vi "Beampointing_Multi_Pico2.vi"() -> ()   [LabVIEW 2013]
uses:
  GUI_Template/GUI_master/tcp_new_data_event.ctl
  GUI_Template/GUI_master/tcp new data cluster.ctl
  Ctrs/beam detection.ctl
  GUI_Beampointing_single_TRA/Ctrs/move.ctl
  <vilib>/Utility/file.llb/Read From Spreadsheet File (string).vi
  <userlib>/_OpenG.lib/array/array.llb/Filter 1D Array with Scalar (String)__ogtk.vi
  <userlib>/_OpenG.lib/array/array.llb/Filter 1D Array (String)__ogtk.vi
  <vilib>/Utility/file.llb/Write To Spreadsheet File (string).vi
  <vilib>/Analysis/NI_AALBase.lvlib
panel:
  out "x-y*floor(x/y)":dbl
  out "error out":errorcluster
  out "config path":string
  out "Array 3":bool[](array[boolean])
  out "Array 2":u16[](array[numeric])
  out "Array":u16[](array[numeric])
  out "Moving Y":string
  out "Moving X":string
  out "particles":T1(array[cluster])
  out "millisecond timer value":u32
  out "appended path":path
  out "millisecond timer 2":u32
  in  "GUIdevice 98":string="PicoPad4"
  in  "Position.Axis 111::98":dbl=77.0 caption="Motor Axis 1" min=-30000.0 max=30000.0 format="%#_6f"
  in  "Position.Axis 112::98":dbl=77.0 caption="Motor Axis 1" min=-20000.0 max=20000.0 format="%#_6f"
  in  "Position.Axis 113::98":dbl=77.0 caption="Motor Axis 1" min=-20000.0 max=20000.0 format="%#_6f"
  in  "Position.Axis 121::98":dbl=77.0 caption="Motor Axis 1" min=-999999.0 max=999999.0 format="%#_6f"
  in  "Position.Axis 122::98":dbl=77.0 caption="Motor Axis 1" min=-999999.0 max=999999.0 format="%#_6f"
  in  "Position.Axis 123::98":dbl=77.0 caption="Motor Axis 1" min=-999999.0 max=999999.0 format="%#_6f"
  in  "Position.Axis 131::98":dbl=77.0 caption="Motor Axis 1" min=-999999.0 max=999999.0 format="%#_6f"
  in  "Position.Axis 132::98":dbl=77.0 caption="Motor Axis 1" min=-999999.0 max=999999.0 format="%#_6f"
  in  "Position.Axis 133::98":dbl=77.0 caption="Motor Axis 1" min=-999999.0 max=999999.0 format="%#_6f"
  in  "Position.Axis 141::98":dbl=77.0 caption="Motor Axis 1" min=-999999.0 max=999999.0 format="%#_6f"
  in  "Position.Axis 142::98":dbl=77.0 caption="Motor Axis 1" min=-999999.0 max=999999.0 format="%#_6f"
  in  "Position.Axis 143::98":dbl=77.0 caption="Motor Axis 1" min=-999999.0 max=999999.0 format="%#_6f"
  in  "Position.Axis 211::98":dbl=77.0 caption="Motor Axis 1" min=-999999.0 max=999999.0 format="%#_6f"
  in  "Position.Axis 212::98":dbl=77.0 caption="Motor Axis 1" min=-999999.0 max=999999.0 format="%#_6f"
  in  "Position.Axis 213::98":dbl=77.0 caption="Motor Axis 1" min=-999999.0 max=999999.0 format="%#_6f"
  in  "Position.Axis 221::98":dbl=77.0 caption="Motor Axis 1" min=-999999.0 max=999999.0 format="%#_6f"
  in  "Position.Axis 222::98":dbl=77.0 caption="Motor Axis 1" min=-999999.0 max=999999.0 format="%#_6f"
  in  "Position.Axis 223::98":dbl=77.0 caption="Motor Axis 1" min=-999999.0 max=999999.0 format="%#_6f"
  in  "Position.Axis 231::98":dbl=77.0 caption="Motor Axis 1" min=-999999.0 max=999999.0 format="%#_6f"
  in  "Position.Axis 232::98":dbl=77.0 caption="Motor Axis 1" min=-999999.0 max=999999.0 format="%#_6f"
  in  "Position.Axis 233::98":dbl=77.0 caption="Motor Axis 1" min=-999999.0 max=999999.0 format="%#_6f"
  in  "Position.Axis 241::98":dbl=77.0 caption="Motor Axis 1" min=-999999.0 max=999999.0 format="%#_6f"
  in  "Position.Axis 242::98":dbl=77.0 caption="Motor Axis 1" min=-999999.0 max=999999.0 format="%#_6f"
  in  "Position.Axis 243::98":dbl=77.0 caption="Motor Axis 1" min=-999999.0 max=999999.0 format="%#_6f"
  in  "Position.Axis 311::98":dbl=77.0 caption="Motor Axis 1" min=-999999.0 max=999999.0 format="%#_6f"
  in  "Position.Axis 312::98":dbl=77.0 caption="Motor Axis 1" min=-999999.0 max=999999.0 format="%#_6f"
  in  "Position.Axis 313::98":dbl=77.0 caption="Motor Axis 1" min=-999999.0 max=999999.0 format="%#_6f"
  in  "Position.Axis 321::98":dbl=77.0 caption="Motor Axis 1" min=-999999.0 max=999999.0 format="%#_6f"
  in  "Position.Axis 322::98":dbl=77.0 caption="Motor Axis 1" min=-999999.0 max=999999.0 format="%#_6f"
  in  "Position.Axis 323::98":dbl=77.0 caption="Motor Axis 1" min=-999999.0 max=999999.0 format="%#_6f"
  in  "Position.Axis 331::98":dbl=77.0 caption="Motor Axis 1" min=-999999.0 max=999999.0 format="%#_6f"
  in  "Position.Axis 332::98":dbl=77.0 caption="Motor Axis 1" min=-999999.0 max=999999.0 format="%#_6f"
  in  "Position.Axis 333::98":dbl=77.0 caption="Motor Axis 1" min=-999999.0 max=999999.0 format="%#_6f"
  in  "Position.Axis 341::98":dbl=77.0 caption="Motor Axis 1" min=-999999.0 max=999999.0 format="%#_6f"
  in  "Position.Axis 342::98":dbl=77.0 caption="Motor Axis 1" min=-999999.0 max=999999.0 format="%#_6f"
  in  "Position.Axis 343::98":dbl=77.0 caption="Motor Axis 1" min=-999999.0 max=999999.0 format="%#_6f"
  in  "Position.Axis 411::98":dbl=77.0 caption="Motor Axis 1" min=-999999.0 max=999999.0 format="%#_6f"
  in  "Position.Axis 412::98":dbl=77.0 caption="Motor Axis 1" min=-999999.0 max=999999.0 format="%#_6f"
  in  "Position.Axis 413::98":dbl=77.0 caption="Motor Axis 1" min=-999999.0 max=999999.0 format="%#_6f"
  in  "Position.Axis 421::98":dbl=77.0 caption="Motor Axis 1" min=-999999.0 max=999999.0 format="%#_6f"
  in  "Position.Axis 422::98":dbl=77.0 caption="Motor Axis 1" min=-999999.0 max=999999.0 format="%#_6f"
  in  "Position.Axis 423::98":dbl=77.0 caption="Motor Axis 1" min=-999999.0 max=999999.0 format="%#_6f"
  in  "Position.Axis 431::98":dbl=77.0 caption="Motor Axis 1" min=-999999.0 max=999999.0 format="%#_6f"
  in  "Position.Axis 432::98":dbl=77.0 caption="Motor Axis 1" min=-999999.0 max=999999.0 format="%#_6f"
  in  "Position.Axis 433::98":dbl=77.0 caption="Motor Axis 1" min=-999999.0 max=999999.0 format="%#_6f"
  in  "Position.Axis 441::98":dbl=77.0 caption="Motor Axis 1" min=-999999.0 max=999999.0 format="%#_6f"
  in  "Position.Axis 442::98":dbl=77.0 caption="Motor Axis 1" min=-999999.0 max=999999.0 format="%#_6f"
  in  "Position.Axis 443::98":dbl=77.0 caption="Motor Axis 1" min=-999999.0 max=999999.0 format="%#_6f"
  in  "Position.Axis 511::98":dbl=77.0 caption="Motor Axis 1" min=-999999.0 max=999999.0 format="%#_6f"
  in  "Position.Axis 512::98":dbl=77.0 caption="Motor Axis 1" min=-999999.0 max=999999.0 format="%#_6f"
  in  "Position.Axis 513::98":dbl=77.0 caption="Motor Axis 1" min=-999999.0 max=999999.0 format="%#_6f"
  in  "Position.Axis 521::98":dbl=77.0 caption="Motor Axis 1" min=-999999.0 max=999999.0 format="%#_6f"
  in  "Position.Axis 522::98":dbl=77.0 caption="Motor Axis 1" min=-999999.0 max=999999.0 format="%#_6f"
  in  "Position.Axis 523::98":dbl=77.0 caption="Motor Axis 1" min=-999999.0 max=999999.0 format="%#_6f"
  in  "Position.Axis 531::98":dbl=77.0 caption="Motor Axis 1" min=-999999.0 max=999999.0 format="%#_6f"
  in  "Position.Axis 532::98":dbl=77.0 caption="Motor Axis 1" min=-999999.0 max=999999.0 format="%#_6f"
  in  "Position.Axis 533::98":dbl=77.0 caption="Motor Axis 1" min=-999999.0 max=999999.0 format="%#_6f"
  in  "Position.Axis 541::98":dbl=77.0 caption="Motor Axis 1" min=-999999.0 max=999999.0 format="%#_6f"
  in  "Position.Axis 542::98":dbl=77.0 caption="Motor Axis 1" min=-999999.0 max=999999.0 format="%#_6f"
  in  "Position.Axis 543::98":dbl=77.0 caption="Motor Axis 1" min=-999999.0 max=999999.0 format="%#_6f"
  in  "Numeric":dbl
  out "Current State":string
  in  "output cluster 2":T5 {"detection para"."smal para"."Measurement Parameter" items=["Center of Mass X", "Center of Mass Y", "First Pixel X", "First Pixel Y", "Bounding Rect Left", "Bounding Rect Top", "Bounding Rect Right", "Bounding Rect Bottom", "Max Feret Diameter Start X", "Max Feret Diameter Start Y", "Max Feret Diameter End X", "Max Feret Diameter End Y", "Max Horiz. Segment Length Left", "Max Horiz. Segment Length Right", "Max Horiz. Segment Length Row", "-", "Bounding Rect Width", "Bounding Rect Height", "Bounding Rect Diagonal", "Perimeter", "Convex Hull Perimeter", "Holes' Perimeter", "Max Feret Diameter", "Equivalent Ellipse Major Axis", "Equivalent Ellipse Minor Axis", "Equivalent Ellipse Minor Axis (Feret)", "Equivalent Rect Long Side", "Equivalent Rect Short Side", "Equivalent Rect Diagonal", "Equivalent Rect Short Side (Feret)", "Average Horiz. Segment Length", "Average Vert. Segment Length", "Hydraulic Radius", "Waddel Disk Diameter", "-", "Area", "Holes' Area", "Particle & Holes' Area", "Convex Hull Area", "Image Area", "-", "Number of Holes", "Number of Horiz. Segments", "Number of Vert. Segments", "-", "Orientation", "Max Feret Diameter Orientation", "-", "% Area/Image Area", "% Area/(Particle & Holes' Area)", "Ratio of Equivalent Ellipse Axes", "Ratio of Equivalent Rect Sides", "-", "Elongation Factor", "Compactness Factor", "Heywood Circularity Factor", "Type Factor", "-", "Sum X", "Sum Y", "Sum XX", "Sum XY", "Sum YY", "Sum XXX", "Sum XXY", "Sum XYY", "Sum YYY", "-", "Moment of Inertia XX", "Moment of Inertia XY", "Moment of Inertia YY", "Moment of Inertia XXX", "Moment of Inertia XXY", "Moment of Inertia XYY", "Moment of Inertia YYY", "Norm. Moment of Inertia XX", "Norm. Moment of Inertia XY", "Norm. Moment of Inertia YY", "Norm. Moment of Inertia XXX", "Norm. Moment of Inertia XXY", "Norm. Moment of Inertia XYY", "Norm. Moment of Inertia YYY", "Hu Moment 1", "Hu Moment 2", "Hu Moment 3", "Hu Moment 4", "Hu Moment 5", "Hu Moment 6", "Hu Moment 7"]; "detection para"."smal para"."Range Lower Value" format="%.2f"; "detection para"."smal para"."Range Upper Value" format="%.2f"; "detection para"."detection method" items=["clustering", "entropy", "metric", "moments", "inter-class variance"]; "detection para"."Filter" items=["No Filter", "Median Filter", "Low Pass Filter"]}
  out "CCDs":string[](array[string])
  in  "GUIdevice 12":string
  in  "GUIdevice 11":string
  in  "GUIdevice 10":string
  in  "GUIdevice 9":string
  out "error out 2":errorcluster
  in  "active cams":string[](array[string])
  in  "Motor Y":dbl[][](array[numeric])
  in  "Motor X":dbl[][](array[numeric])
  out "Names":string[](array[string])
  in  "Offset X stats":dbl[][](array[numeric])
  in  "Offset Y stats":dbl[][](array[numeric])
  out "Box":T6(array[cluster])
  in  "Tab Control 2":enum32{"Config ", "Main", "History"}(tab)=enum."Main"
  out "Waveform Chart":u32(graph)
  in  "associated motors":T7
  out "Cameras":T8
  out "Status":cluster{i32, i32, "Centroid X":dbl[][]}(graph)
  out "image::9":T9(plugin-control) caption="L8_M10Leak"
  out "image::6":T9(plugin-control) caption="L5_TREXPass2"
  in  "Exposure:12":dbl=0.095 min=0.0001 max=1.0 format="%#_6f"
  in  "Triggerdelay::12":dbl=0.003 min=0.0 max=0.09 format="%#_6f"
  in  "Exposure::11":dbl=0.095 min=0.0001 max=1.0 format="%#_6f"
  in  "Triggerdelay::11":dbl=0.003 min=0.0 max=0.09 format="%#_6f"
  in  "Exposure::10":dbl=0.095 min=0.0001 max=1.0 format="%#_6f"
  in  "Triggerdelay::10":dbl=0.003 min=0.0 max=0.09 format="%#_6f"
  in  "Exposure::9":dbl=0.095 min=0.0001 max=1.0 format="%#_6f"
  in  "Triggerdelay::9":dbl=0.003 min=0.0 max=0.09 format="%#_6f"
  in  "Trigger::9":bool
  in  "Trigger::10":bool caption="Trigger:10"
  in  "Trigger::11":bool
  in  "Trigger::12":bool
  in  "Target.Y::9":dbl=45.0 caption="T9y" min=0.0 max=2000.0 format="%#_6f"
  in  "Target.X::9":dbl=47.0 caption="Tx9" min=0.0 max=2000.0 format="%#_6f"
  in  "Target.Y::10":dbl=45.0 caption="T10y" min=0.0 max=2000.0 format="%#_6f"
  in  "Target.X::10":dbl=47.0 caption="T10x" min=0.0 max=2000.0 format="%#_6f"
  in  "Target.Y::11":dbl=45.0 caption="T11y" min=0.0 max=2000.0 format="%#_6f"
  in  "Target.X::11":dbl=47.0 caption="T11x" min=0.0 max=2000.0 format="%#_6f"
  in  "Target.Y::12":dbl=45.0 caption="T12y" min=0.0 max=2000.0 format="%#_6f"
  in  "Target.X::12":dbl=47.0 caption="T12x" min=0.0 max=2000.0 format="%#_6f"
  in  "Exposure::8":dbl=0.095 min=0.01 max=1.0 format="%#_6f"
  in  "Triggerdelay::8":dbl=0.003 min=0.0 max=0.09 format="%#_6f"
  in  "Trigger::8":bool
  in  "Target.Y::8":dbl=45.0 caption="T8y" min=0.0 max=2000.0 format="%#_6f"
  in  "Target.X::8":dbl=47.0 caption="T8x" min=0.0 max=2000.0 format="%#_6f"
  in  "Target.Y::7":dbl=45.0 caption="T7x" min=0.0 max=2000.0 format="%#_6f"
  in  "Target.X::7":dbl=47.0 caption="T7y" min=0.0 max=2000.0 format="%#_6f"
  in  "Target.Y::6":dbl=45.0 caption="T6y" min=0.0 max=2000.0 format="%#_6f"
  in  "Target.X::6":dbl=47.0 caption="T6x" min=0.0 max=2000.0 format="%#_6f"
  in  "Target.Y::5":dbl=45.0 caption="T5y" min=0.0 max=2000.0 format="%#_6f"
  in  "Target.X::5":dbl=47.0 caption="T5x" min=0.0 max=2000.0 format="%#_6f"
  in  "Target.Y::4":dbl=45.0 caption="T4y" min=0.0 max=2000.0 format="%#_6f"
  in  "Target.X::4":dbl=47.0 caption="T4x" min=0.0 max=2000.0 format="%#_6f"
  in  "Target.Y::3":dbl=163.0 caption="T3y" min=0.0 max=2000.0 format="%#_6f"
  in  "Target.X::3":dbl=152.0 caption="T3x" min=0.0 max=2000.0 format="%#_6f"
  in  "Target.Y::2":dbl=74.0 caption="T2y" min=1.0 max=600.0 format="%#_6f"
  in  "Target.X::2":dbl=75.0 caption="T2x" min=1.0 max=800.0 format="%#_6f"
  in  "Target.Y::1":dbl=61.0 caption="T1y" min=1.0 max=600.0 format="%#_6f"
  in  "Target.X::1":dbl=77.0 caption="T1x" min=1.0 max=800.0 format="%#_6f"
  in  "Exposure::7":dbl=0.095 min=0.0001 max=1.0 format="%#_6f"
  in  "Triggerdelay::7":dbl=0.003 min=0.0 max=0.09 format="%#_6f"
  in  "Trigger::7":bool
  in  "Exposure::6":dbl=0.095 min=0.0001 max=1.0 format="%#_6f"
  in  "Triggerdelay::6":dbl=0.003 min=0.0 max=0.09 format="%#_6f"
  in  "Trigger::6":bool
  in  "Exposure::5":dbl=0.095 min=0.0001 max=1.0 format="%#_6f"
  in  "Triggerdelay::5":dbl=0.003 min=0.0 max=0.09 format="%#_6f"
  in  "Trigger::5":bool
  in  "Exposure::4":dbl=0.095 min=0.0001 max=1.0 format="%#_6f"
  in  "Triggerdelay::4":dbl=0.003 min=0.0 max=0.09 format="%#_6f"
  in  "Trigger::4":bool
  in  "Exposure::3":dbl=0.095 min=0.0001 max=1.0 format="%#_6f"
  in  "Triggerdelay::3":dbl=0.003 min=0.0 max=0.09 format="%#_6f"
  in  "Trigger::3":bool
  in  "Exposure::2":dbl=0.095 min=0.0001 max=1.0 format="%#_6f"
  in  "Triggerdelay::2":dbl=0.003 min=0.0 max=0.09 format="%#_6f"
  in  "Trigger::2":bool
  out "image::1":T9(plugin-control) caption="PA2_Input1"
  out "image::2":T9(plugin-control) caption="PA2_Input2"
  out "image::3":T9(plugin-control) caption="L1_TelInpNear"
  out "image::4":T9(plugin-control) caption="L2_TelInpFar"
  out "image::5":T9(plugin-control) caption="L4_TREXpass1"
  out "image::7":T9(plugin-control) caption="L6_TREXpass3"
  out "image::8":T9(plugin-control) caption="L7_TREXPass4"
  in  "Exposure::1":dbl=0.095 min=0.0001 max=1.0 format="%#_6f"
  in  "Triggerdelay::1":dbl=0.003 min=0.0 max=0.09 format="%#_6f"
  in  "Trigger::1":bool
  in  "UDP error message":string
  out "required Y":bool[](array[boolean])
  out "required X":bool[](array[boolean])
  out "detected":bool[](array[boolean])
  out "name array":string[](array[string])
  out "image::10":T9(plugin-control) caption="B1_TelInput"
  out "image::11":T9(plugin-control) caption="B2_TelLens1"
  out "image::12":T9(plugin-control) caption="B3_TelLens2"
  out "speedmode X":bool[](array[boolean])
  out "speedmode Y":bool[](array[boolean])
  out "CCD 9":cluster{timestamp[], dbl[]}[](graph)
  out "CCD 10":cluster{timestamp[], dbl[]}[](graph)
  out "CCD 11":cluster{timestamp[], dbl[]}[](graph)
  out "CCD 12":cluster{timestamp[], dbl[]}[](graph)
  out "CCD 5":cluster{timestamp[], dbl[]}[](graph)
  out "CCD 6":cluster{timestamp[], dbl[]}[](graph)
  out "CCD 7":cluster{timestamp[], dbl[]}[](graph)
  out "CCD 8":cluster{timestamp[], dbl[]}[](graph)
  out "CCD 2":cluster{timestamp[], dbl[]}[](graph)
  out "CCD 1":cluster{timestamp[], dbl[]}[](graph)
  out "CCD 3":cluster{timestamp[], dbl[]}[](graph)
  out "CCD 4":cluster{timestamp[], dbl[]}[](graph)
  out "History index":i32
  in  "History Size":i32=500
  out "Particle Reports (Pixels)":T10(array[cluster])
  in  "Feedback Global":bool
  in  "detection para":T3[](array[typedef])=[{"Filter"=1, "Filter Para"={"X Size"=5, "Y Size"=5, "% Tolerance"=1}, "detection method"=4, "smal para"=[{"Measurement Parameter"=35, "Range Lower Value"=0.0, "Range Upper Value"=0.0, "Range"=TRUE, "Measurement Type"=FALSE}], "Remove small Objects"=TRUE, "Restrict to round Objects"=FALSE}, {"Filter"=1, "Filter Para"={"X Size"=5, "Y Size"=5, "% Tolerance"=1}, "detection method"=4, "smal para"=[{"Measurement Parameter"=35, "Range Lower Value"=0.0, "Range Upper Value"=500.0, "Range"=FALSE, "Measurement Type"=FALSE}], "Remove small Objects"=TRUE, "Restrict to round Objects"=FALSE}, {"Filter"=1, "Filter Para"={"X Size"=5, "Y Size"=5, "% Tolerance"=1}, "detection method"=4, "smal para"=[{"Measurement Parameter"=35, "Range Lower Value"=0.0, "Range Upper Value"=500.0, "Range"=TRUE, "Measurement Type"=FALSE}], "Remove small Objects"=TRUE, "Restrict to round Objects"=FALSE}, {"Filter"=1, "Filter Para"={"X Size"=5, "Y Size"=5, "% Tolerance"=1}, "detection method"=4, "smal para"=[{"Measurement Parameter"=35, "Range Lower Value"=0.0, "Range Upper Value"=500.0, "Range"=TRUE, "Measurement Type"=FALSE}], "Remove small Objects"=TRUE, "Restrict to round Objects"=FALSE}, {"Filter"=1, "Filter Para"={"X Size"=5, "Y Size"=5, "% Tolerance"=1}, "detection method"=4, "smal para"=[{"Measurement Parameter"=35, "Range Lower Value"=0.0, "Range Upper Value"=500.0, "Range"=TRUE, "Measurement Type"=FALSE}], "Remove small Objects"=TRUE, "Restrict to round Objects"=FALSE}, {"Filter"=1, "Filter Para"={"X Size"=5, "Y Size"=5, "% Tolerance"=1}, "detection method"=4, "smal para"=[{"Measurement Parameter"=35, "Range Lower Value"=0.0, "Range Upper Value"=500.0, "Range"=TRUE, "Measurement Type"=FALSE}], "Remove small Objects"=TRUE, "Restrict to round Objects"=FALSE}, {"Filter"=1, "Filter Para"={"X Size"=5, "Y Size"=5, "% Tolerance"=1}, "detection method"=4, "smal para"=[{"Measurement Parameter"=35, "Range Lower Value"=0.0, "Range Upper Value"=500.0, "Range"=TRUE, "Measurement Type"=FALSE}], "Remove small Objects"=TRUE, "Restrict to round Objects"=FALSE}, {"Filter"=1, "Filter Para"={"X Size"=5, "Y Size"=5, "% Tolerance"=1}, "detection method"=3, "smal para"=[{"Measurement Parameter"=35, "Range Lower Value"=0.0, "Range Upper Value"=0.0, "Range"=FALSE, "Measurement Type"=FALSE}], "Remove small Objects"=TRUE, "Restrict to round Objects"=FALSE}, {"Filter"=1, "Filter Para"={"X Size"=5, "Y Size"=5, "% Tolerance"=1}, "detection method"=4, "smal para"=[{"Measurement Parameter"=35, "Range Lower Value"=0.0, "Range Upper Value"=0.0, "Range"=FALSE, "Measurement Type"=FALSE}], "Remove small Objects"=TRUE, "Restrict to round Objects"=FALSE}, {"Filter"=1, "Filter Para"={"X Size"=5, "Y Size"=5, "% Tolerance"=1}, "detection method"=4, "smal para"=[{"Measurement Parameter"=35, "Range Lower Value"=0.0, "Range Upper Value"=500.0, "Range"=TRUE, "Measurement Type"=FALSE}], "Remove small Objects"=TRUE, "Restrict to round Objects"=FALSE}, {"Filter"=1, "Filter Para"={"X Size"=5, "Y Size"=5, "% Tolerance"=1}, "detection method"=4, "smal para"=[{"Measurement Parameter"=35, "Range Lower Value"=0.0, "Range Upper Value"=500.0, "Range"=TRUE, "Measurement Type"=FALSE}], "Remove small Objects"=TRUE, "Restrict to round Objects"=FALSE}, {"Filter"=1, "Filter Para"={"X Size"=5, "Y Size"=5, "% Tolerance"=1}, "detection method"=4, "smal para"=[{"Measurement Parameter"=35, "Range Lower Value"=0.0, "Range Upper Value"=500.0, "Range"=TRUE, "Measurement Type"=FALSE}], "Remove small Objects"=TRUE, "Restrict to round Objects"=FALSE}] {"smal para"."Measurement Parameter" items=["Center of Mass X", "Center of Mass Y", "First Pixel X", "First Pixel Y", "Bounding Rect Left", "Bounding Rect Top", "Bounding Rect Right", "Bounding Rect Bottom", "Max Feret Diameter Start X", "Max Feret Diameter Start Y", "Max Feret Diameter End X", "Max Feret Diameter End Y", "Max Horiz. Segment Length Left", "Max Horiz. Segment Length Right", "Max Horiz. Segment Length Row", "-", "Bounding Rect Width", "Bounding Rect Height", "Bounding Rect Diagonal", "Perimeter", "Convex Hull Perimeter", "Holes' Perimeter", "Max Feret Diameter", "Equivalent Ellipse Major Axis", "Equivalent Ellipse Minor Axis", "Equivalent Ellipse Minor Axis (Feret)", "Equivalent Rect Long Side", "Equivalent Rect Short Side", "Equivalent Rect Diagonal", "Equivalent Rect Short Side (Feret)", "Average Horiz. Segment Length", "Average Vert. Segment Length", "Hydraulic Radius", "Waddel Disk Diameter", "-", "Area", "Holes' Area", "Particle & Holes' Area", "Convex Hull Area", "Image Area", "-", "Number of Holes", "Number of Horiz. Segments", "Number of Vert. Segments", "-", "Orientation", "Max Feret Diameter Orientation", "-", "% Area/Image Area", "% Area/(Particle & Holes' Area)", "Ratio of Equivalent Ellipse Axes", "Ratio of Equivalent Rect Sides", "-", "Elongation Factor", "Compactness Factor", "Heywood Circularity Factor", "Type Factor", "-", "Sum X", "Sum Y", "Sum XX", "Sum XY", "Sum YY", "Sum XXX", "Sum XXY", "Sum XYY", "Sum YYY", "-", "Moment of Inertia XX", "Moment of Inertia XY", "Moment of Inertia YY", "Moment of Inertia XXX", "Moment of Inertia XXY", "Moment of Inertia XYY", "Moment of Inertia YYY", "Norm. Moment of Inertia XX", "Norm. Moment of Inertia XY", "Norm. Moment of Inertia YY", "Norm. Moment of Inertia XXX", "Norm. Moment of Inertia XXY", "Norm. Moment of Inertia XYY", "Norm. Moment of Inertia YYY", "Hu Moment 1", "Hu Moment 2", "Hu Moment 3", "Hu Moment 4", "Hu Moment 5", "Hu Moment 6", "Hu Moment 7"]; "smal para"."Range Lower Value" format="%.2f"; "smal para"."Range Upper Value" format="%.2f"; "detection method" items=["clustering", "entropy", "metric", "moments", "inter-class variance"]; "Filter" items=["No Filter", "Median Filter", "Low Pass Filter"]}
  in  "GUIdevice 8":string="B5_CompressorOut"
  in  "Tab Control":T11(tab)
  in  "Center":bool
  in  "Save Stats":bool
  in  "Save Config":bool
  in  "Load Config":bool
  in  "update speed [ms]":i32=200
  in  "Img to avg":i32=20 min=3 max=200 step=1
  in  "Reset History":bool
  in  "save path":path=path "W:/BP_DATA"
  in  "autodetect":bool
  in  "Detection Rate":dbl=0.8 min=0.001 max=1.0
  in  "new tdms":bool
  in  "Speedmode @":dbl=3.0 min=1.0 max=20.0
  in  "Align":bool
  in  "deivice ini":bool
  in  "beam detection para":T3={"Filter"=1, "Filter Para"={"X Size"=5, "Y Size"=5, "% Tolerance"=1}, "detection method"=4, "smal para"=[{"Measurement Parameter"=35, "Range Lower Value"=0.0, "Range Upper Value"=500.0, "Range"=FALSE, "Measurement Type"=FALSE}], "Remove small Objects"=TRUE, "Restrict to round Objects"=FALSE} {"smal para"."Measurement Parameter" items=["Center of Mass X", "Center of Mass Y", "First Pixel X", "First Pixel Y", "Bounding Rect Left", "Bounding Rect Top", "Bounding Rect Right", "Bounding Rect Bottom", "Max Feret Diameter Start X", "Max Feret Diameter Start Y", "Max Feret Diameter End X", "Max Feret Diameter End Y", "Max Horiz. Segment Length Left", "Max Horiz. Segment Length Right", "Max Horiz. Segment Length Row", "-", "Bounding Rect Width", "Bounding Rect Height", "Bounding Rect Diagonal", "Perimeter", "Convex Hull Perimeter", "Holes' Perimeter", "Max Feret Diameter", "Equivalent Ellipse Major Axis", "Equivalent Ellipse Minor Axis", "Equivalent Ellipse Minor Axis (Feret)", "Equivalent Rect Long Side", "Equivalent Rect Short Side", "Equivalent Rect Diagonal", "Equivalent Rect Short Side (Feret)", "Average Horiz. Segment Length", "Average Vert. Segment Length", "Hydraulic Radius", "Waddel Disk Diameter", "-", "Area", "Holes' Area", "Particle & Holes' Area", "Convex Hull Area", "Image Area", "-", "Number of Holes", "Number of Horiz. Segments", "Number of Vert. Segments", "-", "Orientation", "Max Feret Diameter Orientation", "-", "% Area/Image Area", "% Area/(Particle & Holes' Area)", "Ratio of Equivalent Ellipse Axes", "Ratio of Equivalent Rect Sides", "-", "Elongation Factor", "Compactness Factor", "Heywood Circularity Factor", "Type Factor", "-", "Sum X", "Sum Y", "Sum XX", "Sum XY", "Sum YY", "Sum XXX", "Sum XXY", "Sum XYY", "Sum YYY", "-", "Moment of Inertia XX", "Moment of Inertia XY", "Moment of Inertia YY", "Moment of Inertia XXX", "Moment of Inertia XXY", "Moment of Inertia XYY", "Moment of Inertia YYY", "Norm. Moment of Inertia XX", "Norm. Moment of Inertia XY", "Norm. Moment of Inertia YY", "Norm. Moment of Inertia XXX", "Norm. Moment of Inertia XXY", "Norm. Moment of Inertia XYY", "Norm. Moment of Inertia YYY", "Hu Moment 1", "Hu Moment 2", "Hu Moment 3", "Hu Moment 4", "Hu Moment 5", "Hu Moment 6", "Hu Moment 7"]; "smal para"."Range Lower Value" format="%.2f"; "smal para"."Range Upper Value" format="%.2f"; "detection method" items=["clustering", "entropy", "metric", "moments", "inter-class variance"]; "Filter" items=["No Filter", "Median Filter", "Low Pass Filter"]}
  in  "move config":T2={"Tolerance [%]"=0.1, "Stepsize"=0.0001, "Invert Axis"=TRUE, "Invert Direction X"=FALSE, "Invert Direction Y"=TRUE, "enable feedback"=FALSE, "Set Centriod Target"=FALSE}
  in  "ActiveMotor":u16(ring)=7 items=["PA2_Input1", "PA2_Input2", "L2_TelInpFar", "L1_TelInpNear", "L4_TREXPASS1", "L5_TREXPass2", "L6_TREXPass3", "L7_TREXPass4", "L8_M10Leak", "B1_TelInput", "B2_TelLens1", "NoName", "NoName", "NoName", "MBeamSplitterL", "Mdiode", "NoName", "NoName", "NoName", "NoName"]
  in  "ActiveMotorName::99":string
  in  "RelativeMove.Axis 1.CCW::99":bool caption="RelativeMove.Axis 1.CCW::1"
  in  "RelativeMove.Axis 1.CW::99":bool caption="RelativeMove.Axis 1.CW::1"
  in  "RelativeMove.Axis 2.CCW::99":bool caption="RelativeMove.Axis. 2.CCW::1"
  in  "RelativeMove.Axis 2.CW::99":bool caption="RelativeMove.Axis 2.CW::1"
  in  "RelativeSettings.Axis 1.Position::99":dbl caption="Axis 1 Position" min=-999999.0 max=999999.0 format="%_4p"
  in  "RelativeSettings.Axis 2.Position::99":dbl caption="Axis 2 Position" min=-999999.0 max=999999.0 format="%_4p"
  in  "RelativeSettings.Axis 2.StepSize::99":dbl=50.0 caption="Axis 2 StepSize" min=0.0 max=999999.0 format="%_4p"
  in  "RelativeSettings.Axis 1.StepSize::99":dbl=50.0 caption="Axis 1 Stepsize" min=0.0 max=999999.0 format="%_4p"
  out "Arguments Y":string
  in  "active axis refs 2":T12(array[cluster])
  in  "active Axis ref":cluster{"Ref X":refnum<vi>, "Ref Y":refnum<vi>}
  in  "CCDs":u16(ring) items=["PA2_Input1", "PA2_Input2", "L1_TelInpNear", "L2_TelInpFar", "L4_TREXpass1", "L5_TREXPass2", "L6_TREXpass3", "L7_TREXPass4", "L8_M10Leak", "B1_TelInput", "B2_TelLens1", "B3_TelLens2"]
  out "motor refs":refnum<vi>[](array[refnum])
  in  "Position.Axis 511::99":dbl=77.0 caption="Motor Axis 1" min=-20000.0 max=20000.0 format="%#_6f"
  in  "Position.Axis 512::99":dbl=77.0 caption="Motor Axis 1" min=-20000.0 max=20000.0 format="%#_6f"
  in  "Position.Axis 513::99":dbl=77.0 caption="Motor Axis 1" min=-20000.0 max=20000.0 format="%#_6f"
  in  "Position.Axis 521::99":dbl=77.0 caption="Motor Axis 1" min=-20000.0 max=20000.0 format="%#_6f"
  in  "Position.Axis 522::99":dbl=77.0 caption="Motor Axis 1" min=-20000.0 max=20000.0 format="%#_6f"
  in  "Position.Axis 523::99":dbl=77.0 caption="Motor Axis 1" min=-20000.0 max=20000.0 format="%#_6f"
  in  "Position.Axis 531::99":dbl=77.0 caption="Motor Axis 1" min=-20000.0 max=20000.0 format="%#_6f"
  in  "Position.Axis 532::99":dbl=77.0 caption="Motor Axis 1" min=-20000.0 max=20000.0 format="%#_6f"
  in  "Position.Axis 533::99":dbl=77.0 caption="Motor Axis 1" min=-20000.0 max=20000.0 format="%#_6f"
  in  "Position.Axis 541::99":dbl=77.0 caption="Motor Axis 1" min=-20000.0 max=20000.0 format="%#_6f"
  in  "Position.Axis 542::99":dbl=77.0 caption="Motor Axis 1" min=-20000.0 max=20000.0 format="%#_6f"
  in  "Position.Axis 543::99":dbl=77.0 caption="Motor Axis 1" min=-20000.0 max=20000.0 format="%#_6f"
  in  "Position.Axis 411::99":dbl=77.0 caption="Motor Axis 1" min=-20000.0 max=20000.0 format="%#_6f"
  in  "Position.Axis 412::99":dbl=77.0 caption="Motor Axis 1" min=-20000.0 max=20000.0 format="%#_6f"
  in  "Position.Axis 413::99":dbl=77.0 caption="Motor Axis 1" min=-20000.0 max=20000.0 format="%#_6f"
  in  "Position.Axis 421::99":dbl=77.0 caption="Motor Axis 1" min=-20000.0 max=20000.0 format="%#_6f"
  in  "Position.Axis 422::99":dbl=77.0 caption="Motor Axis 1" min=-20000.0 max=20000.0 format="%#_6f"
  in  "Position.Axis 423::99":dbl=77.0 caption="Motor Axis 1" min=-20000.0 max=20000.0 format="%#_6f"
  in  "Position.Axis 431::99":dbl=77.0 caption="Motor Axis 1" min=-20000.0 max=20000.0 format="%#_6f"
  in  "Position.Axis 432::99":dbl=77.0 caption="Motor Axis 1" min=-20000.0 max=20000.0 format="%#_6f"
  in  "Position.Axis 433::99":dbl=77.0 caption="Motor Axis 1" min=-20000.0 max=20000.0 format="%#_6f"
  in  "Position.Axis 441::99":dbl=77.0 caption="Motor Axis 1" min=-20000.0 max=20000.0 format="%#_6f"
  in  "Position.Axis 442::99":dbl=77.0 caption="Motor Axis 1" min=-20000.0 max=20000.0 format="%#_6f"
  in  "Position.Axis 443::99":dbl=77.0 caption="Motor Axis 1" min=-20000.0 max=20000.0 format="%#_6f"
  in  "Position.Axis 311::99":dbl=77.0 caption="Motor Axis 1" min=-50000.0 max=50000.0 format="%#_6f"
  in  "Position.Axis 312::99":dbl=77.0 caption="Motor Axis 1" min=-50000.0 max=50000.0 format="%#_6f"
  in  "Position.Axis 313::99":dbl=77.0 caption="Motor Axis 1" min=-999999.0 max=999999.0 format="%#_6f"
  in  "Position.Axis 321::99":dbl=77.0 caption="Motor Axis 1" min=-20000.0 max=20000.0 format="%#_6f"
  in  "Position.Axis 322::99":dbl=77.0 caption="Motor Axis 1" min=-20000.0 max=20000.0 format="%#_6f"
  in  "Position.Axis 323::99":dbl=77.0 caption="Motor Axis 1" min=-20000.0 max=20000.0 format="%#_6f"
  in  "Position.Axis 331::99":dbl=77.0 caption="Motor Axis 1" min=-20000.0 max=20000.0 format="%#_6f"
  in  "Position.Axis 332::99":dbl=77.0 caption="Motor Axis 1" min=-20000.0 max=20000.0 format="%#_6f"
  in  "Position.Axis 333::99":dbl=77.0 caption="Motor Axis 1" min=-20000.0 max=20000.0 format="%#_6f"
  in  "Position.Axis 341::99":dbl=77.0 caption="Motor Axis 1" min=-20000.0 max=20000.0 format="%#_6f"
  in  "Position.Axis 342::99":dbl=77.0 caption="Motor Axis 1" min=-20000.0 max=20000.0 format="%#_6f"
  in  "Position.Axis 343::99":dbl=77.0 caption="Motor Axis 1" min=-20000.0 max=20000.0 format="%#_6f"
  in  "Position.Axis 241::99":dbl=77.0 caption="Motor Axis 1" min=-20000.0 max=20000.0 format="%#_6f"
  in  "Position.Axis 242::99":dbl=77.0 caption="Motor Axis 1" min=-20000.0 max=20000.0 format="%#_6f"
  in  "Position.Axis 243::99":dbl=77.0 caption="Motor Axis 1" min=-20000.0 max=20000.0 format="%#_6f"
  in  "Position.Axis 231::99":dbl=77.0 caption="Motor Axis 1" min=-20000.0 max=20000.0 format="%#_6f"
  in  "Position.Axis 232::99":dbl=77.0 caption="Motor Axis 1" min=-20000.0 max=20000.0 format="%#_6f"
  in  "Position.Axis 233::99":dbl=77.0 caption="Motor Axis 1" min=-20000.0 max=20000.0 format="%#_6f"
  in  "Position.Axis 221::99":dbl=77.0 caption="Motor Axis 1" min=-20000.0 max=20000.0 format="%#_6f"
  in  "Position.Axis 222::99":dbl=77.0 caption="Motor Axis 1" min=-20000.0 max=200000.0 format="%#_6f"
  in  "Position.Axis 223::99":dbl=77.0 caption="Motor Axis 1" min=-20000.0 max=20000.0 format="%#_6f"
  in  "Position.Axis 211::99":dbl=77.0 caption="Motor Axis 1" min=-20000.0 max=200000.0 format="%#_6f"
  in  "Position.Axis 212::99":dbl=77.0 caption="Motor Axis 1" min=-20000.0 max=20000.0 format="%#_6f"
  in  "Position.Axis 213::99":dbl=77.0 caption="Motor Axis 1" min=-20000.0 max=20000.0 format="%#_6f"
  in  "Position.Axis 141::99":dbl=77.0 caption="Motor Axis 1" min=-20000.0 max=20000.0 format="%#_6f"
  in  "Position.Axis 142::99":dbl=77.0 caption="Motor Axis 1" min=-20000.0 max=20000.0 format="%#_6f"
  in  "Position.Axis 143::99":dbl=77.0 caption="Motor Axis 1" min=-20000.0 max=20000.0 format="%#_6f"
  in  "Position.Axis 131::99":dbl=77.0 caption="Motor Axis 1" min=-20000.0 max=20000.0 format="%#_6f"
  in  "Position.Axis 132::99":dbl=77.0 caption="Motor Axis 1" min=-20000.0 max=20000.0 format="%#_6f"
  in  "Position.Axis 133::99":dbl=77.0 caption="Motor Axis 1" min=-20000.0 max=20000.0 format="%#_6f"
  in  "Position.Axis 121::99":dbl=77.0 caption="Motor Axis 1" min=-20000.0 max=20000.0 format="%#_6f"
  in  "Position.Axis 122::99":dbl=77.0 caption="Motor Axis 1" min=-20000.0 max=20000.0 format="%#_6f"
  in  "Position.Axis 123::99":dbl=77.0 caption="Motor Axis 1" min=-20000.0 max=20000.0 format="%#_6f"
  in  "Position.Axis 113::99":dbl=77.0 caption="Motor Axis 1" min=-20000.0 max=20000.0 format="%#_6f"
  in  "Position.Axis 112::99":dbl=77.0 caption="Motor Axis 1" min=-20000.0 max=20000.0 format="%#_6f"
  in  "Position.Axis 111::99":dbl=77.0 caption="Motor Axis 1" min=-20000.0 max=20000.0 format="%#_6f"
  out "Arguments X":string
  in  "GUIdevice 99":string="PicoPad3"
  in  "move properties":T2[](array[typedef])=[{"Tolerance [%]"=0.1, "Stepsize"=0.0001, "Invert Axis"=TRUE, "Invert Direction X"=FALSE, "Invert Direction Y"=TRUE, "enable feedback"=FALSE, "Set Centriod Target"=FALSE}, {"Tolerance [%]"=0.1, "Stepsize"=0.0001, "Invert Axis"=TRUE, "Invert Direction X"=FALSE, "Invert Direction Y"=TRUE, "enable feedback"=FALSE, "Set Centriod Target"=FALSE}, {"Tolerance [%]"=0.1, "Stepsize"=0.0001, "Invert Axis"=TRUE, "Invert Direction X"=FALSE, "Invert Direction Y"=TRUE, "enable feedback"=FALSE, "Set Centriod Target"=FALSE}, {"Tolerance [%]"=0.1, "Stepsize"=0.0001, "Invert Axis"=TRUE, "Invert Direction X"=FALSE, "Invert Direction Y"=TRUE, "enable feedback"=FALSE, "Set Centriod Target"=FALSE}, {"Tolerance [%]"=0.1, "Stepsize"=0.0001, "Invert Axis"=TRUE, "Invert Direction X"=FALSE, "Invert Direction Y"=TRUE, "enable feedback"=FALSE, "Set Centriod Target"=FALSE}, {"Tolerance [%]"=0.1, "Stepsize"=0.0001, "Invert Axis"=TRUE, "Invert Direction X"=FALSE, "Invert Direction Y"=TRUE, "enable feedback"=FALSE, "Set Centriod Target"=FALSE}, {"Tolerance [%]"=0.1, "Stepsize"=0.0001, "Invert Axis"=TRUE, "Invert Direction X"=FALSE, "Invert Direction Y"=TRUE, "enable feedback"=FALSE, "Set Centriod Target"=FALSE}, {"Tolerance [%]"=0.1, "Stepsize"=0.0001, "Invert Axis"=TRUE, "Invert Direction X"=FALSE, "Invert Direction Y"=TRUE, "enable feedback"=FALSE, "Set Centriod Target"=FALSE}, {"Tolerance [%]"=0.1, "Stepsize"=0.0001, "Invert Axis"=TRUE, "Invert Direction X"=FALSE, "Invert Direction Y"=TRUE, "enable feedback"=FALSE, "Set Centriod Target"=FALSE}, {"Tolerance [%]"=0.1, "Stepsize"=0.0001, "Invert Axis"=TRUE, "Invert Direction X"=FALSE, "Invert Direction Y"=TRUE, "enable feedback"=FALSE, "Set Centriod Target"=FALSE}, {"Tolerance [%]"=0.1, "Stepsize"=0.0001, "Invert Axis"=TRUE, "Invert Direction X"=FALSE, "Invert Direction Y"=TRUE, "enable feedback"=FALSE, "Set Centriod Target"=FALSE}, {"Tolerance [%]"=0.1, "Stepsize"=0.0001, "Invert Axis"=TRUE, "Invert Direction X"=FALSE, "Invert Direction Y"=TRUE, "enable feedback"=FALSE, "Set Centriod Target"=FALSE}, {"Tolerance [%]"=0.1, "Stepsize"=0.0001, "Invert Axis"=TRUE, "Invert Direction X"=FALSE, "Invert Direction Y"=TRUE, "enable feedback"=FALSE, "Set Centriod Target"=FALSE}]
  in  "Time":timestamp[][](array[timestamp])
  in  "Mean Size":dbl[][](array[numeric])
  in  "Size":dbl[][](array[numeric])
  in  "active CCDs":i32(listbox)=1
  in  "Offset Y":dbl[][](array[numeric])
  in  "Offset X":dbl[][](array[numeric])
  in  "Mean Centroid X":dbl[][](array[numeric])
  in  "Mean Centroid Y":dbl[][](array[numeric])
  in  "Centroid Y":dbl[][](array[numeric])
  in  "Centroid X":dbl[][](array[numeric])
  in  "GUIdevice 7":string="B2_TelLens1"
  in  "GUIdevice 6":string="B1_TelInput"
  in  "GUIdevice 5":string="L8_M10Leak"
  in  "GUIdevice 4":string="L7_TREXPass4"
  in  "GUIdevice 3":string="L6_TREXpass3"
  in  "GUIdevice 2":string="L5_TREXPass2"
  in  "insert tag":bool=TRUE
  in  "stop":bool
  in  "GUIdevice 1":string="L4_TREXpass1"
  out "tcp data event":T13
  out "error IO 2":errorcluster
  # "x [Tolerance]"
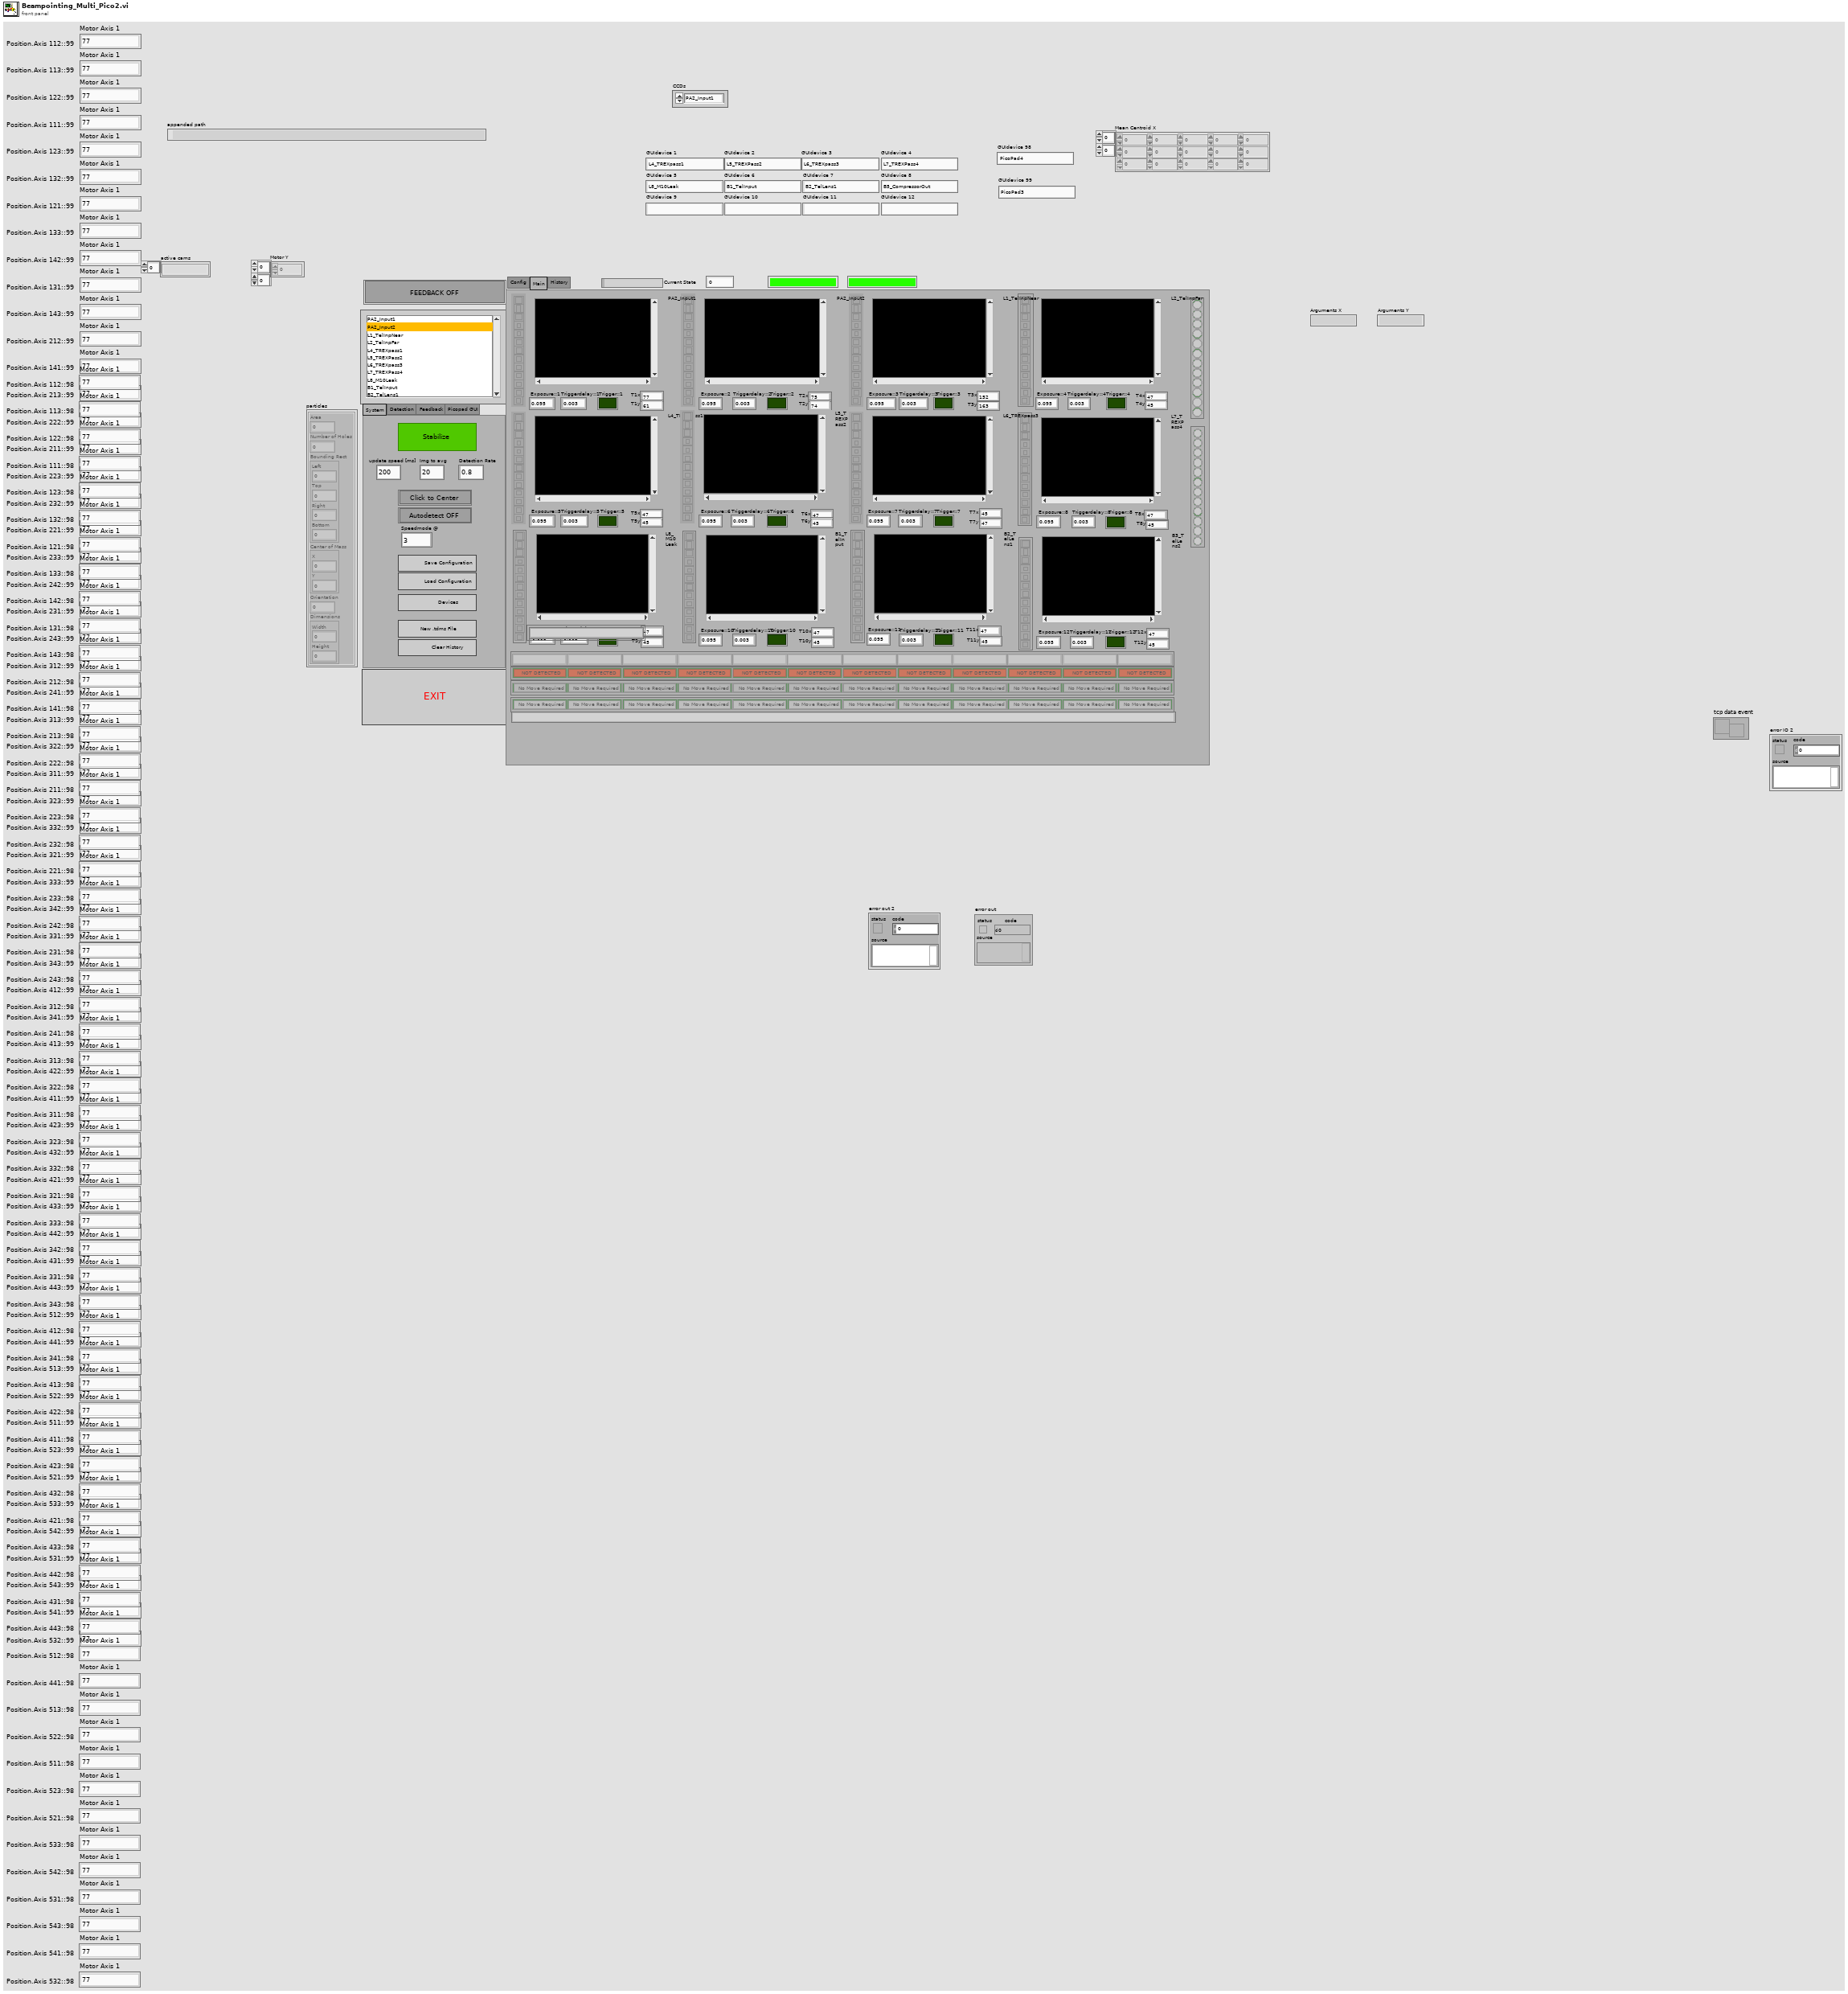
[diagram p1: front panel]
types:
  T1 = cluster{"Area":dbl, "Number of Holes":dbl, "Bounding Rect":cluster{"Left":dbl, "Top":dbl, "Right":dbl, "Bottom":dbl}, "Center of Mass":cluster{"X":dbl, "Y":dbl}, "Orientation":dbl, "Dimensions":cluster{"Width":dbl, "Height":dbl}}[]
  T2 = typedef "move.ctl" = cluster{"Tolerance [%]":dbl, "Stepsize":dbl, "Invert Axis":bool, "Invert Direction X":bool, "Invert Direction Y":bool, "enable feedback":bool, "Set Centriod Target":bool}
  T3 = typedef "beam detection.ctl" = cluster{"Filter":u16, "Filter Para":cluster{"X Size":i32, "Y Size":i32, "% Tolerance":i32}, "detection method":i32, "smal para":cluster{"Measurement Parameter":T4, "Range Lower Value":dbl, "Range Upper Value":dbl, "Range":bool, "Measurement Type":bool}[], "Remove small Objects":bool, "Restrict to round Objects":bool}
  T4 = typedef "Particle Parameters" = i32
  T5 = cluster{"CCDs":string[], "move properties":T2[], "detection para":T3[], "thresholds":cluster{"Lower value":sgl, "Upper value":sgl}[], "Value":cluster{"Motor CCD 1":u16, "Motor CCD 2":u16, "Motor CCD 3":u16, "Motor CCD 4":u16, "Motor CCD 5":u16, "Motor CCD 6":u16, "Motor CCD 7":u16, "Motor CCD 8":u16, "Motor CCD 9":u16, "Motor CCD 10":u16, "Motor CCD 11":u16, "Motor CCD 12":u16}}
  T6 = cluster{"Left":dbl, "Top":dbl, "Right":dbl, "Bottom":dbl}[]
  T7 = cluster{"Motor CCD 1":u16, "Motor CCD 2":u16, "Motor CCD 3":u16, "Motor CCD 4":u16, "Motor CCD 5":u16, "Motor CCD 6":u16, "Motor CCD 7":u16, "Motor CCD 8":u16, "Motor CCD 9":u16, "Motor CCD 10":u16, "Motor CCD 11":u16, "Motor CCD 12":u16}
  T8 = cluster{"[0]":string, "[1]":string, "[2]":string, "[3]":string, "[4]":string, "[5]":string, "[6]":string, "[7]":string, "[8]":string, "[8] 2":string, "[8] 3":string, "[8] 4":string}
  T9 = typedef "IMAQ Image.ctl" = refnum<image>
  T10 = cluster{"Area":dbl, "Number of Holes":dbl, "Bounding Rect":cluster{"Left":dbl, "Top":dbl, "Right":dbl, "Bottom":dbl}, "Center of Mass":cluster{"X":dbl, "Y":dbl}, "Orientation":dbl, "Dimensions":cluster{"Width":dbl, "Height":dbl}}[][]
  T11 = enum32{"System", "Detection", "Feedback", "Picopad GUI"}
  T12 = cluster{"Ref X":refnum<vi>, "Ref Y":refnum<vi>}[]
  T13 = typedef "tcp_new_data_event.ctl" = refnum<user-event>
  T14 = typedef "tcp new data cluster.ctl" = cluster{"EventEnum":enum16{"new data", "connection status update"}, "Device name":string}
  T15 = cluster{"Left":i32, "Top":i32, "Right":i32, "Bottom":i32}
  T16 = enum32{"invalid app kind", "Development System", "Run Time System", "Student Edition", "Embedded LabVIEW", "Evaluation", "Custom"}
  T17 = enum16{"open", "open or create", "create or replace", "create", "open (read-only)"}
  T18 = enum32{"Invalid", "Standard", "Closed", "Hidden", "Minimized", "Maximized"}
  T19 = enum16{"open", "replace", "create", "open or create", "replace or create", "replace or create with confirmation"}
  T20 = typedef "Image Type" = u32
  T21 = cluster{"[0]":string, "[1]":string, "[2]":string, "[3]":string, "[4]":string, "[5]":string, "[6]":string, "[7]":string, "[8]":string, "[9]":string, "[10]":string, "[11]":string}
  T22 = cluster{"Target.X::1":refnum<vi>, "Target.Y::1":refnum<vi>}
  T23 = cluster{"Target.X::2":refnum<vi>, "Target.Y::2":refnum<vi>}
  T24 = cluster{"Target.X::3":refnum<vi>, "Target.Y::3":refnum<vi>}
  T25 = cluster{"Target.X::4":refnum<vi>, "Target.Y::4":refnum<vi>}
  T26 = cluster{"Target.X::5":refnum<vi>, "Target.Y::5":refnum<vi>}
  T27 = cluster{"Target.X::6":refnum<vi>, "Target.Y::6":refnum<vi>}
  T28 = cluster{"Target.X::7":refnum<vi>, "Target.Y::7":refnum<vi>}
  T29 = cluster{"Target.X::8":refnum<vi>, "Target.Y::8":refnum<vi>}
  T30 = cluster{"Target.X::12":refnum<vi>, "Target.Y::12":refnum<vi>}
  T31 = cluster{"Target.X::9":refnum<vi>, "Target.Y::9":refnum<vi>}
  T32 = cluster{"Target.X::10":refnum<vi>, "Target.Y::10":refnum<vi>}
  T33 = cluster{"Target.X::11":refnum<vi>, "Target.Y::11":refnum<vi>}
  T34 = cluster{"Target.X::12":refnum<vi>, "Target.Y::12":refnum<vi>}[]
  T35 = cluster{"Left":dbl, "Top":dbl, "Right":dbl, "Bottom":dbl}
  T36 = cluster{"Core":cluster{"Current VI Reference":refnum<vi>, "Close Panel on Exit?":bool}, "detection para":T3[], "thresholds":cluster{"Lower value":sgl, "Upper value":sgl}[], "Centroid X":dbl[][], "Centroid Y":dbl[][], "img to avg":i32, "Mean Centroid X":dbl[][], "Mean Centroid Y":dbl[][], "Offset X":dbl[][], "Offset Y":dbl[][], "Offset X stats ":dbl[][], "Offset Y stats ":dbl[][], "Size":dbl[][], "Mean Size":dbl[][], "Time":timestamp[][], "move properties":T2[], "active axis refs 2":cluster{"Ref X":refnum<vi>, "Ref Y":refnum<vi>}[], "active ccd":i32, "Feedback global":bool, "Motor X":dbl[][], "Motor Y":dbl[][], "active cams":string[], "Data Value Reference out":refnum<k34>, "detected":bool[], "speedmode X":bool[], "speedmode Y":bool[]}
  T37 = cluster{"Current VI Reference":refnum<vi>, "Close Panel on Exit?":bool}
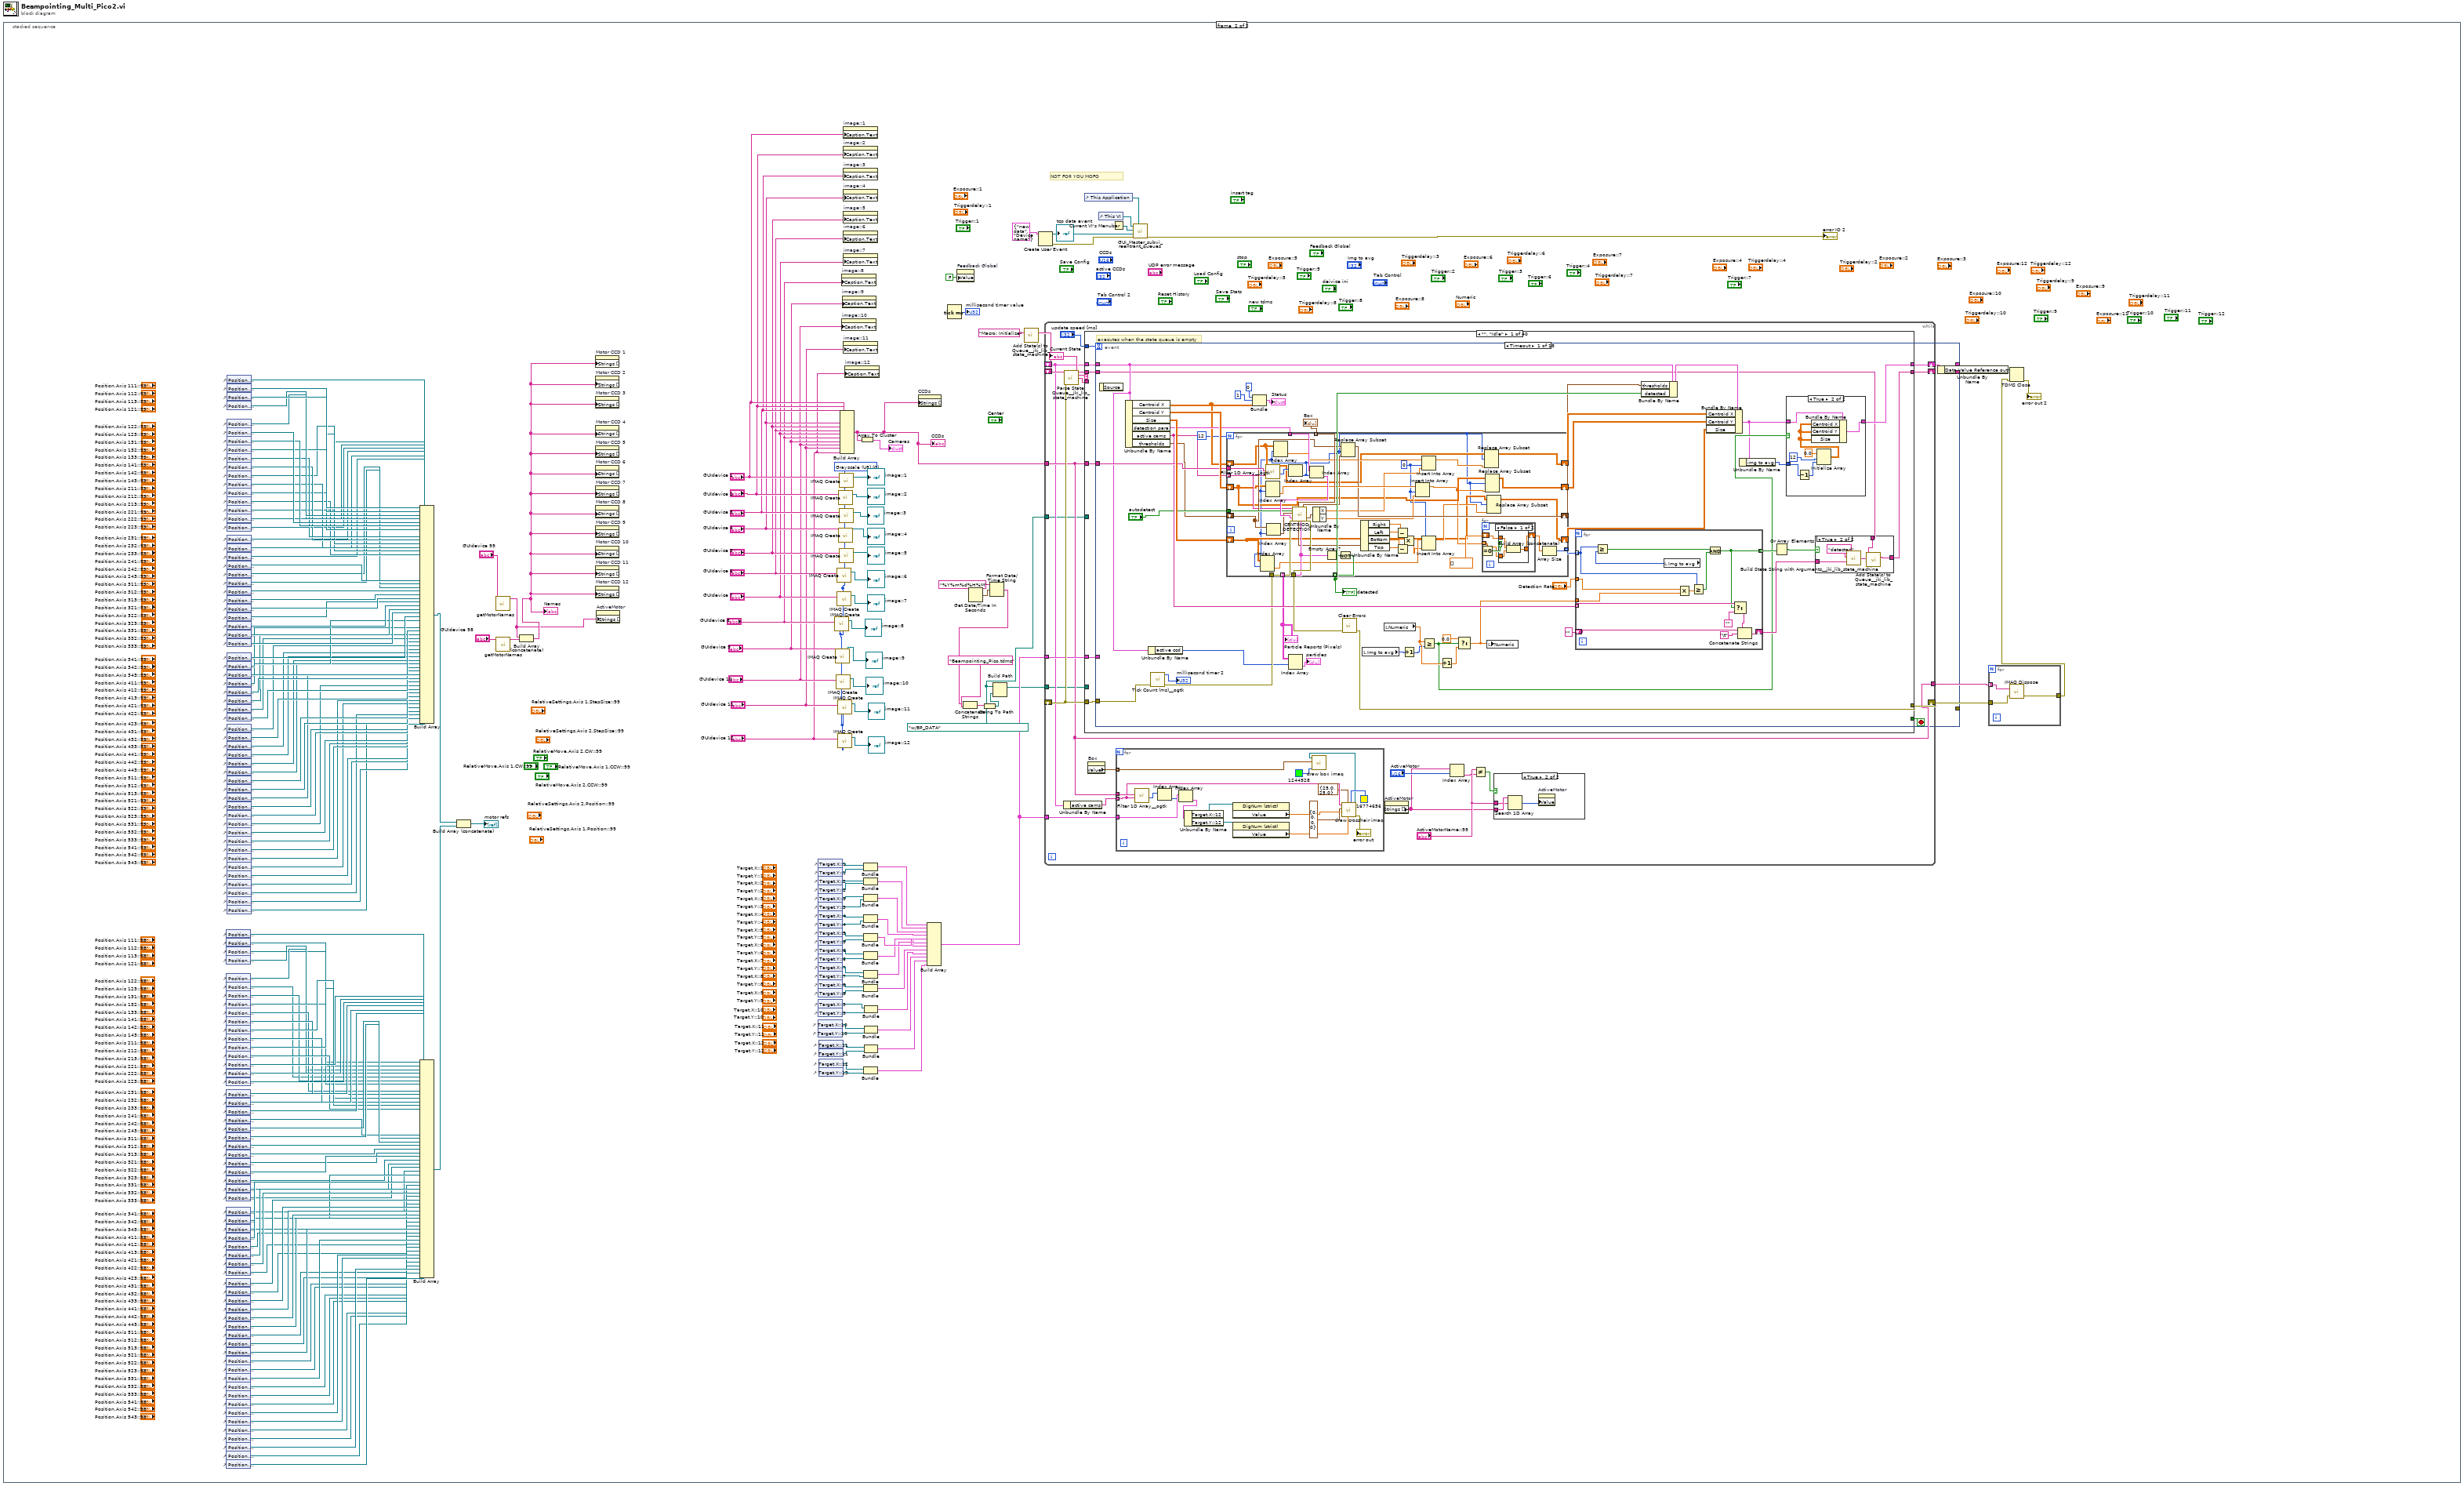
[diagram p0: block diagram]
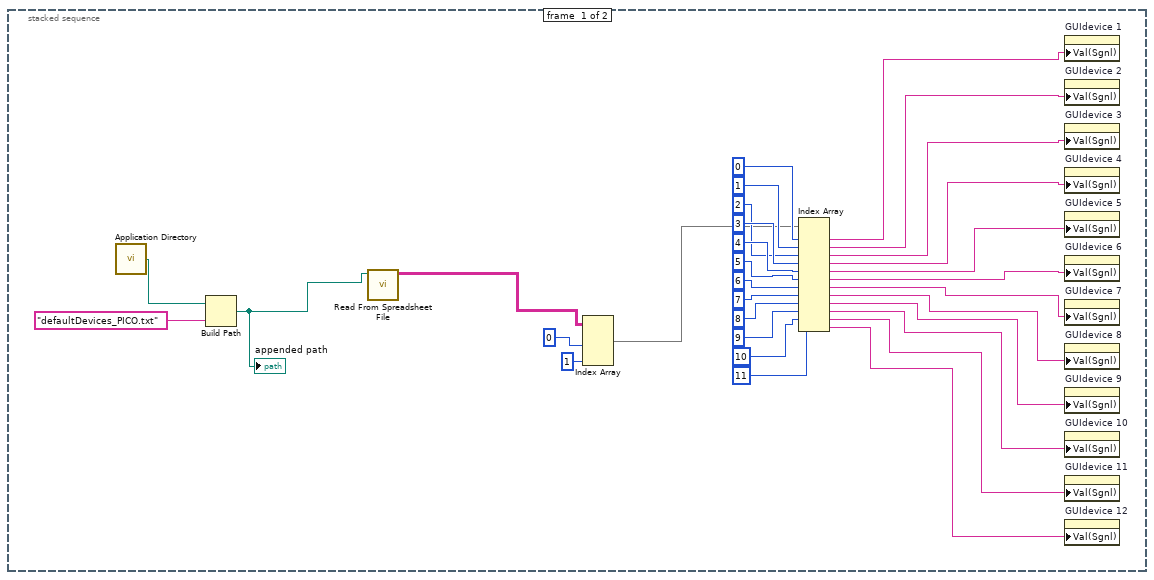
[diagram p2: hidden frame]
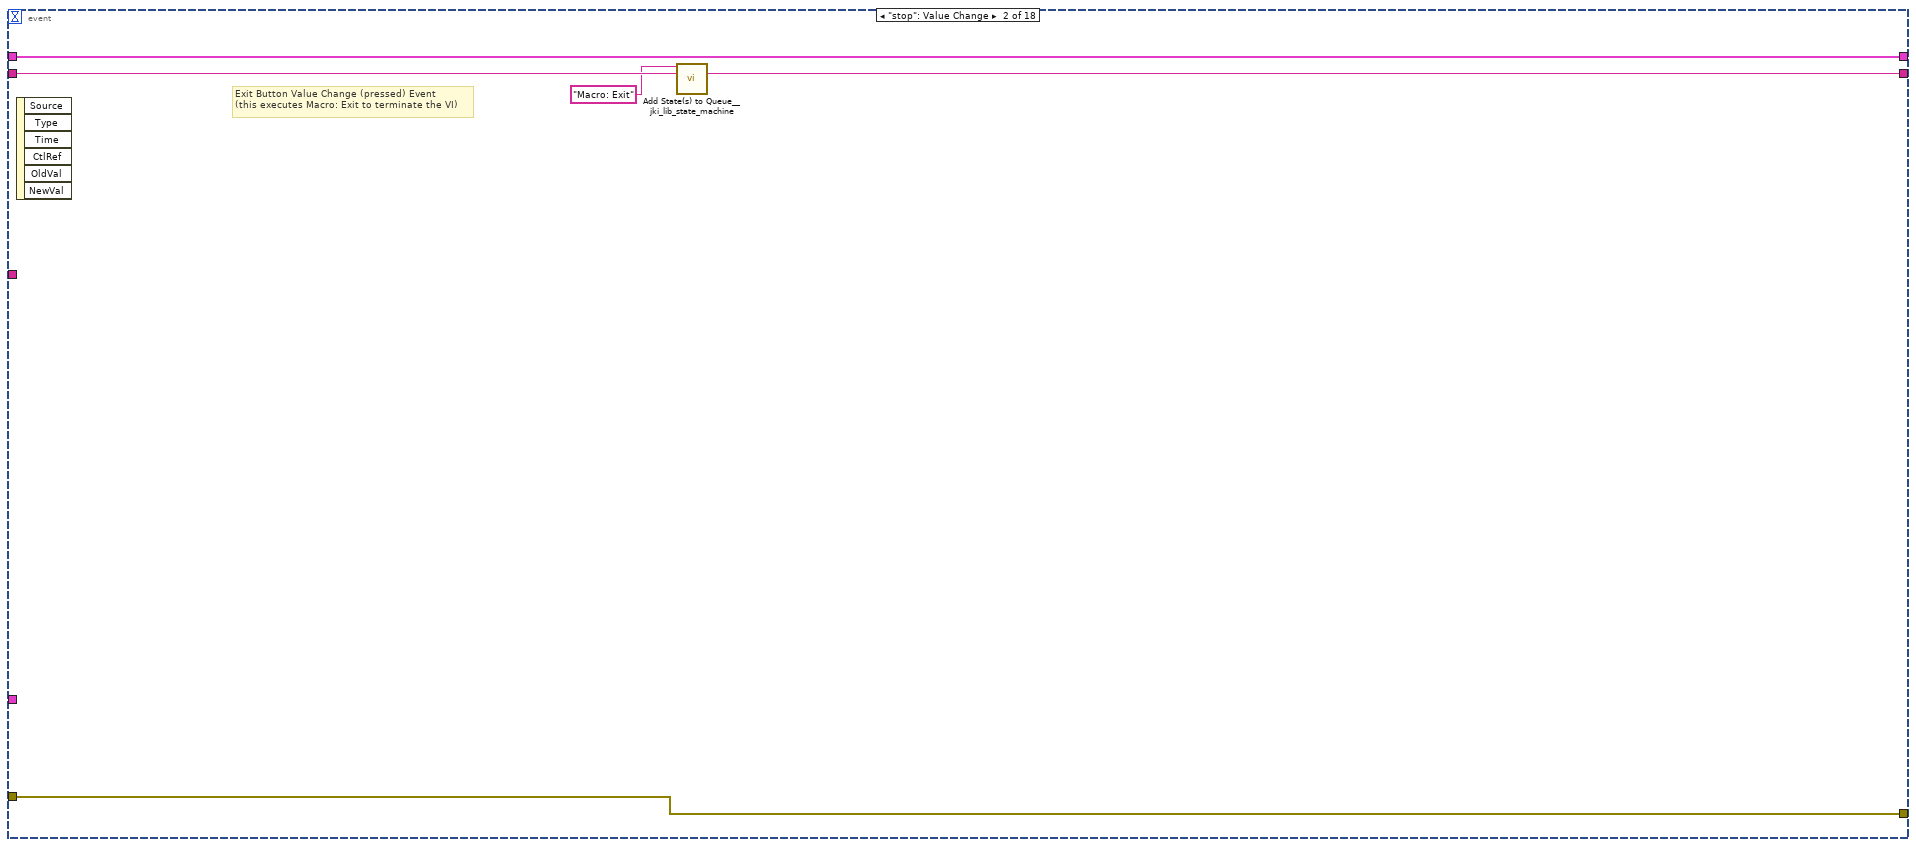
[diagram p7: hidden frame]
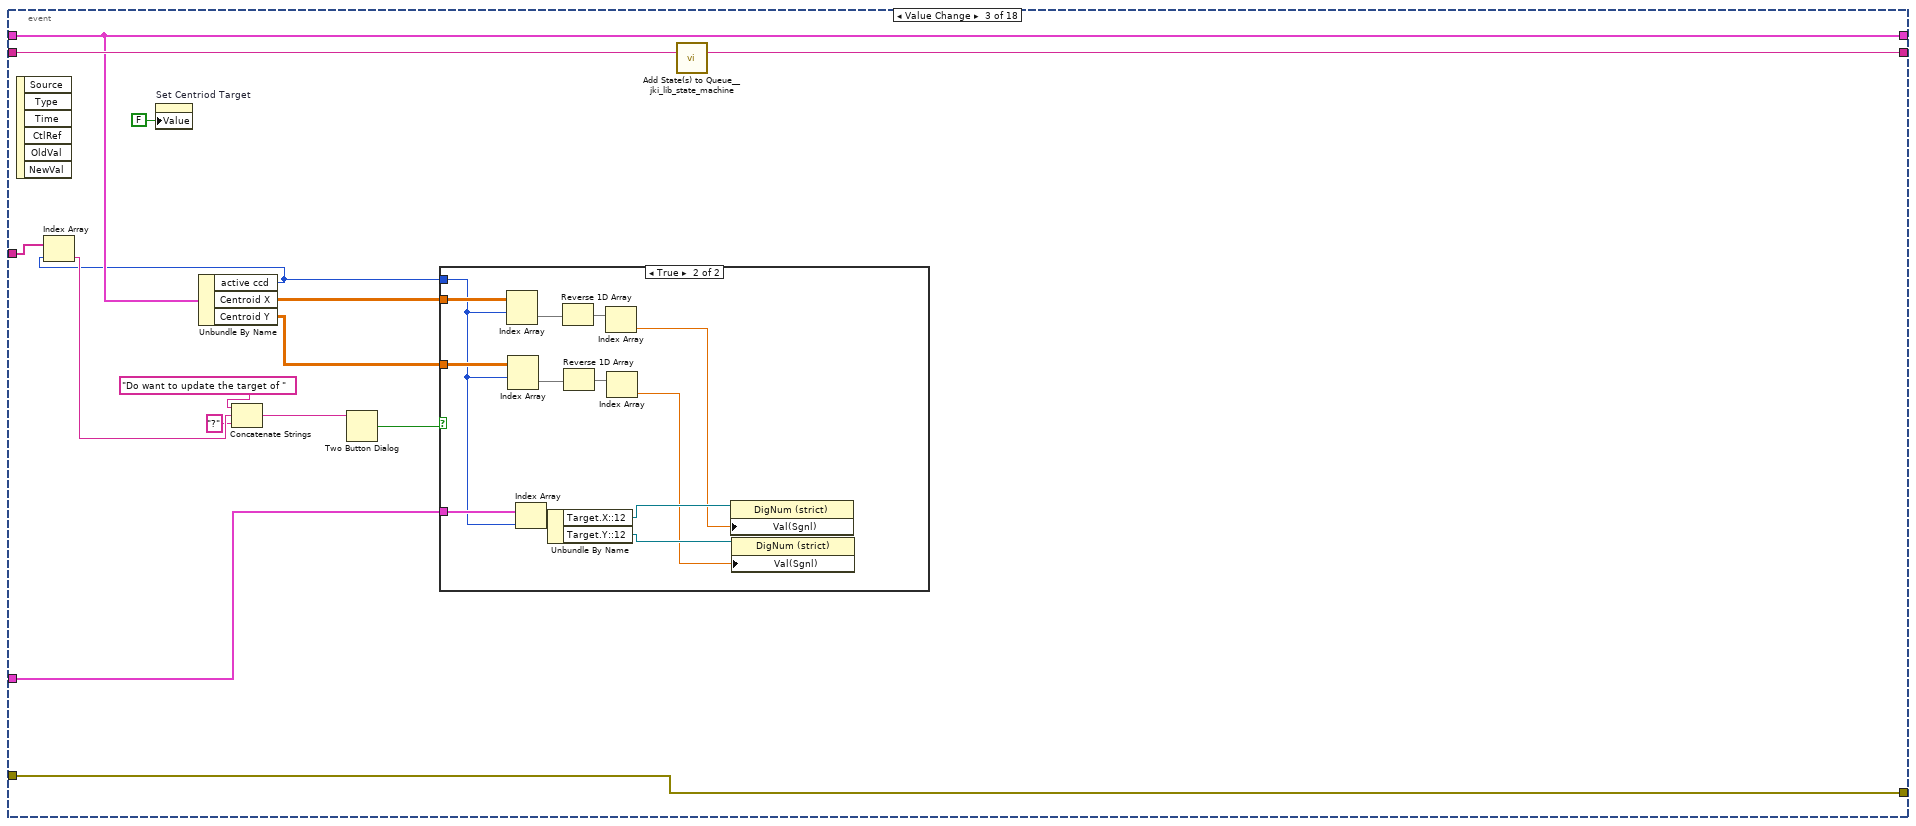
[diagram p8: hidden frame]
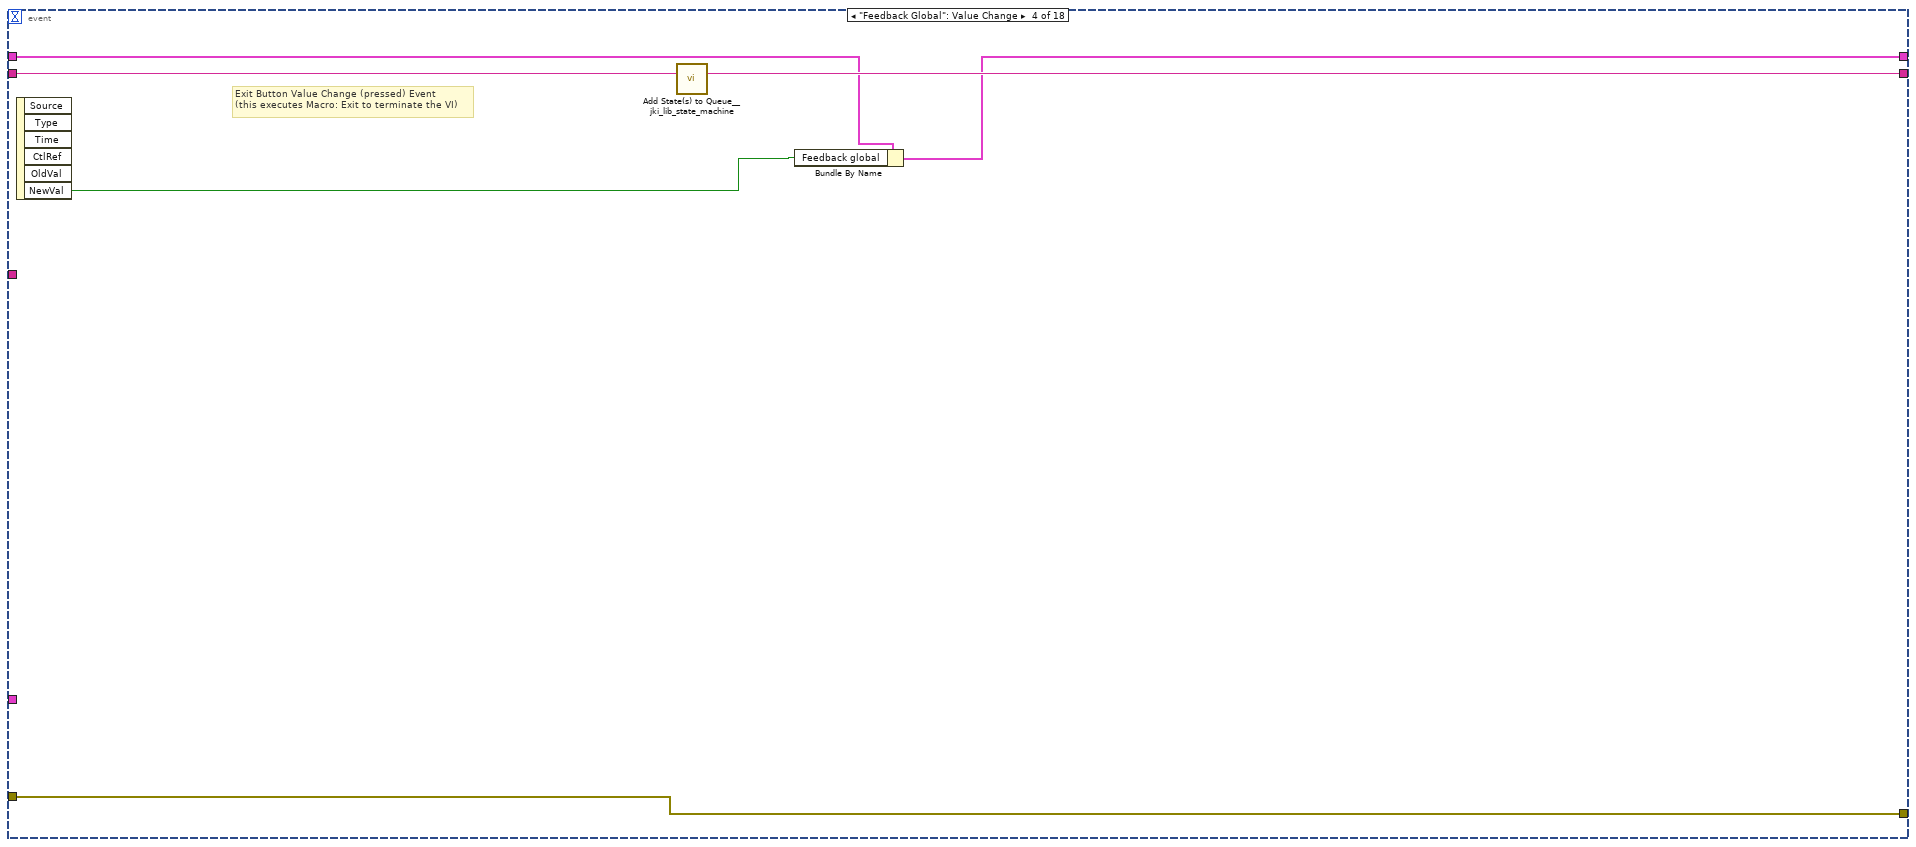
[diagram p10: hidden frame]
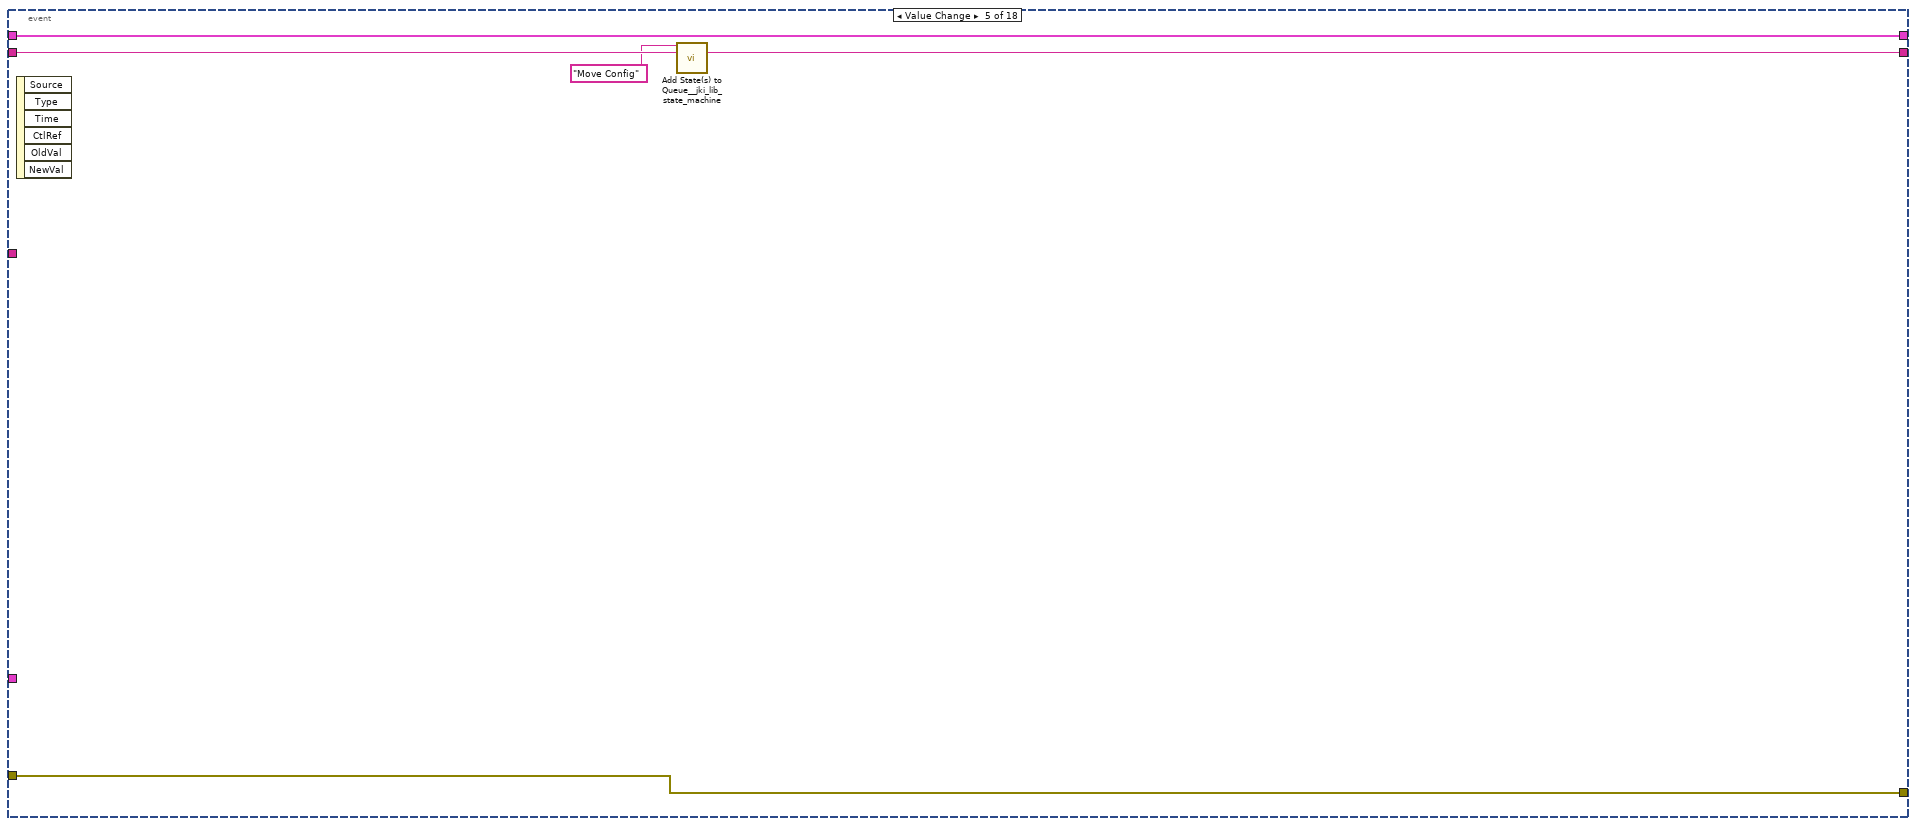
[diagram p11: hidden frame]
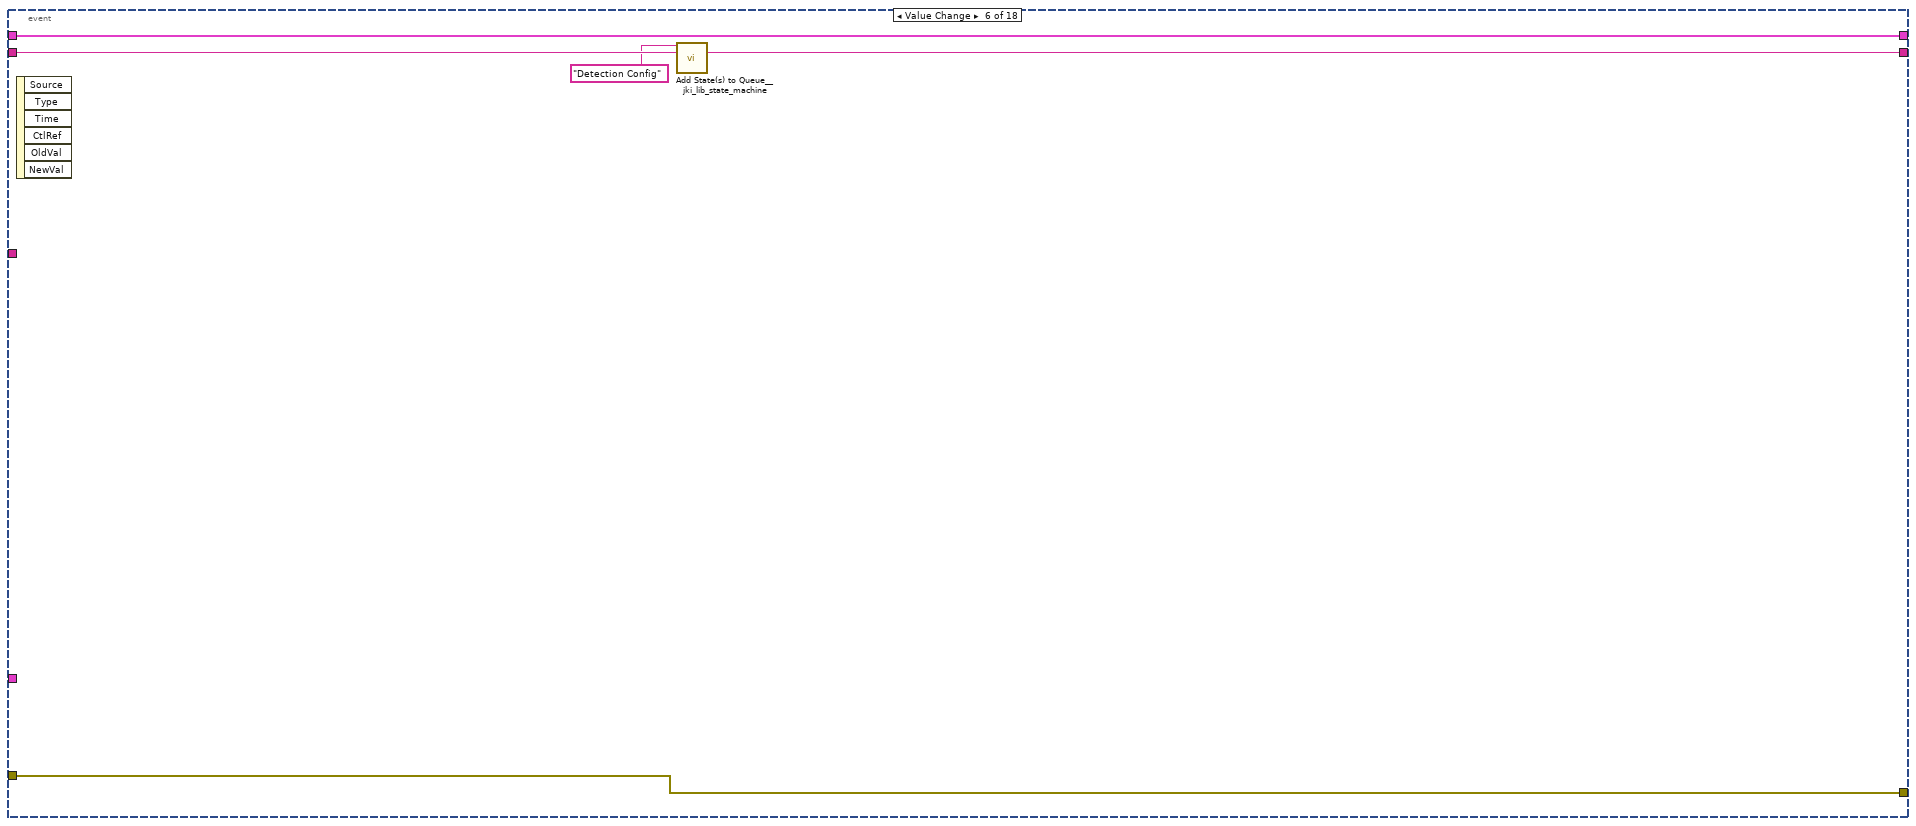
[diagram p12: hidden frame]
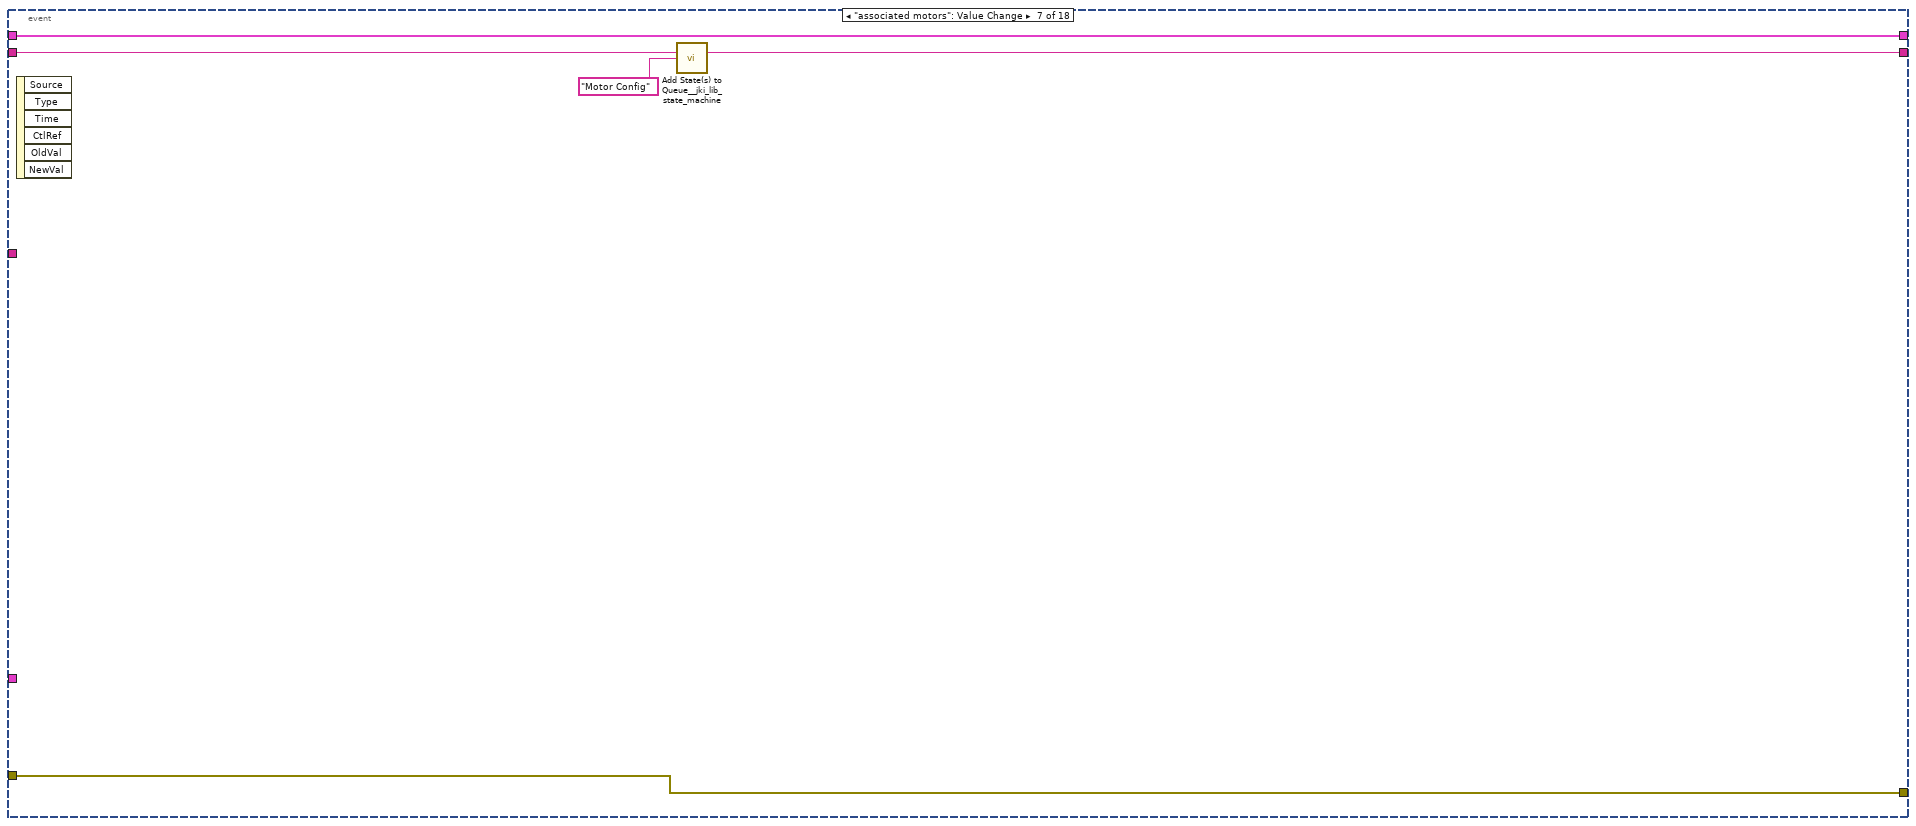
[diagram p13: hidden frame]
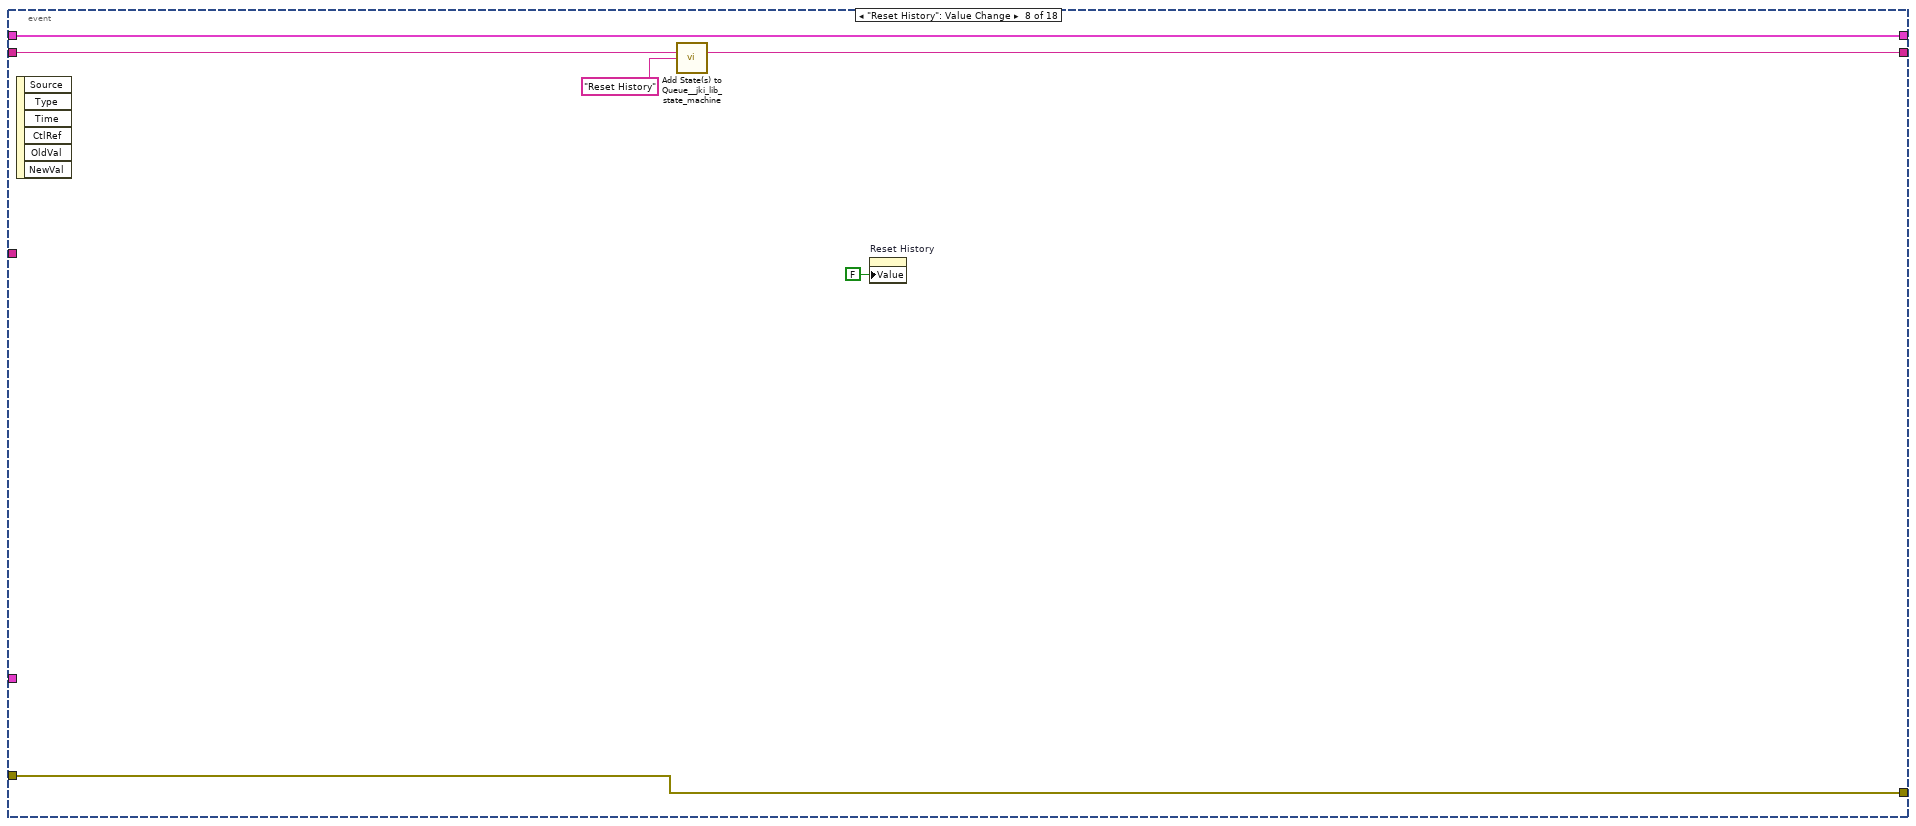
[diagram p14: hidden frame]
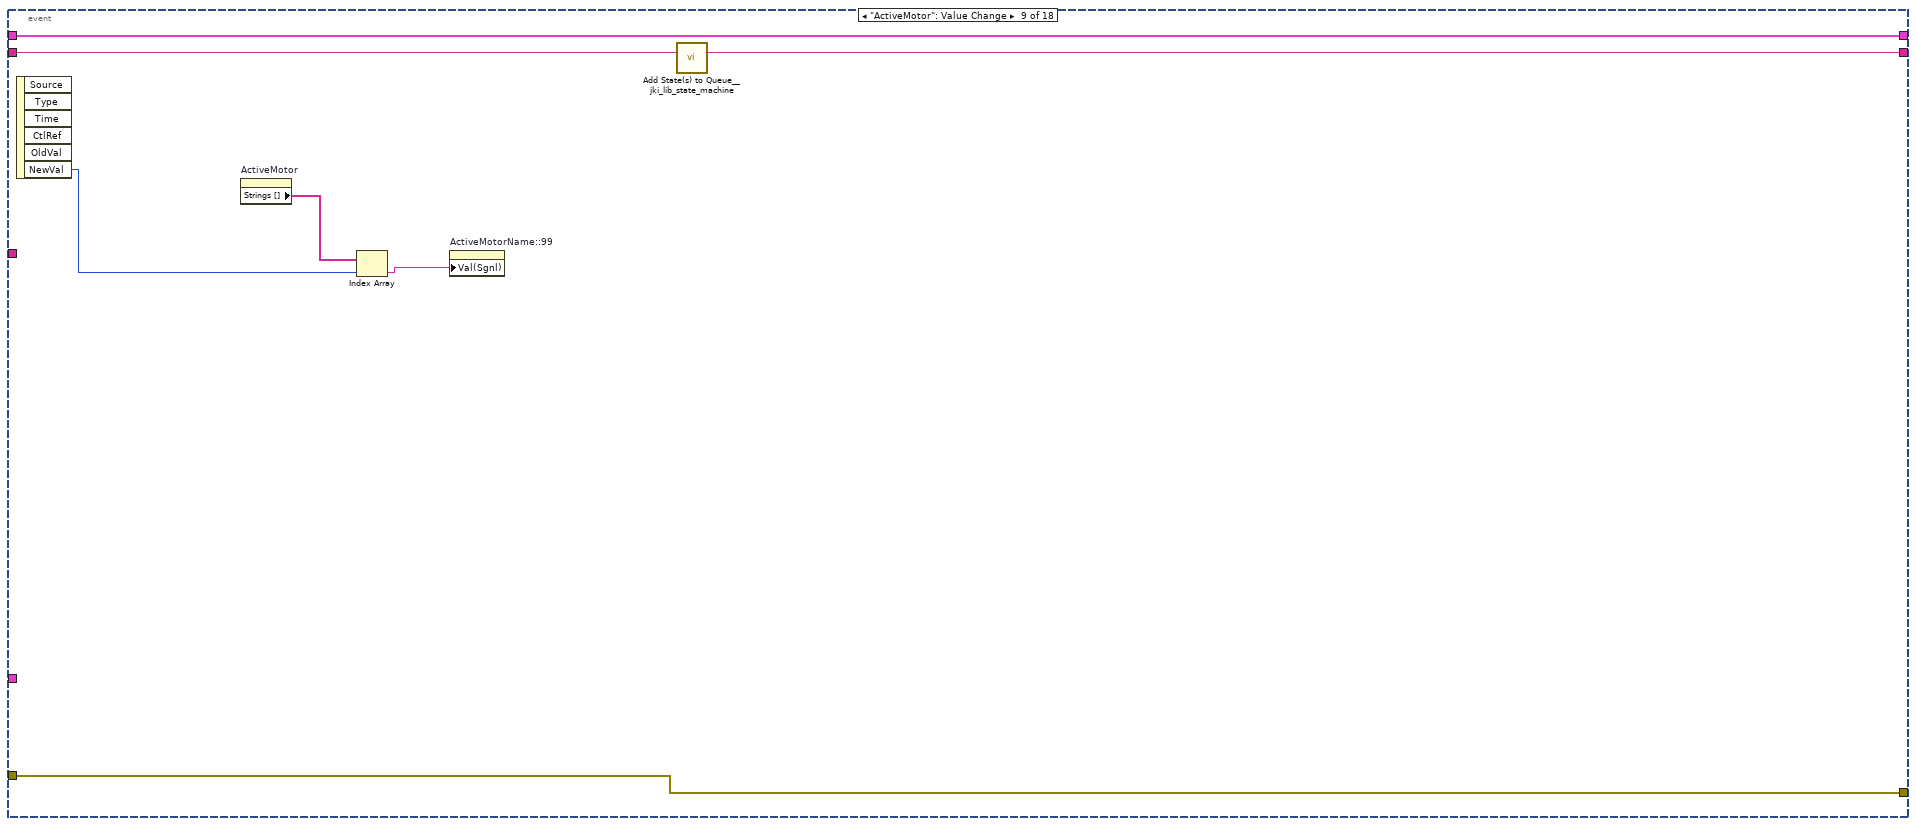
[diagram p15: hidden frame]
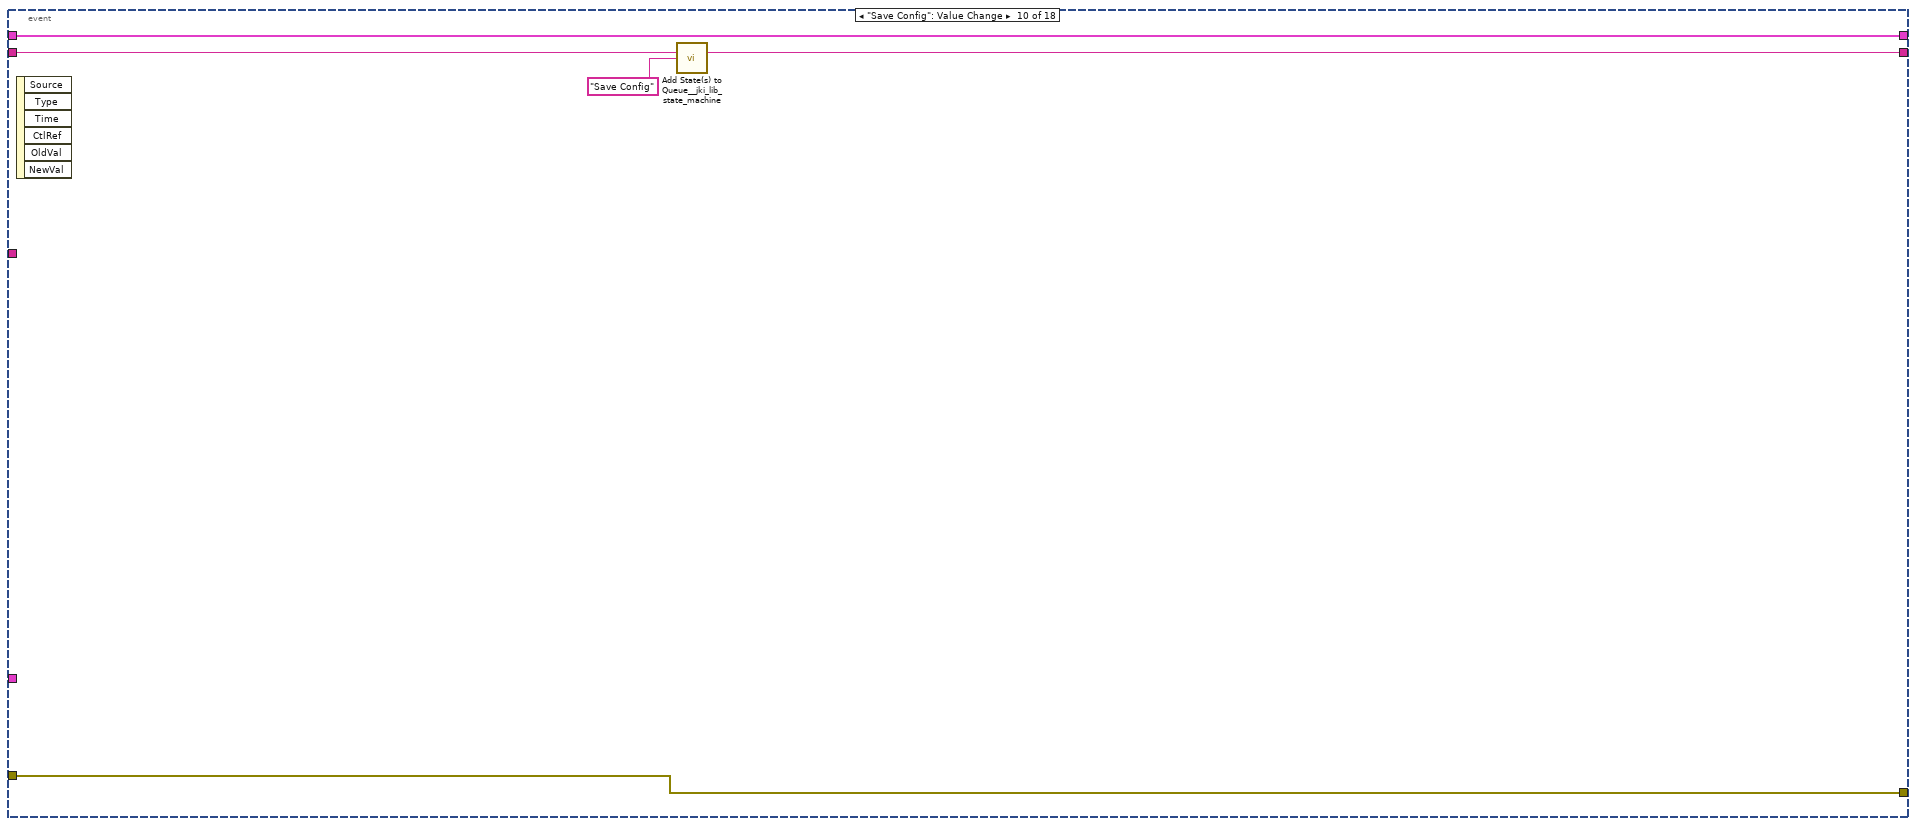
[diagram p16: hidden frame]
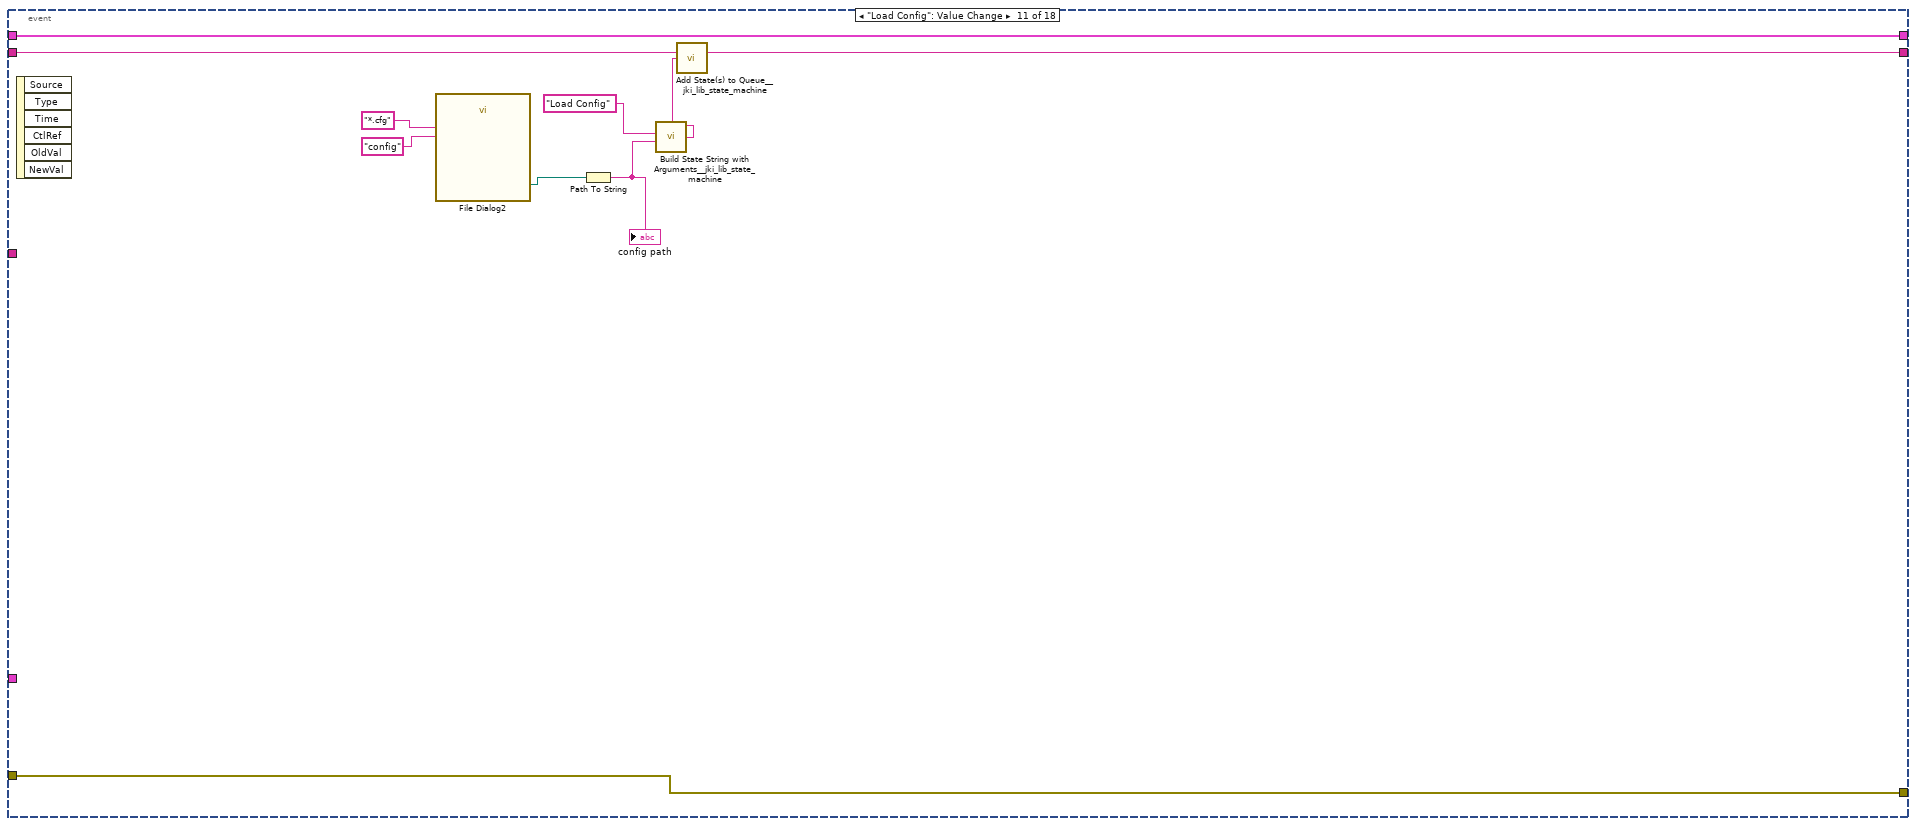
[diagram p17: hidden frame]
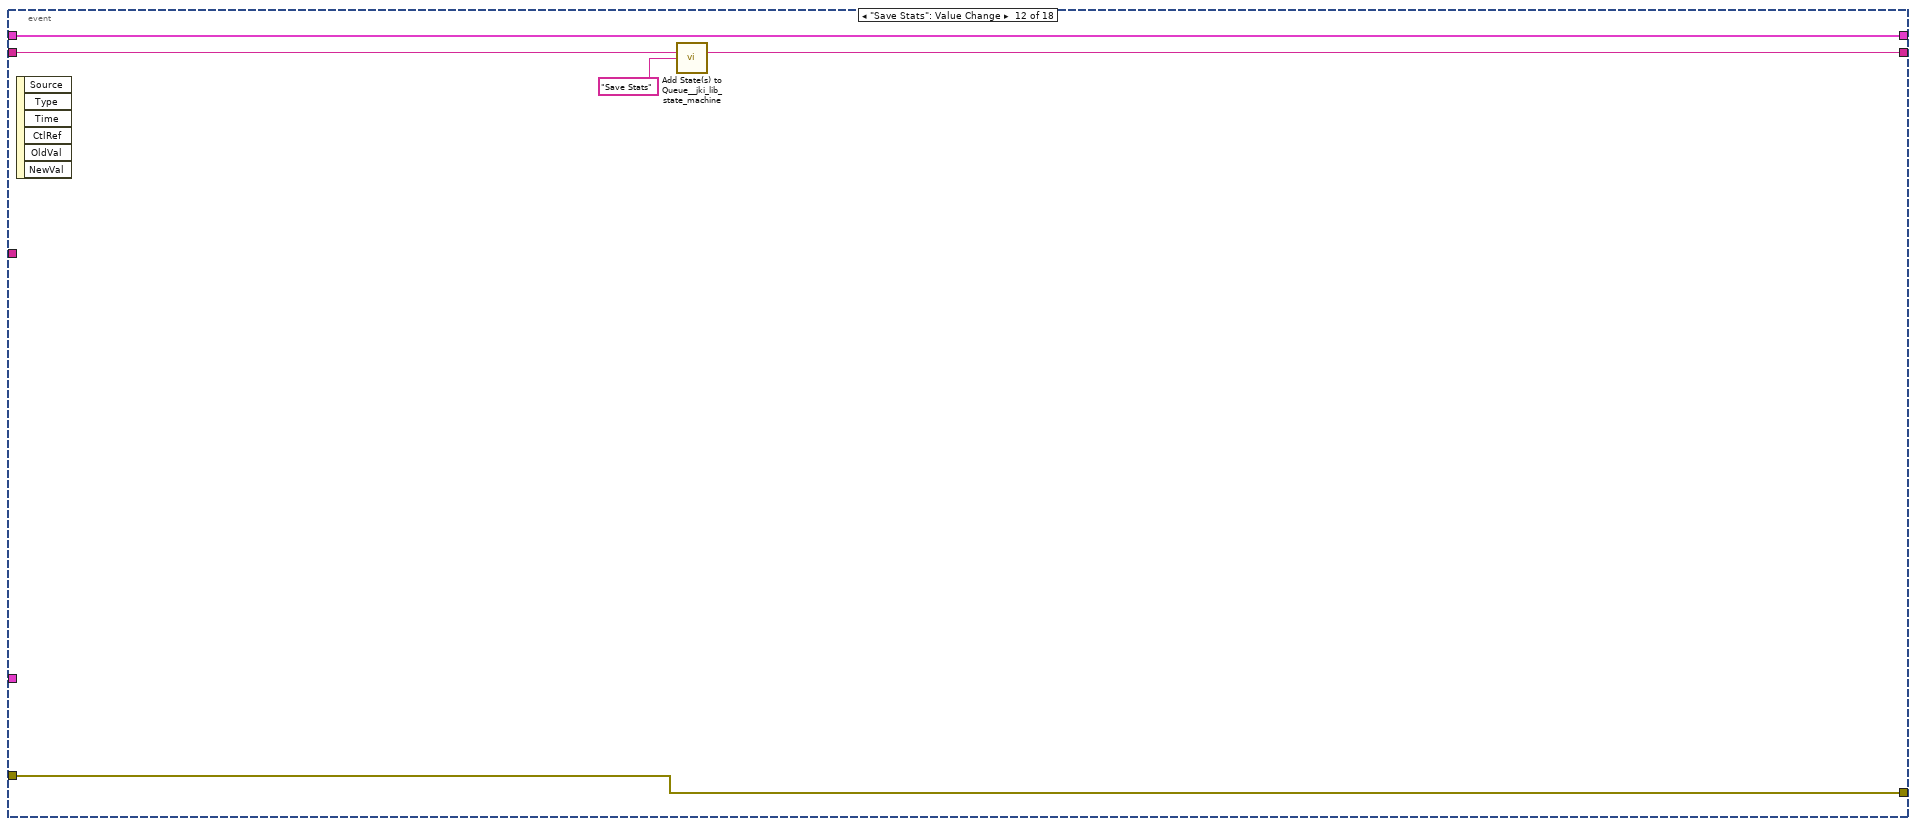
[diagram p18: hidden frame]
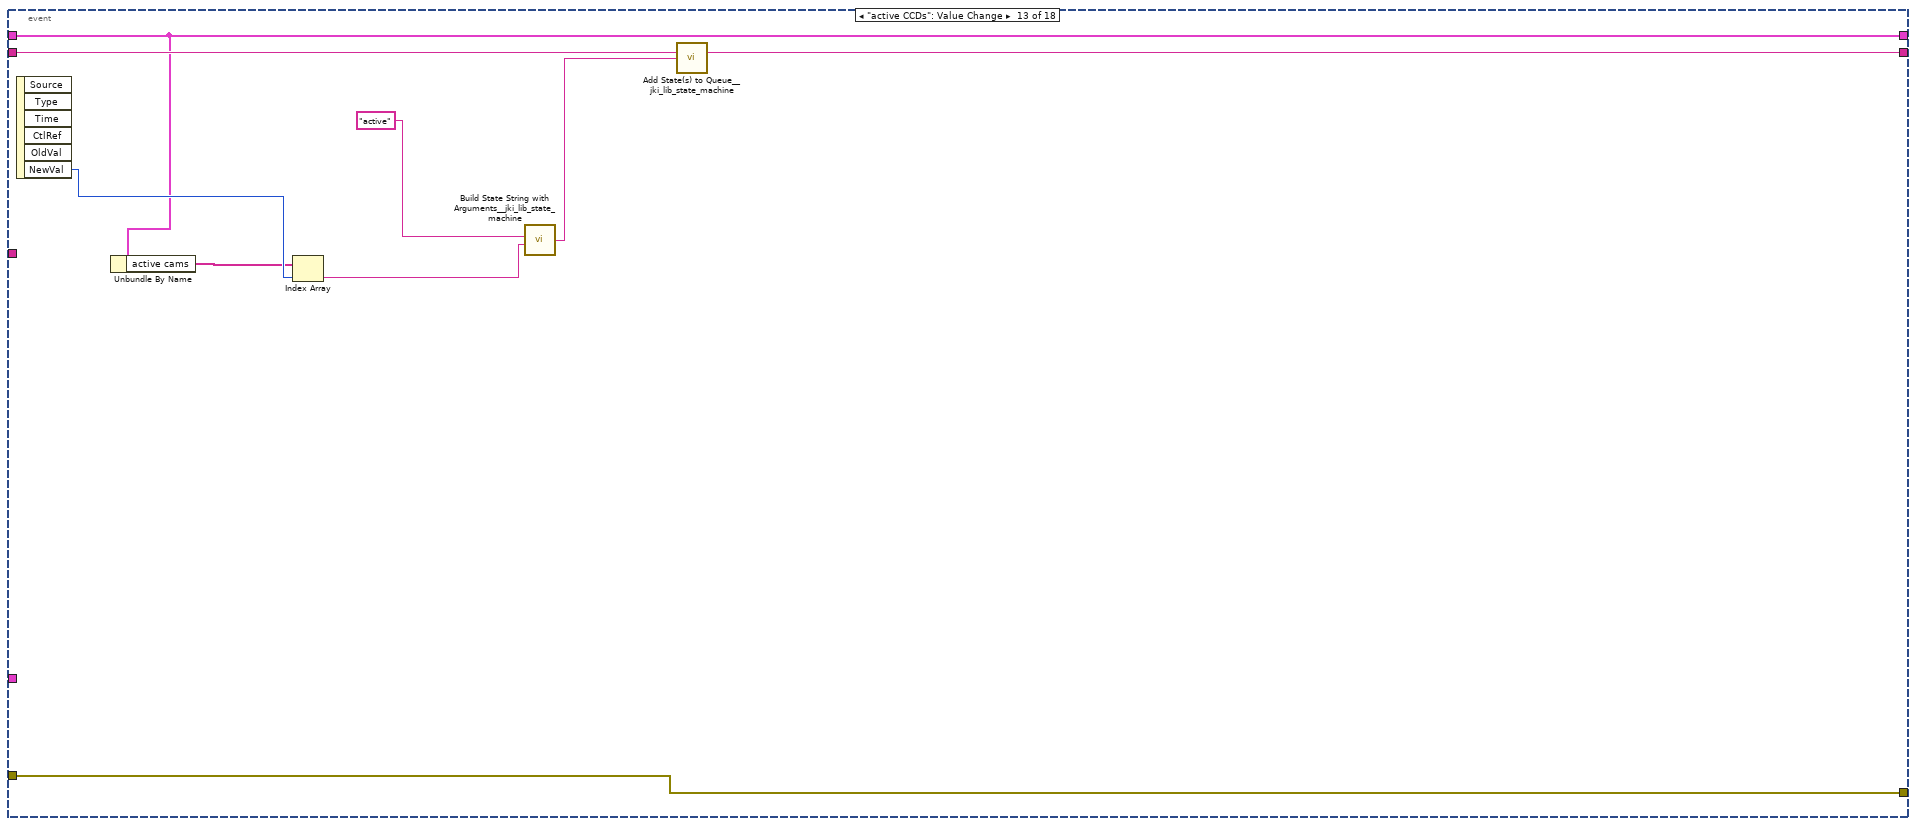
[diagram p19: hidden frame]
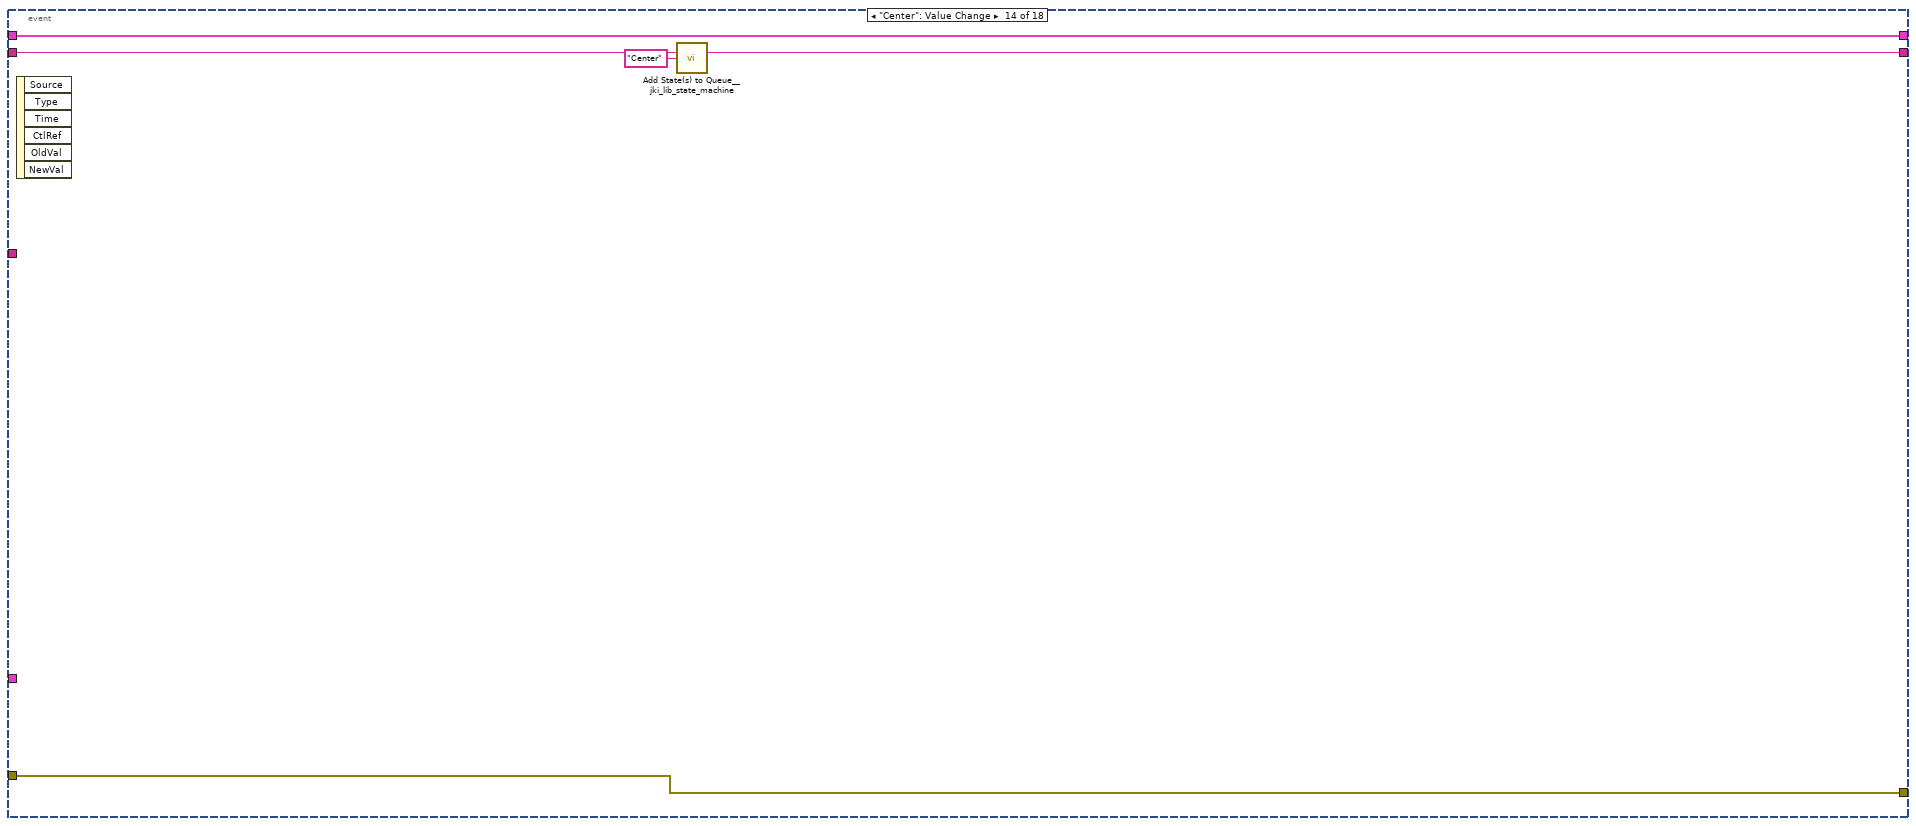
[diagram p20: hidden frame]
diagram:
  n1 = stacked-sequence {
    frame #0 {
      n2 = call <vilib>:"Application Directory.vi"() -> ("Application Directory"=w13:path)
      n3 = Build Path(base path=w13, name or relative path="defaultDevices_PICO.txt") -> (appended path=w15:path)
      "appended path" <- w15
      n4 = call-poly <vilib>:"Read From Spreadsheet File.vi"("file path (dialog if empty)"=w15) -> ("all rows"=w16:string[][])  [unwired: 6 in, 4 out]
      n5 = Index Array(array=w16, index (col) #1=0 ("disabled index (col)"), index (col) #2=1 ("index (col)")) -> (element #1=w19:string[])  [unwired: 2 in, 1 out]
      n6 = Index Array(array=w19, index #1=0 ("index"), index #2=1 ("index"), index #3=2 ("index"), index #4=3 ("index"), index #5=4 ("index"), index #6=5 ("index"), index #7=6 ("index"), index #8=7 ("index"), index #9=8 ("index"), index #10=9 ("index"), index #11=10 ("index"), index #12=11 ("index")) -> (element #1=w12:string, element #2=w11:string, element #3=w10:string, element #4=w9:string, element #5=w8:string, element #6=w7:string, element #7=w6:string, element #8=w5:string, element #9=w4:string, element #10=w3:string, element #11=w2:string, element #12=w1:string)
      n7 = property on="GUIdevice 1" class="Str"("Val(Sgnl)"=w12) -> ()  [unwired: 2 in, 2 out]
      n8 = property on="GUIdevice 2" class="Str"("Val(Sgnl)"=w11) -> ()  [unwired: 2 in, 2 out]
      n9 = property on="GUIdevice 3" class="Str"("Val(Sgnl)"=w10) -> ()  [unwired: 2 in, 2 out]
      n10 = property on="GUIdevice 4" class="Str"("Val(Sgnl)"=w9) -> ()  [unwired: 2 in, 2 out]
      n11 = property on="GUIdevice 5" class="Str"("Val(Sgnl)"=w8) -> ()  [unwired: 2 in, 2 out]
      n12 = property on="GUIdevice 6" class="Str"("Val(Sgnl)"=w7) -> ()  [unwired: 2 in, 2 out]
      n13 = property on="GUIdevice 7" class="Str"("Val(Sgnl)"=w6) -> ()  [unwired: 2 in, 2 out]
      n14 = property on="GUIdevice 8" class="Str"("Val(Sgnl)"=w5) -> ()  [unwired: 2 in, 2 out]
      n15 = property on="GUIdevice 9" class="Str"("Val(Sgnl)"=w4) -> ()  [unwired: 2 in, 2 out]
      n16 = property on="GUIdevice 10" class="Str"("Val(Sgnl)"=w3) -> ()  [unwired: 2 in, 2 out]
      n17 = property on="GUIdevice 11" class="Str"("Val(Sgnl)"=w2) -> ()  [unwired: 2 in, 2 out]
      n18 = property on="GUIdevice 12" class="Str"("Val(Sgnl)"=w1) -> ()  [unwired: 2 in, 2 out]
    }
    frame #1 {
      w32 = path "w:/BP_DATA" ("base path")
      w105 = T20 0 items=["Grayscale (U8)", "Grayscale (I16)", "Grayscale (SGL)", "Complex (CSG)", "RGB (U32)", "HSL (U32)", "RGB (U64)", "Grayscale (U16)"] ("Image Type")
      # "NOT FOR YOU MOFO"
      n19 = control-ref of="Position.Axis 111::98"() -> (w42:refnum<vi>)
      n20 = control-ref of="Position.Axis 112::98"() -> (w43:refnum<vi>)
      n21 = control-ref of="Position.Axis 113::98"() -> (w44:refnum<vi>)
      n22 = control-ref of="Position.Axis 121::98"() -> (w45:refnum<vi>)
      n23 = control-ref of="Position.Axis 122::98"() -> (w46:refnum<vi>)
      n24 = control-ref of="Position.Axis 123::98"() -> (w47:refnum<vi>)
      n25 = control-ref of="Position.Axis 131::98"() -> (w48:refnum<vi>)
      n26 = control-ref of="Position.Axis 132::98"() -> (w49:refnum<vi>)
      n27 = control-ref of="Position.Axis 133::98"() -> (w50:refnum<vi>)
      n28 = control-ref of="Position.Axis 141::98"() -> (w51:refnum<vi>)
      n29 = control-ref of="Position.Axis 142::98"() -> (w52:refnum<vi>)
      n30 = control-ref of="Position.Axis 143::98"() -> (w53:refnum<vi>)
      n31 = control-ref of="Position.Axis 211::98"() -> (w54:refnum<vi>)
      n32 = control-ref of="Position.Axis 212::98"() -> (w55:refnum<vi>)
      n33 = control-ref of="Position.Axis 213::98"() -> (w56:refnum<vi>)
      n34 = control-ref of="Position.Axis 221::98"() -> (w57:refnum<vi>)
      n35 = control-ref of="Position.Axis 222::98"() -> (w58:refnum<vi>)
      n36 = control-ref of="Position.Axis 223::98"() -> (w59:refnum<vi>)
      n37 = control-ref of="Position.Axis 231::98"() -> (w60:refnum<vi>)
      n38 = control-ref of="Position.Axis 232::98"() -> (w61:refnum<vi>)
      n39 = control-ref of="Position.Axis 233::98"() -> (w62:refnum<vi>)
      n40 = control-ref of="Position.Axis 241::98"() -> (w63:refnum<vi>)
      n41 = control-ref of="Position.Axis 242::98"() -> (w64:refnum<vi>)
      n42 = control-ref of="Position.Axis 243::98"() -> (w65:refnum<vi>)
      n43 = control-ref of="Position.Axis 311::98"() -> (w66:refnum<vi>)
      n44 = control-ref of="Position.Axis 312::98"() -> (w67:refnum<vi>)
      n45 = control-ref of="Position.Axis 313::98"() -> (w68:refnum<vi>)
      n46 = control-ref of="Position.Axis 321::98"() -> (w69:refnum<vi>)
      n47 = control-ref of="Position.Axis 322::98"() -> (w70:refnum<vi>)
      n48 = control-ref of="Position.Axis 323::98"() -> (w71:refnum<vi>)
      n49 = control-ref of="Position.Axis 331::98"() -> (w72:refnum<vi>)
      n50 = control-ref of="Position.Axis 332::98"() -> (w73:refnum<vi>)
      n51 = control-ref of="Position.Axis 333::98"() -> (w74:refnum<vi>)
      n52 = control-ref of="Position.Axis 341::98"() -> (w75:refnum<vi>)
      n53 = control-ref of="Position.Axis 342::98"() -> (w76:refnum<vi>)
      n54 = control-ref of="Position.Axis 343::98"() -> (w77:refnum<vi>)
      n55 = control-ref of="Position.Axis 411::98"() -> (w78:refnum<vi>)
      n56 = control-ref of="Position.Axis 412::98"() -> (w79:refnum<vi>)
      n57 = control-ref of="Position.Axis 413::98"() -> (w80:refnum<vi>)
      n58 = control-ref of="Position.Axis 421::98"() -> (w81:refnum<vi>)
      n59 = control-ref of="Position.Axis 422::98"() -> (w82:refnum<vi>)
      n60 = control-ref of="Position.Axis 423::98"() -> (w83:refnum<vi>)
      n61 = control-ref of="Position.Axis 431::98"() -> (w84:refnum<vi>)
      n62 = control-ref of="Position.Axis 432::98"() -> (w85:refnum<vi>)
      n63 = control-ref of="Position.Axis 433::98"() -> (w86:refnum<vi>)
      n64 = control-ref of="Position.Axis 441::98"() -> (w87:refnum<vi>)
      n65 = control-ref of="Position.Axis 442::98"() -> (w88:refnum<vi>)
      n66 = control-ref of="Position.Axis 443::98"() -> (w89:refnum<vi>)
      n67 = control-ref of="Position.Axis 511::98"() -> (w90:refnum<vi>)
      n68 = control-ref of="Position.Axis 512::98"() -> (w91:refnum<vi>)
      n69 = control-ref of="Position.Axis 513::98"() -> (w92:refnum<vi>)
      n70 = control-ref of="Position.Axis 521::98"() -> (w93:refnum<vi>)
      n71 = control-ref of="Position.Axis 522::98"() -> (w94:refnum<vi>)
      n72 = control-ref of="Position.Axis 523::98"() -> (w95:refnum<vi>)
      n73 = control-ref of="Position.Axis 531::98"() -> (w96:refnum<vi>)
      n74 = control-ref of="Position.Axis 532::98"() -> (w97:refnum<vi>)
      n75 = control-ref of="Position.Axis 533::98"() -> (w98:refnum<vi>)
      n76 = control-ref of="Position.Axis 541::98"() -> (w99:refnum<vi>)
      n77 = control-ref of="Position.Axis 542::98"() -> (w100:refnum<vi>)
      n78 = control-ref of="Position.Axis 543::98"() -> (w101:refnum<vi>)
      n79 = control-ref of="Position.Axis 111::99"() -> (w232:refnum<vi>)
      n80 = control-ref of="Position.Axis 112::99"() -> (w231:refnum<vi>)
      n81 = control-ref of="Position.Axis 113::99"() -> (w230:refnum<vi>)
      n82 = control-ref of="Position.Axis 121::99"() -> (w229:refnum<vi>)
      n83 = control-ref of="Position.Axis 122::99"() -> (w228:refnum<vi>)
      n84 = control-ref of="Position.Axis 123::99"() -> (w227:refnum<vi>)
      n85 = control-ref of="Position.Axis 131::99"() -> (w226:refnum<vi>)
      n86 = control-ref of="Position.Axis 132::99"() -> (w225:refnum<vi>)
      n87 = control-ref of="Position.Axis 133::99"() -> (w224:refnum<vi>)
      n88 = control-ref of="Position.Axis 141::99"() -> (w223:refnum<vi>)
      n89 = control-ref of="Position.Axis 142::99"() -> (w222:refnum<vi>)
      n90 = control-ref of="Position.Axis 143::99"() -> (w221:refnum<vi>)
      n91 = control-ref of="Position.Axis 211::99"() -> (w220:refnum<vi>)
      n92 = control-ref of="Position.Axis 212::99"() -> (w219:refnum<vi>)
      n93 = control-ref of="Position.Axis 213::99"() -> (w218:refnum<vi>)
      n94 = control-ref of="Position.Axis 221::99"() -> (w217:refnum<vi>)
      n95 = control-ref of="Position.Axis 222::99"() -> (w216:refnum<vi>)
      n96 = control-ref of="Position.Axis 223::99"() -> (w215:refnum<vi>)
      n97 = control-ref of="Position.Axis 231::99"() -> (w214:refnum<vi>)
      n98 = control-ref of="Position.Axis 232::99"() -> (w213:refnum<vi>)
      n99 = control-ref of="Position.Axis 233::99"() -> (w212:refnum<vi>)
      n100 = control-ref of="Position.Axis 241::99"() -> (w211:refnum<vi>)
      n101 = control-ref of="Position.Axis 242::99"() -> (w210:refnum<vi>)
      n102 = control-ref of="Position.Axis 243::99"() -> (w209:refnum<vi>)
      n103 = control-ref of="Position.Axis 311::99"() -> (w208:refnum<vi>)
      n104 = control-ref of="Position.Axis 312::99"() -> (w207:refnum<vi>)
      n105 = control-ref of="Position.Axis 313::99"() -> (w206:refnum<vi>)
      n106 = control-ref of="Position.Axis 321::99"() -> (w205:refnum<vi>)
      n107 = control-ref of="Position.Axis 322::99"() -> (w204:refnum<vi>)
      n108 = control-ref of="Position.Axis 323::99"() -> (w203:refnum<vi>)
      n109 = control-ref of="Position.Axis 331::99"() -> (w202:refnum<vi>)
      n110 = control-ref of="Position.Axis 332::99"() -> (w201:refnum<vi>)
      n111 = control-ref of="Position.Axis 333::99"() -> (w200:refnum<vi>)
      n112 = control-ref of="Position.Axis 341::99"() -> (w199:refnum<vi>)
      n113 = control-ref of="Position.Axis 342::99"() -> (w198:refnum<vi>)
      n114 = control-ref of="Position.Axis 343::99"() -> (w197:refnum<vi>)
      n115 = control-ref of="Position.Axis 411::99"() -> (w196:refnum<vi>)
      n116 = control-ref of="Position.Axis 412::99"() -> (w195:refnum<vi>)
      n117 = control-ref of="Position.Axis 413::99"() -> (w194:refnum<vi>)
      n118 = control-ref of="Position.Axis 421::99"() -> (w193:refnum<vi>)
      n119 = control-ref of="Position.Axis 422::99"() -> (w192:refnum<vi>)
      n120 = control-ref of="Position.Axis 423::99"() -> (w191:refnum<vi>)
      n121 = control-ref of="Position.Axis 431::99"() -> (w190:refnum<vi>)
      n122 = control-ref of="Position.Axis 432::99"() -> (w189:refnum<vi>)
      n123 = control-ref of="Position.Axis 433::99"() -> (w188:refnum<vi>)
      n124 = control-ref of="Position.Axis 441::99"() -> (w187:refnum<vi>)
      n125 = control-ref of="Position.Axis 442::99"() -> (w186:refnum<vi>)
      n126 = control-ref of="Position.Axis 443::99"() -> (w185:refnum<vi>)
      n127 = control-ref of="Position.Axis 511::99"() -> (w184:refnum<vi>)
      n128 = control-ref of="Position.Axis 512::99"() -> (w183:refnum<vi>)
      n129 = control-ref of="Position.Axis 513::99"() -> (w182:refnum<vi>)
      n130 = control-ref of="Position.Axis 521::99"() -> (w181:refnum<vi>)
      n131 = control-ref of="Position.Axis 522::99"() -> (w180:refnum<vi>)
      n132 = control-ref of="Position.Axis 523::99"() -> (w179:refnum<vi>)
      n133 = control-ref of="Position.Axis 531::99"() -> (w178:refnum<vi>)
      n134 = control-ref of="Position.Axis 532::99"() -> (w177:refnum<vi>)
      n135 = control-ref of="Position.Axis 533::99"() -> (w176:refnum<vi>)
      n136 = control-ref of="Position.Axis 541::99"() -> (w175:refnum<vi>)
      n137 = control-ref of="Position.Axis 542::99"() -> (w174:refnum<vi>)
      n138 = control-ref of="Position.Axis 543::99"() -> (w173:refnum<vi>)
      n139 = Build Array(w42, w43, w44, w45, w46, w47, w48, w49, w50, w51, w52, w53, w54, w55, w56, w57, w58, w59, w60, w61, w62, w63, w64, w65, w66, w67, w68, w69, w70, w71, w72, w73, w74, w75, w76, w77, w78, w79, w80, w81, w82, w83, w84, w85, w86, w87, w88, w89, w90, w91, w92, w93, w94, w95, w96, w97, w98, w99, w100, w101) -> (w39:refnum<vi>[])
      n140 = Build Array(w232, w231, w230, w229, w228, w227, w226, w225, w224, w223, w222, w221, w220, w219, w218, w217, w216, w215, w214, w213, w212, w211, w210, w209, w208, w207, w206, w205, w204, w203, w202, w201, w200, w199, w198, w197, w196, w195, w194, w193, w192, w191, w190, w189, w188, w187, w186, w185, w184, w183, w182, w181, w180, w179, w178, w177, w176, w175, w174, w173) -> (w38:refnum<vi>[])
      n141 = Build Array (concatenate)(w38, w39) -> (→"motor refs":refnum<vi>[])
      n142 = call "getMotorNames.vi"("DeviceName"="GUIdevice 99") -> ("elements"=w36:string[])  [unwired: 10 in]
      n143 = call "getMotorNames.vi"("DeviceName"="GUIdevice 98") -> ("elements"=w35:string[])  [unwired: 10 in]
      n144 = Build Array (concatenate)(w36, w35) -> (w40:string[])
      "Names" <- w40
      n145 = property on="Motor CCD 1" class="Ring (strict)"("Strings []"=w40) -> ()  [unwired: 2 in, 2 out]
      n146 = property on="Motor CCD 2" class="Ring (strict)"("Strings []"=w40) -> ()  [unwired: 2 in, 2 out]
      n147 = property on="Motor CCD 3" class="Ring (strict)"("Strings []"=w40) -> ()  [unwired: 2 in, 2 out]
      n148 = property on="Motor CCD 4" class="Ring (strict)"("Strings []"=w40) -> ()  [unwired: 2 in, 2 out]
      n149 = property on="Motor CCD 5" class="Ring (strict)"("Strings []"=w40) -> ()  [unwired: 2 in, 2 out]
      n150 = property on="Motor CCD 6" class="Ring (strict)"("Strings []"=w40) -> ()  [unwired: 2 in, 2 out]
      n151 = property on="Motor CCD 7" class="Ring (strict)"("Strings []"=w40) -> ()  [unwired: 2 in, 2 out]
      n152 = property on="Motor CCD 8" class="Ring (strict)"("Strings []"=w40) -> ()  [unwired: 2 in, 2 out]
      n153 = property on="Motor CCD 9" class="Ring (strict)"("Strings []"=w40) -> ()  [unwired: 2 in, 2 out]
      n154 = property on="Motor CCD 10" class="Ring (strict)"("Strings []"=w40) -> ()  [unwired: 2 in, 2 out]
      n155 = property on="Motor CCD 11" class="Ring (strict)"("Strings []"=w40) -> ()  [unwired: 2 in, 2 out]
      n156 = property on="Motor CCD 12" class="Ring (strict)"("Strings []"=w40) -> ()  [unwired: 2 in, 2 out]
      n157 = property on="ActiveMotor" class="Ring (strict)"("Strings []"=w36) -> ()  [unwired: 2 in, 2 out]
      n158 = control-ref of="Target.X::1"() -> (w159:refnum<vi>)
      n159 = control-ref of="Target.Y::1"() -> (w158:refnum<vi>)
      n160 = control-ref of="Target.X::2"() -> (w157:refnum<vi>)
      n161 = control-ref of="Target.Y::2"() -> (w156:refnum<vi>)
      n162 = control-ref of="Target.X::3"() -> (w155:refnum<vi>)
      n163 = control-ref of="Target.Y::3"() -> (w154:refnum<vi>)
      n164 = control-ref of="Target.X::4"() -> (w153:refnum<vi>)
      n165 = control-ref of="Target.Y::4"() -> (w152:refnum<vi>)
      n166 = control-ref of="Target.X::5"() -> (w151:refnum<vi>)
      n167 = control-ref of="Target.Y::5"() -> (w150:refnum<vi>)
      n168 = control-ref of="Target.X::6"() -> (w149:refnum<vi>)
      n169 = control-ref of="Target.Y::6"() -> (w148:refnum<vi>)
      n170 = control-ref of="Target.X::7"() -> (w147:refnum<vi>)
      n171 = control-ref of="Target.Y::7"() -> (w146:refnum<vi>)
      n172 = control-ref of="Target.X::8"() -> (w145:refnum<vi>)
      n173 = control-ref of="Target.Y::8"() -> (w144:refnum<vi>)
      n174 = control-ref of="Target.X::9"() -> (w122:refnum<vi>)
      n175 = control-ref of="Target.Y::9"() -> (w121:refnum<vi>)
      n176 = control-ref of="Target.X::10"() -> (w120:refnum<vi>)
      n177 = control-ref of="Target.Y::10"() -> (w119:refnum<vi>)
      n178 = control-ref of="Target.X::11"() -> (w118:refnum<vi>)
      n179 = control-ref of="Target.Y::11"() -> (w117:refnum<vi>)
      n180 = control-ref of="Target.X::12"() -> (w116:refnum<vi>)
      n181 = control-ref of="Target.Y::12"() -> (w115:refnum<vi>)
      n182 = call "IMAQ Create"("Image Name"="GUIdevice 8", "Image Type"=w105) -> ("New Image"=→"image::8":T9)  [unwired: 3 in, 1 out]
      n183 = call "IMAQ Create"("Image Name"="GUIdevice 9", "Image Type"=w105) -> ("New Image"=→"image::9":T9)  [unwired: 3 in, 1 out]
      n184 = call "IMAQ Create"("Image Name"="GUIdevice 10", "Image Type"=w105) -> ("New Image"=→"image::10":T9)  [unwired: 3 in, 1 out]
      n185 = call "IMAQ Create"("Image Name"="GUIdevice 6", "Image Type"=w105) -> ("New Image"=→"image::6":T9)  [unwired: 3 in, 1 out]
      n186 = call "IMAQ Create"("Image Name"="GUIdevice 7", "Image Type"=w105) -> ("New Image"=→"image::7":T9)  [unwired: 3 in, 1 out]
      n187 = call "IMAQ Create"("Image Name"="GUIdevice 11", "Image Type"=w105) -> ("New Image"=→"image::11":T9)  [unwired: 3 in, 1 out]
      n188 = call "IMAQ Create"("Image Name"="GUIdevice 12", "Image Type"=w105) -> ("New Image"=→"image::12":T9)  [unwired: 3 in, 1 out]
      n189 = call "IMAQ Create"("Image Name"="GUIdevice 2") -> ("New Image"=→"image::2":T9)  [unwired: 4 in, 1 out]
      n190 = call "IMAQ Create"("Image Name"="GUIdevice 4", "Image Type"=w105) -> ("New Image"=→"image::4":T9)  [unwired: 3 in, 1 out]
      n191 = call "IMAQ Create"("Image Name"="GUIdevice 1", "Image Type"=w105) -> ("New Image"=→"image::1":T9)  [unwired: 3 in, 1 out]
      n192 = call "IMAQ Create"("Image Name"="GUIdevice 3", "Image Type"=w105) -> ("New Image"=→"image::3":T9)  [unwired: 3 in, 1 out]
      n193 = call "IMAQ Create"("Image Name"="GUIdevice 5", "Image Type"=w105) -> ("New Image"=→"image::5":T9)  [unwired: 3 in, 1 out]
      n194 = Build Array("GUIdevice 1", "GUIdevice 2", "GUIdevice 3", "GUIdevice 4", "GUIdevice 5", "GUIdevice 6", "GUIdevice 7", "GUIdevice 8", "GUIdevice 9", "GUIdevice 10", "GUIdevice 11", "GUIdevice 12") -> (w133:string[])
      "CCDs" <- w133
      n195 = property on="image::8" class="ImageControl"("Caption.Text"="GUIdevice 8") -> ()  [unwired: 2 in, 2 out]
      n196 = property on="image::10" class="ImageControl"("Caption.Text"="GUIdevice 10") -> ()  [unwired: 2 in, 2 out]
      n197 = property on="image::9" class="ImageControl"("Caption.Text"="GUIdevice 9") -> ()  [unwired: 2 in, 2 out]
      n198 = property on="image::1" class="ImageControl"("Caption.Text"="GUIdevice 1") -> ()  [unwired: 2 in, 2 out]
      n199 = property on="image::2" class="ImageControl"("Caption.Text"="GUIdevice 2") -> ()  [unwired: 2 in, 2 out]
      n200 = property on="image::3" class="ImageControl"("Caption.Text"="GUIdevice 3") -> ()  [unwired: 2 in, 2 out]
      n201 = property on="image::4" class="ImageControl"("Caption.Text"="GUIdevice 4") -> ()  [unwired: 2 in, 2 out]
      n202 = property on="image::5" class="ImageControl"("Caption.Text"="GUIdevice 5") -> ()  [unwired: 2 in, 2 out]
      n203 = property on="image::6" class="ImageControl"("Caption.Text"="GUIdevice 6") -> ()  [unwired: 2 in, 2 out]
      n204 = property on="image::7" class="ImageControl"("Caption.Text"="GUIdevice 7") -> ()  [unwired: 2 in, 2 out]
      n205 = property on="image::11" class="ImageControl"("Caption.Text"="GUIdevice 11") -> ()  [unwired: 2 in, 2 out]
      n206 = property on="image::12" class="ImageControl"("Caption.Text"="GUIdevice 12") -> ()  [unwired: 2 in, 2 out]
      n207 = Array To Cluster(array=w133) -> (cluster=→"Cameras":T21)
      n208 = Bundle("Target.X::1"=w159, "Target.Y::1"=w158) -> (w143:T22)  [unwired: 1 in]
      n209 = Bundle("Target.X::2"=w157, "Target.Y::2"=w156) -> (w142:T23)  [unwired: 1 in]
      n210 = Bundle("Target.X::3"=w155, "Target.Y::3"=w154) -> (w141:T24)  [unwired: 1 in]
      n211 = Bundle("Target.X::4"=w153, "Target.Y::4"=w152) -> (w134:T25)  [unwired: 1 in]
      n212 = Bundle("Target.X::5"=w151, "Target.Y::5"=w150) -> (w140:T26)  [unwired: 1 in]
      n213 = Bundle("Target.X::6"=w149, "Target.Y::6"=w148) -> (w139:T27)  [unwired: 1 in]
      n214 = Bundle("Target.X::7"=w147, "Target.Y::7"=w146) -> (w138:T28)  [unwired: 1 in]
      n215 = Bundle("Target.X::8"=w145, "Target.Y::8"=w144) -> (w137:T29)  [unwired: 1 in]
      n216 = Bundle("Target.X::12"=w116, "Target.Y::12"=w115) -> (w111:T30)  [unwired: 1 in]
      n217 = Bundle("Target.X::9"=w122, "Target.Y::9"=w121) -> (w114:T31)  [unwired: 1 in]
      n218 = Bundle("Target.X::10"=w120, "Target.Y::10"=w119) -> (w113:T32)  [unwired: 1 in]
      n219 = Bundle("Target.X::11"=w118, "Target.Y::11"=w117) -> (w112:T33)  [unwired: 1 in]
      n220 = property on="CCDs" class="Ring (strict)"("Strings []"=w133) -> ()  [unwired: 2 in, 2 out]
      n221 = Build Array(w143, w142, w141, w134, w140, w139, w138, w137, w114, w113, w112, w111) -> (w136:T34)
      n222 = Tick Count (ms)() -> (millisecond timer value=→"millisecond timer value":u32)
      n223 = property on="Feedback Global" class="Bool (strict)"("Value"=FALSE ("Feedback Global")) -> ()  [unwired: 2 in, 2 out]
      n224 = Get Date/Time In Seconds() -> (seconds since 1Jan1904=w124:timestamp)
      n225 = Format Date/Time String(time format string (%c)="%Y%m%d%H%M", seconds (now)=w124) -> (date/time string=w123:string)  [unwired: 1 in]
      n226 = Concatenate Strings(w123, "Beampointing_Pico.tdms" ("string")) -> (w127:string)
      n227 = String To Path(string=w127) -> (path=w126:path)
      n228 = Build Path(base path=w32, name or relative path=w126) -> (appended path=w33:path)
      n229 = call <vilib>:"Add State(s) to Queue__jki_lib_state_machine.vi"("State(s) in (\"\")"="Macro: Initialize") -> ("States Out"=w234:string)  [unwired: 14 in]
      n230 = Create User Event(user event datatype=T14 {"EventEnum"=enum."new data", "Device name"="Device name"} ("New Event")) -> (user event=w242:refnum<user-event>, error out=w244:errorcluster)  [unwired: 1 in]
      "tcp data event" <- w242
      n231 = while "JKI - String-Based Queued State Machine (Basic) v1.0" {
        shift-right: [w267] -> w132
        shift-left: _ -> [w255]
        shift-right: [w270] -> w160
        shift-left: _ -> [w266]
        shift-right: [w269] -> _
        shift-left: w234 -> [w271]
        tunnel: w136 -> [w264]
        tunnel: w133 -> [w262]
        tunnel: [w262] -> w161
        tunnel: w136 -> [w263]
        tunnel: w33 -> [w253]
        tunnel: w32 -> [w252]
        stop <- w268 stop-if-true
        n232 = Unbundle By Name(w255) -> ("active cams"=w254:string[])
        n233 = call <vilib>:"Parse State Queue__jki_lib_state_machine.vi"("State Queue"=w271, "Error In (no error)"=w266) -> ("Remaining States"=w273:string, "Current State"=w274:string, "Arguments"=w272:string)  [unwired: 11 in]
        "Current State" <- w274
        n234 = case shown="\"\", \"Idle\"" w274 {
          selector: w274 -> [_ _ w560 _ _ _ _ _ _ _ _ _ _ _ _ _ _ _ _ _ _ _ _ _ _ _ _ _ _ _ _ _ _ _ _ _ _ _ _ _]
          tunnel: w273 -> [w303 w559 w564 w582 w588 w593 w597 w639 w647 w651 w655 w661 w672 w696 w706 w716 w720 w742 w844 w896 w909 w918 w945 w966 w970 w989 w1128 w1282 w1373 w1439 w1477 w1497 w1512 w1600 w1652 w1662 w1669 w1693 w1713 w1740]
          tunnel: w272 -> [_ _ _ _ _ _ _ _ _ _ _ w656 w667 _ _ _ _ w737 w795 _ w906 _ _ _ _ w991 _ w1260 w1350 _ _ _ _ _ _ _ w1666 _ _ _]
          tunnel: w255 -> [w301 w556 w562 w572 w585 w591 w594 _ w643 w648 w653 w659 w666 w693 w704 w708 w717 w734 w796 w894 w901 w914 w937 w959 w967 w973 w1122 w1275 w1366 w1436 w1448 w1494 w1509 w1572 w1649 w1659 w1665 w1680 w1710 w1731]
          tunnel: [w300 w557 w566 w580 errorcluster {"status"=FALSE, "code"=0, "source"=""} ("error out") w590 w595 w607 w640 w649 w652 w657 w669 w694 w705 w714 w718 w738 w800 w885 w907 w916 w943 w964 w968 w993 w1152 w1280 w1371 w1437 w1475 w1495 w1510 w1590 w1650 w1660 w1667 w1673 w1711 w1738] -> w270
          tunnel: w266 -> [w299 w557 w565 w580 w584 w590 w595 w614 w645 w649 w652 w658 w670 w694 w705 w714 w718 w738 w798 w886 w907 w916 w943 w964 w968 w993 w1152 w1280 w1371 w1437 w1475 w1495 w1510 w1595 w1650 w1660 w1667 w1678 w1711 w1738]
          tunnel: [w302 w558 w563 w581 w587 w592 w596 w638 w646 w650 w654 w660 w671 w695 w697 w715 w719 w728 w843 w895 w908 w917 w944 w965 w969 w996 w1153 w1281 w1372 w1438 w1476 w1496 w1511 w1560 w1651 w1661 w1668 w1692 w1712 w1739] -> w269
          tunnel: [_ _ _ _ _ TRUE _ _ _ _ _ _ _ _ _ _ _ _ _ _ _ _ _ _ _ _ _ _ _ _ _ _ _ _ _ _ _ _ _ _] -> w268
          tunnel: [w296 w556 w562 w571 w585 w591 w594 w599 w643 w648 w653 w659 w666 w693 w704 w708 w717 w739 w833 w894 w900 w913 w936 w958 w967 w1018 w1121 w1275 w1366 w1435 w1448 w1494 w1509 w1572 w1648 w1659 w1664 w1681 w1710 w1730] -> w267
          tunnel: "update speed [ms]" -> [w298 _ _ _ _ _ _ _ _ _ _ _ _ _ _ _ _ _ _ _ _ _ _ _ _ _ _ _ _ _ _ _ _ _ _ _ _ _ _ _]
          tunnel: w264 -> [w295 _ _ _ _ _ _ _ _ _ _ _ _ _ _ _ _ _ _ _ _ _ _ _ _ w1016 _ _ _ _ _ _ _ _ _ _ _ _ w1694 _]
          tunnel: w262 -> [w297 _ _ _ _ _ _ w605 _ _ _ _ _ _ _ _ _ w741 w797 _ w902 _ _ _ _ w981 w1118 w1279 w1370 _ w1449 _ w1498 w1598 _ _ _ w1676 _ _]
          tunnel: w253 -> [_ _ _ _ _ _ _ w612 _ _ _ _ _ _ _ _ _ _ _ _ _ _ _ _ _ _ _ _ _ _ _ _ _ _ _ _ _ _ _ _]
          tunnel: w252 -> [_ _ _ _ _ _ _ _ _ _ _ _ _ _ _ _ _ _ _ _ _ _ _ _ _ _ _ _ _ _ _ _ _ _ _ _ _ w1672 _ _]
          frame "", "Idle" {
            # "executes when the state queue is empty"
            n235 = event shown="[0] Timeout" {
              selector: _ -> [_ _ _ _ _ _ _ _ _ _ _ _ _ _ _ _ _ _]
              dyn-events: _ -> [_ _ _ _ _ _ _ _ _ _ _ _ _ _ _ _ _ _]
              timeout: w298 -> [_ _ _ _ _ _ _ _ _ _ _ _ _ _ _ _ _ _]
              tunnel: w303 -> [w306 w433 w448 w467 w472 w477 w482 w488 w495 w500 w510 w515 w524 w529 w535 w541 w549 w555]
              tunnel: [w321 w432 w447 w466 w471 w476 w481 w487 w494 w499 w509 w514 w523 w528 w534 w540 w548 w554] -> w302
              tunnel: w301 -> [w311 w430 w444 w463 w469 w474 w479 w485 w492 w497 w507 w512 w517 w526 w532 w538 w546 w552]
              tunnel: [w315 w431 w446 w465 w470 w475 w480 w486 w493 w498 w508 w513 w522 w527 w533 w539 w547 w553] -> w300
              tunnel: w299 -> [w318 w431 w446 w465 w470 w475 w480 w486 w493 w498 w508 w513 w522 w527 w533 w539 w547 w553]
              tunnel: [w320 w430 w444 w462 w469 w474 w479 w485 w492 w497 w507 w512 w517 w526 w532 w538 w546 w552] -> w296
              tunnel: w297 -> [w338 _ w440 _ _ _ _ _ _ _ _ _ _ _ _ _ _ _]
              tunnel: w295 -> [_ _ w442 _ _ _ _ _ _ _ _ _ _ _ _ _ _ _]
              event Timeout {
                n236 = event-data() -> ()  [unwired: 1 in, 1 out]
                n237 = Unbundle By Name(w311) -> ("Centroid X"=w308:dbl[][], "Centroid Y"=w348:dbl[][], "Size"=w341:dbl[][], "detection para"=w337:T3[], "active cams"=w332:string[], "thresholds"=w329:cluster{"Lower value":sgl, "Upper value":sgl}[])
                n238 = Unbundle By Name(w311) -> ("active ccd"=w310:i32)
                n239 = call <userlib>:"Tick Count (ms)__ogtk.vi"("error in (no error)"=w318) -> ("error out"=w317:errorcluster, "millisecond timer value"=→"millisecond timer 2":u32)  [unwired: 9 in]
                n240 = for {
                  N: 12 ("Numeric 2") -> [_]
                  tunnel: w332 -> [w393] mode=indexing
                  tunnel: [w394] -> w346 mode=indexing
                  tunnel: w338 -> [w417]
                  tunnel: w337 -> [w415]
                  tunnel: [w413] -> w314 mode=indexing
                  tunnel: [w412] -> w312 mode=indexing
                  tunnel: [w410] -> w333 mode=indexing
                  tunnel: "autodetect" -> [w404]
                  tunnel: w317 -> [w418]
                  tunnel: [w419] -> w339
                  shift-right: [w401] -> w309
                  shift-left: w329 -> [w403]
                  shift-right: [w388] -> w347
                  shift-left: w308 -> [w390]
                  shift-right: [w384] -> w349
                  shift-left: w348 -> [w386]
                  shift-right: [w378] -> w340
                  shift-left: w341 -> [w380]
                  w382 = 0 ("index")
                  n241 = call-poly <userlib>:"Filter 1D Array__ogtk.vi"("items to filter"=w393, "array"=w417) -> ("filtered item indices"=w416:i32[])  [unwired: 4 in, 1 out]
                  n242 = Index Array(array=w416) -> (element=w379:i32)  [unwired: 1 in]
                  n243 = Index Array(array=w380, index (row)=w379) -> (element=w408:dbl[])  [unwired: 1 in]
                  n244 = Index Array(array=w386, index (row)=w379) -> (element=w409:dbl[])  [unwired: 1 in]
                  n245 = Index Array(array=w403, index=w379) -> (element=w407:cluster{"Lower value":sgl, "Upper value":sgl})
                  n246 = Index Array(array=w390, index (row)=w379) -> (element=w392:dbl[])  [unwired: 1 in]
                  n247 = Index Array(array=w415, index=w379) -> (element=w411:T3)
                  n248 = call "CENTRIOD DETECTION.vi"("Refnum in"=w393, "auto threshold"=w404, "Threshold Range In"=w407, "beam detection para"=w411, "error in (no error)"=w418) -> ("Bounding Rect"=w410:T35, "Particle Reports (Pixels)"=w412:T1, "Threshold Range Out"=w402:cluster{"Lower value":sgl, "Upper value":sgl}, "Centriod"=w420:cluster{"X":dbl, "Y":dbl}, "error out"=w419:errorcluster)  [unwired: 7 in, 3 out]
                  n249 = Unbundle By Name(w420) -> ("X"=w391:dbl, "Y"=w387:dbl)
                  n250 = Empty Array?(array=w412) -> (empty?=w414:bool)
                  n251 = Not(x=w414) -> (.not. x?=w413:bool)
                  n252 = Replace Array Subset(array=w403, new element=w402, index=w379) -> (w401:cluster{"Lower value":sgl, "Upper value":sgl}[])
                  n253 = Unbundle By Name(w410) -> ("Right"=w400:dbl, "Left"=w399:dbl, "Bottom"=w398:dbl, "Top"=w397:dbl)
                  n254 = Subtract(x=w400, y=w399) -> (x-y=w395:dbl)
                  n255 = Subtract(x=w398, y=w397) -> (x-y=w396:dbl)
                  n256 = Multiply(x=w395, y=w396) -> (x*y=w383:dbl)
                  n257 = Insert Into Array(array=w409, index=w382, new element=w387) -> (w385:dbl[])
                  n258 = Insert Into Array(array=w408, index=w382, new element=w383) -> (w381:dbl[])
                  n259 = Insert Into Array(array=w392, index=w382, new element=w391) -> (w389:dbl[])
                  n260 = for {
                    shift-right: [w421] -> w405
                    shift-left: dbl[] [] ("Array 4") -> [w424]
                    tunnel: w385 -> [w422] mode=indexing
                    n261 = Equal To 0?(x=w422) -> (x = 0?=w423:bool)
                    n262 = case shown="False" w423 {
                      tunnel: w424 -> [w427 w428]
                      tunnel: w422 -> [w426 _]
                      tunnel: [w425 w428] -> w421
                      frame False {
                        n263 = Build Array (concatenate)(w427, w426) -> (w425:dbl[])
                      }
                      frame True {
                      }
                    }
                  }
                  n264 = Replace Array Subset(array=w390, new element=w389, index (row)=w379) -> (w388:dbl[][])  [unwired: 1 in]
                  n265 = Replace Array Subset(array=w386, new element=w385, index (row)=w379) -> (w384:dbl[][])  [unwired: 1 in]
                  n266 = Replace Array Subset(array=w380, new element=w381, index (row)=w379) -> (w378:dbl[][])  [unwired: 1 in]
                  n267 = Array Size(array=w405) -> (size(s)=w394:i32)
                }
                "detected" <- w314
                "Particle Reports (Pixels)" <- w312
                "Box" <- w333
                n268 = Bundle(0, 1, "Centroid X"=w308) -> (→"Status":cluster{i32, i32, "Centroid X":dbl[][]})  [unwired: 1 in]
                n269 = Index Array(array=w312, index (row)=w310) -> (element=→"particles":T1)  [unwired: 1 in]
                n270 = call <vilib>:"Clear Errors.vi"("error in (no error)"=w339) -> ("error out"=w315:errorcluster)  [unwired: 6 in]
                n271 = local read "Img to avg"() -> (w323:i32)
                n272 = local read "Numeric"() -> (w326:dbl)
                n273 = Increment(x=w323) -> (x+1=w322:i32)
                n274 = Greater Or Equal?(x=w326, y=w322) -> (x >= y?=w319:bool)
                n275 = Increment(x=w326) -> (x+1=w325:dbl)
                n276 = Select(t=0.0, s=w319, f=w325) -> (s? t:f=w324:dbl)
                n277 = local write "Numeric"(w324) -> ()
                n278 = for {
                  tunnel: w346 -> [w370] mode=indexing
                  tunnel: w332 -> [w377] mode=indexing
                  shift-right: [w372] -> w342
                  shift-left: "" ("GUIdevice 7") -> [w375]
                  tunnel: [w365] -> w344 mode=indexing
                  tunnel: "Detection Rate" -> [w369]
                  tunnel: w324 -> [w367]
                  n279 = local read "Img to avg"() -> (w371:i32)
                  n280 = Greater Or Equal?(x=w370, y=w371) -> (x >= y?=w366:bool)
                  n281 = Multiply(x=w369, y=w367) -> (x*y=w368:dbl)
                  n282 = Greater Or Equal?(x=w370, y=w368) -> (x >= y?=w364:bool)
                  n283 = And(x=w366, y=w364) -> (x .and. y?=w365:bool)
                  n284 = Select(t=w377, s=w365, f="") -> (s? t:f=w373:string)
                  n285 = Concatenate Strings(w375, "\t", w373) -> (w372:string)
                }
                n286 = Bundle By Name(cluster=w311, "thresholds"=w309, "detected"=w314) -> (w330:T36)
                n287 = Bundle By Name(cluster=w330, "Centroid X"=w347, "Centroid Y"=w349, "Size"=w340) -> (w305:T36)
                n288 = Unbundle By Name(w305) -> ("img to avg"=w304:i32)
                n289 = Or Array Elements(Boolean array=w344) -> (logical OR=w343:bool)
                n290 = case shown="True" w319 {
                  tunnel: w305 -> [w350 w357]
                  tunnel: [w350 w356] -> w320
                  tunnel: w304 -> [_ w352]
                  frame False {
                  }
                  frame True {
                    n291 = Decrement(x=w352) -> (x-1=w351:i32)
                    n292 = Initialize Array(0.0 ("element"), 12 ("dimension size"), w351) -> (w353:dbl[][])
                    n293 = Bundle By Name(cluster=w357, "Centroid X"=w353, "Centroid Y"=w353, "Size"=w353) -> (w356:T36)
                  }
                }
                n294 = case shown="True" w343 {
                  tunnel: w342 -> [_ w362]
                  tunnel: w306 -> [w358 w360]
                  tunnel: [w358 w359] -> w321
                  frame False {
                  }
                  frame True {
                    n295 = call <vilib>:"Build State String with Arguments__jki_lib_state_machine.vi"("Arguments (\"\")"=w362, "State"="detected") -> ("State with Arguments"=w361:string)  [unwired: 4 in]
                    n296 = call <vilib>:"Add State(s) to Queue__jki_lib_state_machine.vi"("State(s) in (\"\")"=w360, "State(s) at Back (\"\")"=w361) -> ("States Out"=w359:string)  [unwired: 13 in]
                  }
                }
              }
              event "stop": Value Change {
                # "Exit Button Value Change (pressed) Event\n(this executes Macro: Exit to terminate the VI)"
                n297 = event-data() -> ()  [unwired: 1 in, 6 out]
                n298 = call <vilib>:"Add State(s) to Queue__jki_lib_state_machine.vi"("State(s) in Front (\"\")"="Macro: Exit", "State(s) in (\"\")"=w433) -> ("States Out"=w432:string)  [unwired: 13 in]
              }
              event Value Change {
                n299 = event-data() -> ()  [unwired: 1 in, 6 out]
                n300 = property on="Set Centriod Target" class="Bool (strict)"("Value"=FALSE) -> ()  [unwired: 2 in, 2 out]
                n301 = Unbundle By Name(w444) -> ("active ccd"=w436:i32, "Centroid X"=w435:dbl[][], "Centroid Y"=w434:dbl[][])
                n302 = Index Array(array=w440, index=w436) -> (element=w439:string)
                n303 = Concatenate Strings("Do want to update the target of " ("message"), w439, "?" ("string")) -> (w437:string)
                n304 = Two Button Dialog(message=w437) -> (T button?=w443:bool)  [unwired: 2 in]
                n305 = case shown="True" w443 {
                  tunnel: w442 -> [_ w455]
                  tunnel: w436 -> [_ w454]
                  tunnel: w435 -> [_ w461]
                  tunnel: w434 -> [_ w456]
                  frame False {
                  }
                  frame True {
                    n306 = Index Array(array=w461, index (row)=w454) -> (element=w460:dbl[])  [unwired: 1 in]
                    n307 = Index Array(array=w456, index (row)=w454) -> (element=w457:dbl[])  [unwired: 1 in]
                    n308 = Index Array(array=w455, index=w454) -> (element=w453:T30)
                    n309 = Unbundle By Name(w453) -> ("Target.X::12"=w452:refnum<vi>, "Target.Y::12"=w450:refnum<vi>)
                    n310 = Reverse 1D Array(array=w460) -> (reversed array=w459:dbl[])
                    n311 = Reverse 1D Array(array=w457) -> (reversed array=w458:dbl[])
                    n312 = Index Array(array=w459) -> (element=w451:dbl)  [unwired: 1 in]
                    n313 = Index Array(array=w458) -> (element=w449:dbl)  [unwired: 1 in]
                    n314 = property class="DigNum (strict)"(reference=w452, "Val(Sgnl)"=w451) -> ()  [unwired: 1 in, 2 out]
                    n315 = property class="DigNum (strict)"(reference=w450, "Val(Sgnl)"=w449) -> ()  [unwired: 1 in, 2 out]
                  }
                }
                n316 = call <vilib>:"Add State(s) to Queue__jki_lib_state_machine.vi"("State(s) in (\"\")"=w448) -> ("States Out"=w447:string)  [unwired: 14 in]
              }
              event "Feedback Global": Value Change {
                # "Exit Button Value Change (pressed) Event\n(this executes Macro: Exit to terminate the VI)"
                n317 = event-data() -> ("NewVal"=w464:bool)  [unwired: 1 in, 5 out]
                n318 = call <vilib>:"Add State(s) to Queue__jki_lib_state_machine.vi"("State(s) in (\"\")"=w467) -> ("States Out"=w466:string)  [unwired: 14 in]
                n319 = Bundle By Name(cluster=w463, "Feedback global"=w464) -> (w462:T36)
              }
              event Value Change {
                n320 = event-data() -> ()  [unwired: 1 in, 6 out]
                n321 = call <vilib>:"Add State(s) to Queue__jki_lib_state_machine.vi"("State(s) in Front (\"\")"="Move Config", "State(s) in (\"\")"=w472) -> ("States Out"=w471:string)  [unwired: 13 in]
              }
              event Value Change {
                n322 = event-data() -> ()  [unwired: 1 in, 6 out]
                n323 = call <vilib>:"Add State(s) to Queue__jki_lib_state_machine.vi"("State(s) in Front (\"\")"="Detection Config", "State(s) in (\"\")"=w477) -> ("States Out"=w476:string)  [unwired: 13 in]
              }
              event "associated motors": Value Change {
                n324 = event-data() -> ()  [unwired: 1 in, 6 out]
                n325 = call <vilib>:"Add State(s) to Queue__jki_lib_state_machine.vi"("State(s) in (\"\")"=w482, "State(s) at Back (\"\")"="Motor Config" ("State(s) at Back (\"\")")) -> ("States Out"=w481:string)  [unwired: 13 in]
              }
              event "Reset History": Value Change {
                n326 = event-data() -> ()  [unwired: 1 in, 6 out]
                n327 = call <vilib>:"Add State(s) to Queue__jki_lib_state_machine.vi"("State(s) in (\"\")"=w488, "State(s) at Back (\"\")"="Reset History" ("State(s) at Back (\"\")")) -> ("States Out"=w487:string)  [unwired: 13 in]
                n328 = property on="Reset History" class="Bool (strict)"("Value"=FALSE ("Reset History")) -> ()  [unwired: 2 in, 2 out]
              }
              event "ActiveMotor": Value Change {
                n329 = event-data() -> ("NewVal"=w490:u16)  [unwired: 1 in, 5 out]
                n330 = property on="ActiveMotor" class="Ring (strict)"() -> ("Strings []"=w491:string[])  [unwired: 2 in, 2 out]
                n331 = Index Array(array=w491, index=w490) -> (element=w489:string)
                n332 = property on="ActiveMotorName::99" class="Str"("Val(Sgnl)"=w489) -> ()  [unwired: 2 in, 2 out]
                n333 = call <vilib>:"Add State(s) to Queue__jki_lib_state_machine.vi"("State(s) in (\"\")"=w495) -> ("States Out"=w494:string)  [unwired: 14 in]
              }
              event "Save Config": Value Change {
                n334 = event-data() -> ()  [unwired: 1 in, 6 out]
                n335 = call <vilib>:"Add State(s) to Queue__jki_lib_state_machine.vi"("State(s) in (\"\")"=w500, "State(s) at Back (\"\")"="Save Config" ("State(s) at Back (\"\")")) -> ("States Out"=w499:string)  [unwired: 13 in]
              }
              event "Load Config": Value Change {
                n336 = event-data() -> ()  [unwired: 1 in, 6 out]
                n337 = call "File Dialog2"("pattern (all files)"="*.cfg", "pattern label"="config") -> ("selected path"=w504:path)  [unwired: 10 in, 3 out]
                n338 = Path To String(path=w504) -> (string=w502:string)
                "config path" <- w502
                n339 = call <vilib>:"Build State String with Arguments__jki_lib_state_machine.vi"("Arguments (\"\")"=w502, "State"="Load Config" ("State(s) at Back (\"\")")) -> ("State with Arguments"=w501:string)  [unwired: 4 in]
                n340 = call <vilib>:"Add State(s) to Queue__jki_lib_state_machine.vi"("State(s) in (\"\")"=w510, "State(s) at Back (\"\")"=w501) -> ("States Out"=w509:string)  [unwired: 13 in]
              }
              event "Save Stats": Value Change {
                n341 = event-data() -> ()  [unwired: 1 in, 6 out]
                n342 = call <vilib>:"Add State(s) to Queue__jki_lib_state_machine.vi"("State(s) in (\"\")"=w515, "State(s) at Back (\"\")"="Save Stats" ("State(s) at Back (\"\")")) -> ("States Out"=w514:string)  [unwired: 13 in]
              }
              event "active CCDs": Value Change {
                n343 = event-data() -> ("NewVal"=w521:i32)  [unwired: 1 in, 5 out]
                n344 = Unbundle By Name(w517) -> ("active cams"=w516:string[])
                n345 = Index Array(array=w516, index=w521) -> (element=w519:string)
                n346 = call <vilib>:"Build State String with Arguments__jki_lib_state_machine.vi"("Arguments (\"\")"=w519, "State"="active" ("State(s) at Back (\"\")")) -> ("State with Arguments"=w518:string)  [unwired: 4 in]
                n347 = call <vilib>:"Add State(s) to Queue__jki_lib_state_machine.vi"("State(s) in (\"\")"=w524, "State(s) at Back (\"\")"=w518) -> ("States Out"=w523:string)  [unwired: 13 in]
              }
              event "Center": Value Change {
                n348 = event-data() -> ()  [unwired: 1 in, 6 out]
                n349 = call <vilib>:"Add State(s) to Queue__jki_lib_state_machine.vi"("State(s) in (\"\")"=w529, "State(s) at Back (\"\")"="Center" ("State(s) at Back (\"\")")) -> ("States Out"=w528:string)  [unwired: 13 in]
              }
              event "new tdms": Value Change {
                n350 = event-data() -> ()  [unwired: 1 in, 6 out]
                n351 = property on="new tdms" class="Bool (strict)"("Value"=FALSE ("new tdms")) -> ()  [unwired: 2 in, 2 out]
                n352 = call <vilib>:"Add State(s) to Queue__jki_lib_state_machine.vi"("State(s) in (\"\")"=w535, "State(s) at Back (\"\")"="newtdms" ("State(s) at Back (\"\")")) -> ("States Out"=w534:string)  [unwired: 13 in]
              }
              event "deivice ini": Value Change {
                n353 = event-data() -> ()  [unwired: 1 in, 6 out]
                n354 = property on="deivice ini" class="Bool (strict)"("Value"=FALSE ("new tdms")) -> ()  [unwired: 2 in, 2 out]
                n355 = call <vilib>:"Add State(s) to Queue__jki_lib_state_machine.vi"("State(s) in (\"\")"=w541, "State(s) at Back (\"\")"="Device Ini" ("State(s) at Back (\"\")")) -> ("States Out"=w540:string)  [unwired: 13 in]
              }
              event "Img to avg": Value Change {
                n356 = event-data() -> ()  [unwired: 1 in, 6 out]
                n357 = property on="Img to avg" class="DigNum (strict)"() -> ("Value"=w544:i32)  [unwired: 2 in, 2 out]
                n358 = Number To Decimal String(number=w544) -> (decimal integer string=w543:string)  [unwired: 1 in]
                n359 = call <vilib>:"Build State String with Arguments__jki_lib_state_machine.vi"("Arguments (\"\")"=w543, "State"="ImgToAvg" ("State(s) at Back (\"\")")) -> ("State with Arguments"=w542:string)  [unwired: 4 in]
                n360 = call <vilib>:"Add State(s) to Queue__jki_lib_state_machine.vi"("State(s) in (\"\")"=w549, "State(s) at Back (\"\")"=w542) -> ("States Out"=w548:string)  [unwired: 13 in]
              }
              event Panel Close? {
                # "Discard the event because we'll close the front panel ourselves in Macro: Exit"
                # "Close Panel button (pressed) Event\n(this executes Macro: Exit to terminate the VI)"
                n361 = event-data() -> ()  [unwired: 1 in, 1 out]
                n362 = call <vilib>:"Add State(s) to Queue__jki_lib_state_machine.vi"("State(s) in Front (\"\")"="Macro: Exit", "State(s) in (\"\")"=w555) -> ("States Out"=w554:string)  [unwired: 13 in]
                n363 = event-data("Discard?"=TRUE) -> ()  [unwired: 1 in, 1 out]
              }
            }
          }
          frame "---------- Core ----------" {
            # "Do not put any code in this frame.\n(it is a separator no-op)"
            n364 = call <vilib>:"Add State(s) to Queue__jki_lib_state_machine.vi"("State(s) in (\"\")"=w559) -> ("States Out"=w558:string)  [unwired: 14 in]
          }
          frame Default {
            w569 = 42 items=["No error", "Argument error", "Memory is full", "Out of zone", "End of file", "File already open", "Generic file I/O error", "File not found", "File permission error", "Disk is full", "Duplicate path", "Too many files open", "System feature not enabled", "Resource file not found", "Cannot add resource", "Resource not found", "Image not found", "Image memory error", "Pen does not exist", "Config type invalid", "Config token not found", "Config parse error", "Config memory error", "Bad external code format", "Bad external code offset", "External code not present", "Null window", "Destroy window error", "Null menu", "Print aborted", "Bad print record", "Print driver error", "Windows error during printing", "Memory error during printing", "Print dialog error", "Generic print error", "Invalid device refnum", "Device not found", "Device parameter error", "Device unit error", "Cannot open device", "Device call aborted", "Generic error", "Cancelled by user", "Object ID too low", "Object ID too high", "Object not in heap", "Unknown heap", "Unknown object (invalid DefProc)", "Unknown object (DefProc not in table)", "Message out of range", "Invalid (null) method", "Unknown message", "Manager call not supported", "Bad address", "Network operation in progress", "Network operation timed out", "Connection is busy", "Network attribute not supported", "Network error", "Address in use", "System out of memory", "Connection aborted", "Connection refused", "Not connected", "Already connected", "Connection closed", "Initialization error (interapplication manager)", "Bad occurrence", "Wait on unbound occurrence handler", "Occurrence queue overflow", "Datalog type conflict", "Unused", "Unrecognized type (interapplication manager)", "Memory corrupt", "Failed to make temporary DLL", "Old CIN version", "Drag socket not found", "Failed to load drop-object", "Failed to register OLE object", "Failed to release OLE object", "Format specifier type mismatch", "Unknown format specifier", "Too few format specifiers", "Too many format specifiers", "Scan failed", "Newer CIN version", "Error converting to variant", "Runtime menu error", "Password tampered", "Variant attribute not found", "Incompatible variant data type", "Event data is not available", "Event Store is not present", "Occurrence is not found", "Event Queue is not created", "Event info is not available", "Refnum passed is NULL", "Error retrieving Class GUID", "Error retrieving CoClass GUID", "Error retrieving TypeLib GUID.", "Bad built application magic bytes.", "Specific driver is different from the specific driver associated with the Logical Name.", "There is no session opened to the class driver.", "Max Error", "MAX - Error with config objects", "MAX - Error loading configuration", "MAX - Group not supported"]
            # "Current State"
            # "Do not delete, rename, or modify this frame.\n(this is used to capture unhandled states and typos)"
            # "Handle mistyped state name (developer tool)"
            n365 = Format Into String(format string="Software Exception: Unhandled State \"%s\"." ("message"), error in=w565, w560) -> (resulting string=w568:string, error out=w567:errorcluster)  [unwired: 1 in]
            n366 = call <vilib>:"Error Cluster From Error Code.vi"("show call chain? (False)"=TRUE, "error in (no error)"=w567, "error message (\"\")"=w568, "error code (0)"=w569) -> ("error out"=w566:errorcluster)  [unwired: 5 in]
            n367 = call <vilib>:"Add State(s) to Queue__jki_lib_state_machine.vi"("State(s) in (\"\")"=w564) -> ("States Out"=w563:string)  [unwired: 14 in]
          }
          frame "Initialize Core Data" {
            # "Do not delete, rename, or modify this frame.\n(this is used to determine panel behavior on exit)"
            # "originally closed?"
            # "exe?"
            # "If panel starts closed or is an EXE, then close it when we exit"
            n368 = property class="VI"() -> ("Front Panel.Open"=w579:bool)  [unwired: 2 in, 2 out]
            n369 = property class="App"() -> ("App.Kind"=w578:T16)  [unwired: 2 in, 2 out]
            n370 = control-ref of="Current VI Reference"() -> (w573:refnum<vi>)
            n371 = Not(x=w579) -> (.not. x?=w576:bool)
            n372 = Equal?(x=w578, y=T16."Run Time System" ("Application:Kind")) -> (x = y?=w575:bool)
            n373 = Or(x=w576, y=w575) -> (x .or. y?=w574:bool)
            n374 = Bundle By Name(cluster=w572, "Core.Current VI Reference"=w573, "Core.Close Panel on Exit?"=w574) -> (w571:T36)
            n375 = call <vilib>:"Add State(s) to Queue__jki_lib_state_machine.vi"("State(s) in (\"\")"=w582) -> ("States Out"=w581:string)  [unwired: 14 in]
          }
          frame "Error Handler" {
            # "Unhandled Error -- Display it"
            # "Handle any errors here.\nYou can also output any states to clean-up after errors occur"
            # "Clear error"
            n376 = call <vilib>:"General Error Handler.vi"("error in (no error)"=w584) -> ()  [unwired: 10 in, 5 out]
            n377 = call <vilib>:"Add State(s) to Queue__jki_lib_state_machine.vi"("State(s) in Front (\"\")"="/* Post Error States", "State(s) in (\"\")"=w588) -> ("States Out"=w587:string)  [unwired: 13 in]
          }
          frame "Exit" {
            # "Do not put any code in this frame.\n(No errors that occur here will be handled.)"
            n378 = call <vilib>:"Add State(s) to Queue__jki_lib_state_machine.vi"("State(s) in (\"\")"=w593) -> ("States Out"=w592:string)  [unwired: 14 in]
          }
          frame "---------- Data ----------" {
            # "Do not put any code in this frame.\n(It is a separator no-op. You can make a copy of this frame to create a new Data frame)"
            n379 = call <vilib>:"Add State(s) to Queue__jki_lib_state_machine.vi"("State(s) in (\"\")"=w597) -> ("States Out"=w596:string)  [unwired: 14 in]
          }
          frame "Data: Initialize" {
            w609 = bool[] [FALSE, FALSE, FALSE, FALSE, FALSE, FALSE, FALSE, FALSE, FALSE, FALSE, FALSE, TRUE]  # speedmode Y
            w610 = bool[] [FALSE, FALSE, FALSE, FALSE, FALSE, FALSE, FALSE, FALSE, FALSE, FALSE, FALSE, TRUE]  # speedmode X
            w611 = bool[] [FALSE, FALSE, FALSE, FALSE, TRUE, TRUE, TRUE, FALSE, FALSE, FALSE, FALSE, FALSE]  # detected
            w613 = cluster{"Lower value":sgl, "Upper value":sgl}[] [{"Lower value"=93.0, "Upper value"=255.0}, {"Lower value"=105.0, "Upper value"=255.0}, {"Lower value"=0.0, "Upper value"=255.0}, {"Lower value"=127.0, "Upper value"=255.0}, {"Lower value"=0.0, "Upper value"=255.0}, {"Lower value"=0.0, "Upper value"=255.0}, {"Lower value"=0.0, "Upper value"=255.0}, {"Lower value"=0.0, "Upper value"=255.0}, {"Lower value"=0.0, "Upper value"=255.0}, {"Lower value"=0.0, "Upper value"=255.0}, {"Lower value"=0.0, "Upper value"=255.0}, {"Lower value"=0.0, "Upper value"=255.0}]  # thresholds
            w624 = FALSE  # Feedback global
            w626 = 0  # active ccd
            w598 = 2  # img to avg
            w637 = T37 {"Current VI Reference"=refnum, "Close Panel on Exit?"=FALSE}  # Core
            # "Initialize the shift-register data, here.\n(data names are defined by what you wire into the bundle function)"
            n380 = TDMS Open(6:FALSE ("disable buffering (T)"), 7:enum16{"1.0", "2.0"}."2.0" ("file format version (2.0)"), 8:w614, 10:T17."create or replace" ("operation"), 11:w612) -> (0:w608:errorcluster, 3:w606:refnum<k34>)  [unwired: 2 in]
            n381 = call "TDMSbuffersize.vi"("error in (no error)"=w608, "group names"=w605, "Data Value Reference in"=w606) -> ("error out"=w607:errorcluster, "Data Value Reference out"=w604:refnum<k34>)  [unwired: 7 in]
            n382 = call <vilib>:"Add State(s) to Queue__jki_lib_state_machine.vi"("State(s) in (\"\")"=w639) -> ("States Out"=w638:string)  [unwired: 14 in]
            n383 = Bundle("Core"=w637, "detection para"="detection para", "thresholds"=w613, "Centroid X"="Centroid X", "Centroid Y"="Centroid Y", "img to avg"=w598, "Mean Centroid X"="Mean Centroid X", "Mean Centroid Y"="Mean Centroid Y", "Offset X"="Offset X", "Offset Y"="Offset Y", "Offset X stats"="Offset X stats", "Offset Y stats"="Offset Y stats", "Size"="Size", "Mean Size"="Mean Size", "Time"="Time", "move properties"="move properties", "active axis refs 2"="active axis refs 2", "active ccd"=w626, "Feedback global"=w624, "Motor X"="Motor X", "Motor Y"="Motor Y", "active cams"="active cams", "Data Value Reference out"=w604, "detected"=w611, "speedmode X"=w610, "speedmode Y"=w609) -> (w600:T36)  [unwired: 1 in]
            n384 = Initialize Array(0.0 ("element"), 12 ("dimension size"), w598) -> (w601:dbl[][])
            n385 = Bundle By Name(cluster=w600, "Centroid X"=w601, "Centroid Y"=w601, "Size"=w601) -> (w599:T36)
          }
          frame "Data: Cleanup" {
            # "Cleanup any data and references, here.\n(this is called automatically, by the Macro: Exit)"
            n386 = Unbundle By Name(w643) -> ("Core.Current VI Reference"=w644:refnum<vi>)
            n387 = Close Reference(reference=w644, error in (no error)=w645) -> (error out=w641:errorcluster)
            n388 = Unbundle By Name(w643) -> ("Data Value Reference out"=w642:refnum<k34>)
            n389 = TDMS Close(8:w641, 11:w642) -> (0:w640:errorcluster)  [unwired: 1 out]
            n390 = call <vilib>:"Add State(s) to Queue__jki_lib_state_machine.vi"("State(s) in (\"\")"=w647) -> ("States Out"=w646:string)  [unwired: 14 in]
          }
          frame "---------- UI ----------" {
            # "Do not put any code in this frame.\n(It is a separator no-op. You can make a copy of this frame to create a new UI frame)"
            n391 = call <vilib>:"Add State(s) to Queue__jki_lib_state_machine.vi"("State(s) in (\"\")"=w651) -> ("States Out"=w650:string)  [unwired: 14 in]
          }
          frame "UI: Initialize" {
            # "Initialize the User Interface, here.\n(this is called automatically, by the Macro: Init)"
            n392 = call <vilib>:"Add State(s) to Queue__jki_lib_state_machine.vi"("State(s) in (\"\")"=w655) -> ("States Out"=w654:string)  [unwired: 14 in]
          }
          frame "UI: Cursor Set" {
            # "Argument"
            # "Set and Unset Cursor Busy.\n(Usage: \"UI: Cursor Set >> Busy|Idle\")"
            n393 = case shown="\"Idle\", Default" w656 {
              tunnel: w658 -> [w663 w665]
              tunnel: [w662 w664] -> w657
              frame "Idle", Default {
                n394 = call <vilib>:"Unset Busy.vi"("error in (no error)"=w663) -> ("error out"=w662:errorcluster)  [unwired: 10 in]
              }
              frame "Busy" {
                n395 = call <vilib>:"Set Busy.vi"("error in (no error)"=w665) -> ("error out"=w664:errorcluster)  [unwired: 9 in, 1 out]
              }
            }
            n396 = call <vilib>:"Add State(s) to Queue__jki_lib_state_machine.vi"("State(s) in (\"\")"=w661) -> ("States Out"=w660:string)  [unwired: 14 in]
          }
          frame "UI: Front Panel State" {
            # "Argument"
            # "Set Front Panel Open or Closed\n(Usage: \"UI: Front Panel State >> Open|Close\")"
            n397 = Unbundle By Name(w666) -> ("Core.Current VI Reference"=w668:refnum<vi>)
            n398 = case shown="\"Open\", Default" w667 {
              tunnel: w670 -> [w676 w687]
              tunnel: [w677 w688] -> w669
              tunnel: w668 -> [_ _]
              frame "Open", Default {
                n399 = property class="VI"(error in=w676) -> (reference out=w674:refnum<vi>, error out=w675:errorcluster, "Front Panel.Open"=w673:bool)  [unwired: 1 in]
                n400 = case shown="False" w673 {
                  tunnel: [w680 w683] -> w677
                  tunnel: w675 -> [w679 w683]
                  tunnel: w674 -> [w678 _]
                  frame False {
                    n401 = invoke class="VI" method="FP.Open"(reference=w678, error in=w679, "Activate"=TRUE, "State"=T18."Standard") -> (error out=w680:errorcluster)  [unwired: 1 in, 4 out]
                  }
                  frame True {
                  }
                }
              }
              frame "Close" {
                n402 = property class="VI"(error in=w687) -> (reference out=w685:refnum<vi>, error out=w686:errorcluster, "Front Panel.Open"=w684:bool)  [unwired: 1 in]
                n403 = case shown="True" w684 {
                  tunnel: [w689 w692] -> w688
                  tunnel: w686 -> [w689 w691]
                  tunnel: w685 -> [_ w690]
                  frame False {
                  }
                  frame True {
                    n404 = invoke class="VI" method="FP.Close"(reference=w690, error in=w691) -> (error out=w692:errorcluster)  [unwired: 1 in, 2 out]
                  }
                }
              }
            }
            n405 = call <vilib>:"Add State(s) to Queue__jki_lib_state_machine.vi"("State(s) in (\"\")"=w672) -> ("States Out"=w671:string)  [unwired: 14 in]
          }
          frame "---------- Macro ----------" {
            # "Do not put any code in this frame.\n(It is a separator no-op. You can make a copy of this frame to create a new Macro frame)"
            n406 = call <vilib>:"Add State(s) to Queue__jki_lib_state_machine.vi"("State(s) in (\"\")"=w696) -> ("States Out"=w695:string)  [unwired: 14 in]
          }
          frame "Macro: Initialize" {
            w703 = "Data: Initialize\nInitialize Core Data\nUI: Initialize\nUI: Front Panel State >> Open\nDevice Ini >> 3000"  # Data: Initialize Initialize Core Data UI: Initialize UI: Front Panel State >> Open Device Ini >> 3000
            # "Initialization Macro\n(This is called once, when the VI starts)"
            n407 = property on="Img to avg" class="DigNum (strict)"() -> ("Value"=w701:i32)  [unwired: 2 in, 2 out]
            n408 = call <vilib>:"Add State(s) to Queue__jki_lib_state_machine.vi"("State(s) in Front (\"\")"=w703, "State(s) in (\"\")"=w706) -> ("States Out"=w698:string)  [unwired: 13 in]
            n409 = Number To Decimal String(number=w701) -> (decimal integer string=w700:string)  [unwired: 1 in]
            n410 = call <vilib>:"Build State String with Arguments__jki_lib_state_machine.vi"("Arguments (\"\")"=w700, "State"="ImgToAvg") -> ("State with Arguments"=w699:string)  [unwired: 4 in]
            n411 = call <vilib>:"Add State(s) to Queue__jki_lib_state_machine.vi"("State(s) in (\"\")"=w698, "State(s) at Back (\"\")"=w699) -> ("States Out"=w697:string)  [unwired: 13 in]
          }
          frame "Macro: Exit" {
            # "Exit Macro\n(This is called once, when the VI exits)"
            n412 = Unbundle By Name(w708) -> ("Core.Close Panel on Exit?"=w707:bool)
            n413 = Select(t="UI: Front Panel State >> Close", s=w707, f="") -> (s? t:f=w711:string)
            n414 = call <vilib>:"Add State(s) to Queue__jki_lib_state_machine.vi"("State(s) in (\"\")"=w711, "State(s) at Back (\"\")"="Data: Cleanup\nExit") -> ("States Out"=w709:string)  [unwired: 13 in]
            n415 = call <vilib>:"Add State(s) to Queue__jki_lib_state_machine.vi"("State(s) in Front (\"\")"=w709, "State(s) in (\"\")"=w716) -> ("States Out"=w715:string)  [unwired: 13 in]
          }
          frame "---------- Ini and Configure ----------" {
            # "Template Separator\n(You can make a copy of, or modify, this frame)"
            n416 = call <vilib>:"Add State(s) to Queue__jki_lib_state_machine.vi"("State(s) in (\"\")"=w720) -> ("States Out"=w719:string)  [unwired: 14 in]
          }
          frame "Device Ini" {
            # "Your code here.\n(You can make a copy of, or modify, this frame)"
            n417 = Empty String/Path?(string/path=w737) -> (empty?=w735:bool)
            n418 = case shown="False" w735 {
              tunnel: w737 -> [w774 _]
              tunnel: [w773 0] -> w736
              frame False {
                n419 = Decimal String To Number(string=w774) -> (number=w773:i32)  [unwired: 2 in, 1 out]
              }
              frame True {
              }
            }
            n420 = flat-sequence {
              tunnel: w741 -> [w777]
              tunnel: [w777] -> w740
              tunnel: w736 -> [w776]
              tunnel: w740 -> [w780]
              tunnel: [w778] -> w727
              frame #0 {
                n421 = Wait (ms)(milliseconds to wait=w776) -> ()  [unwired: 1 out]
              }
              frame #1 {
                n422 = for {
                  tunnel: w780 -> [w782] mode=indexing
                  shift-right: [w783] -> w778
                  shift-left: string[] [] -> [w784]
                  n423 = Empty String/Path?(string/path=w782) -> (empty?=w781:bool)
                  n424 = case shown="False" w781 {
                    tunnel: w784 -> [w787 w793]
                    tunnel: [w786 w793] -> w783
                    tunnel: w782 -> [w785 _]
                    frame False {
                      n425 = call "send command.vi"("Device Name"=w785) -> ("status"=w788:bool)  [unwired: 4 in]
                      n426 = case shown="False" w788 {
                        tunnel: w787 -> [w789 w792]
                        tunnel: [w789 w791] -> w786
                        tunnel: w785 -> [_ w790]
                        frame False {
                        }
                        frame True {
                          n427 = Build Array (concatenate)(w792, w790) -> (w791:string[])
                        }
                      }
                    }
                    frame True {
                    }
                  }
                }
              }
            }
            n428 = Unbundle By Name(w734) -> ("active cams"=w726:string[])
            n429 = call <vilib>:"Add State(s) to Queue__jki_lib_state_machine.vi"("State(s) in (\"\")"=w742) -> ("States Out"=w729:string)  [unwired: 14 in]
            n430 = Empty Array?(array=w726) -> (empty?=w731:bool)
            n431 = Equal?(x=w726, y=w727) -> (x = y?=w732:bool[])
            n432 = Not(x=w731) -> (.not. x?=w730:bool)
            n433 = Build Array (concatenate)(w732, w730) -> (w733:bool[])
            n434 = Array Size(array=w726) -> (size(s)=w725:i32)
            n435 = Array Size(array=w727) -> (size(s)=w724:i32)
            n436 = And Array Elements(Boolean array=w733) -> (logical AND=w722:bool)
            n437 = Equal?(x=w725, y=w724) -> (x = y?=w723:bool)
            n438 = And(x=w723, y=w722) -> (x .and. y?=w721:bool)
            n439 = case shown="False" w721 {
              tunnel: [w759 w772] -> w739
              tunnel: w734 -> [w744 w772]
              tunnel: w727 -> [w745 _]
              tunnel: w729 -> [w754 w771]
              tunnel: [w752 w771] -> w728
              frame False {
                n440 = Bundle By Name(cluster=w744, "active cams"=w745) -> (w760:T36)
                n441 = property on="active CCDs" class="LstBox (strict)"("Item Names"=w745) -> ()  [unwired: 2 in, 2 out]
                n442 = Array Size(array=w745) -> (size(s)=w763:i32)
                n443 = for {
                  N: 1 -> [_]
                  shift-right: [w765] -> w758
                  shift-left: timestamp[][] [] ("Time") -> [w767]
                  n444 = for {
                    N: 12 -> [_]
                    tunnel: w767 -> [w770] mode=indexing
                    tunnel: [w768] -> w765 mode=indexing
                    n445 = Get Date/Time In Seconds() -> (seconds since 1Jan1904=w769:timestamp)
                    n446 = Build Array (concatenate)(w770, w769) -> (w768:timestamp[])
                  }
                }
                n447 = Unbundle By Name(w744) -> ("img to avg"=w743:i32)
                n448 = Initialize Array(0.0 ("element"), w763, 0 ("dimension size")) -> (w761:dbl[][])
                n449 = Initialize Array(0.0 ("element"), 12 ("dimension size"), w743) -> (w746:dbl[][])
                n450 = Bundle By Name(cluster=w760, "Offset X stats"=w761, "Offset Y stats"=w761, "Centroid X"=w746, "Centroid Y"=w746, "Mean Centroid X"=w761, "Mean Centroid Y"=w761, "Offset X"=w761, "Offset Y"=w761, "Size"=w746, "Mean Size"=w761, "Motor X"=w761, "Motor Y"=w761) -> (w759:T36)
                n451 = property on="Time" class="Arr (strict)"("Value"=w758) -> ()  [unwired: 2 in, 2 out]
                n452 = property on="config path" class="Str"() -> ("Value"=w751:string)  [unwired: 2 in, 2 out]
                n453 = call <vilib>:"Add State(s) to Queue__jki_lib_state_machine.vi"("State(s) in Front (\"\")"="newtdms\nMove Config\nDetection Config\nactive\nCenter" ("State(s) in Front (\"\")"), "State(s) in (\"\")"=w754) -> ("States Out"=w753:string)  [unwired: 13 in]
                n454 = call <vilib>:"Build State String with Arguments__jki_lib_state_machine.vi"("Arguments (\"\")"=w751, "State"="Load Config" ("State(s) in Front (\"\")")) -> ("State with Arguments"=w749:string)  [unwired: 4 in]
                n455 = call <vilib>:"Add State(s) to Queue__jki_lib_state_machine.vi"("State(s) in Front (\"\")"=w749, "State(s) in (\"\")"=w753) -> ("States Out"=w752:string)  [unwired: 13 in]
                "name array" <- w745
              }
              frame True {
              }
            }
          }
          frame "Load Config" {
            # "Your code here.\n(You can make a copy of, or modify, this frame)"
            n456 = Unbundle By Name(w796) -> ("detection para"=w839:T3[], "move properties"=w836:T2[], "thresholds"=w831:cluster{"Lower value":sgl, "Upper value":sgl}[])
            n457 = Empty String/Path?(string/path=w795) -> (empty?=w794:bool)
            n458 = property on="Load Config" class="Bool (strict)"("Value"=FALSE ("Load Config")) -> ()  [unwired: 2 in, 2 out]
            n459 = case shown="False" w794 {
              tunnel: [w850 T5 {"CCDs"=[], "move properties"=[], "detection para"=[], "thresholds"=[], "Value"={"Motor CCD 1"=0, "Motor CCD 2"=0, "Motor CCD 3"=0, "Motor CCD 4"=0, "Motor CCD 5"=0, "Motor CCD 6"=0, "Motor CCD 7"=0, "Motor CCD 8"=0, "Motor CCD 9"=0, "Motor CCD 10"=0, "Motor CCD 11"=0, "Motor CCD 12"=0}} ("output cluster 2")] -> w841
              tunnel: [w848 w857] -> w801
              tunnel: w795 -> [w847 _]
              tunnel: w798 -> [w845 w857]
              tunnel: w796 -> [_ _]
              frame False {
                n460 = String To Path(string=w847) -> (path=w846:path)
                n461 = Open/Create/Replace File(file path (use dialog)=w846, error in=w845, operation (0:open)=T19."open or create") -> (refnum out=w852:refnum<file>, error out=w853:errorcluster)  [unwired: 3 in, 1 out]
                n462 = Read from Binary File(5:"output cluster 2", 8:w853, 11:w852) -> (0:w854:errorcluster, 2:w850:T5, 3:w855:refnum<file>)  [unwired: 3 in, 1 out]
                n463 = Close File(refnum=w855, error in=w854) -> (error out=w848:errorcluster)  [unwired: 1 out]
              }
              frame True {
              }
            }
            n464 = Unbundle By Name(w841) -> ("Value"=w828:T7, "CCDs"=w840:string[], "detection para"=w838:T3[], "move properties"=w837:T2[], "thresholds"=w832:cluster{"Lower value":sgl, "Upper value":sgl}[])
            n465 = Cluster To Array(cluster=w828) -> (array=w829:u16[])
            n466 = call <vilib>:"Add State(s) to Queue__jki_lib_state_machine.vi"("State(s) in (\"\")"=w844, "State(s) at Back (\"\")"="Motor Config" ("State(s) at Back (\"\")")) -> ("States Out"=w843:string)  [unwired: 13 in]
            n467 = for {
              tunnel: w840 -> [w873]
              tunnel: w838 -> [w875]
              tunnel: w837 -> [w874]
              shift-right: [w867] -> w835
              shift-left: w839 -> [w872]
              shift-right: [w865] -> w834
              shift-left: w836 -> [w871]
              tunnel: w797 -> [w870] mode=indexing
              tunnel: w832 -> [w866]
              shift-right: [w862] -> w830
              shift-left: w831 -> [w864]
              tunnel: w829 -> [w861]
              tunnel: [w858] -> w827 mode=indexing
              i -> [w859]
              n468 = call-poly <userlib>:"Filter 1D Array__ogtk.vi"("items to filter"=w870, "array"=w873) -> ("filtered item indices"=w876:i32[])  [unwired: 4 in, 1 out]
              n469 = Index Array(array=w876) -> (element=w860:i32)  [unwired: 1 in]
              n470 = Index Array(array=w861, index=w860) -> (element=w858:u16)
              n471 = Index Array(array=w875, index=w860) -> (element=w869:T3)
              n472 = Index Array(array=w874, index=w860) -> (element=w868:T2)
              n473 = Index Array(array=w866, index=w860) -> (element=w863:cluster{"Lower value":sgl, "Upper value":sgl})
              n474 = Replace Array Subset(array=w872, new element=w869, index=w859) -> (w867:T3[])
              n475 = Replace Array Subset(array=w871, new element=w868, index=w859) -> (w865:T2[])
              n476 = Replace Array Subset(array=w864, new element=w863, index=w859) -> (w862:cluster{"Lower value":sgl, "Upper value":sgl}[])
            }
            n477 = Index Array(array=w827, index #1=0 ("index (row)"), index #2=1 ("index (row)"), index #3=2 ("index (row)"), index #4=3 ("index (row)"), index #5=4 ("index (row)"), index #6=5 ("index (row)"), index #7=6 ("index (row)"), index #8=7 ("index (row)"), index #9=8 ("index (row)"), index #10=9 ("index (row)"), index #11=10 ("index (row)"), index #12=11 ("index (row)")) -> (element #1=w814:u16, element #2=w813:u16, element #3=w812:u16, element #4=w811:u16, element #5=w810:u16, element #6=w809:u16, element #7=w808:u16, element #8=w807:u16, element #9=w806:u16, element #10=w805:u16, element #11=w804:u16, element #12=w803:u16)
            n478 = Bundle By Name(cluster=w828, "Motor CCD 1"=w814, "Motor CCD 2"=w813, "Motor CCD 3"=w812, "Motor CCD 4"=w811, "Motor CCD 5"=w810, "Motor CCD 6"=w809, "Motor CCD 7"=w808, "Motor CCD 8"=w807, "Motor CCD 9"=w806, "Motor CCD 10"=w805, "Motor CCD 11"=w804, "Motor CCD 12"=w803) -> (w802:T7)
            n479 = Bundle By Name(cluster=w796, "detection para"=w835, "move properties"=w834, "thresholds"=w830) -> (w833:T36)
            n480 = property on="associated motors" class="Clust (strict)"(error in=w801, "Val(Sgnl)"=w802) -> (error out=w800:errorcluster)  [unwired: 1 in, 1 out]
          }
          frame "Save Config" {
            # "Your code here.\n(You can make a copy of, or modify, this frame)"
            n481 = Unbundle By Name(w894) -> ("move properties"=w880:T2[], "detection para"=w889:T3[], "thresholds"=w877:cluster{"Lower value":sgl, "Upper value":sgl}[])
            n482 = property on="associated motors" class="Clust (strict)"() -> ("Value"=w888:T7)  [unwired: 2 in, 2 out]
            n483 = property on="Save Config" class="Bool (strict)"("Value"=FALSE ("Save Config")) -> ()  [unwired: 2 in, 2 out]
            n484 = local read "CCDs"() -> (w878:string[])
            n485 = call "File Dialog"("pattern (all files)"="*.cfg", "pattern label"="config") -> ("selected path"=w882:path)  [unwired: 10 in, 3 out]
            n486 = Bundle("CCDs"=w878, "move properties"=w880, "detection para"=w889, "thresholds"=w877, "Value"=w888) -> (w881:T5)  [unwired: 1 in]
            n487 = Open/Create/Replace File(file path (use dialog)=w882, error in=w886, operation (0:open)=T19."replace or create with confirmation") -> (refnum out=w890:refnum<file>, error out=w891:errorcluster)  [unwired: 3 in, 1 out]
            n488 = Write to Binary File(file (use dialog)=w890, data=w881, error in=w891) -> (refnum out=w893:refnum<file>, error out=w892:errorcluster)  [unwired: 3 in, 1 out]
            n489 = Close File(refnum=w893, error in=w892) -> (error out=w885:errorcluster)  [unwired: 1 out]
            n490 = call <vilib>:"Add State(s) to Queue__jki_lib_state_machine.vi"("State(s) in (\"\")"=w896) -> ("States Out"=w895:string)  [unwired: 14 in]
          }
          frame "active" {
            # "Your code here.\n(You can make a copy of, or modify, this frame)"
            n491 = call-poly <userlib>:"Filter 1D Array__ogtk.vi"("items to filter"=w906, "array"=w902) -> ("filtered item indices"=w905:i32[])  [unwired: 4 in, 1 out]
            n492 = Unbundle By Name(w901) -> ("move properties"=w904:T2[], "detection para"=w899:T3[])  [unwired: 1 out]
            n493 = Index Array(array=w905) -> (element=w897:i32)  [unwired: 1 in]
            n494 = Index Array(array=w904, index=w897) -> (element=w903:T2)
            n495 = Index Array(array=w899, index=w897) -> (element=w898:T3)
            n496 = property on="move config" class="Clust (strict)"("Value"=w903) -> ()  [unwired: 2 in, 2 out]
            n497 = property on="beam detection para" class="Clust (strict)"("Value"=w898) -> ()  [unwired: 2 in, 2 out]
            n498 = Bundle By Name(cluster=w901, "active ccd"=w897) -> (w900:T36)
            n499 = call <vilib>:"Add State(s) to Queue__jki_lib_state_machine.vi"("State(s) in (\"\")"=w909) -> ("States Out"=w908:string)  [unwired: 14 in]
          }
          frame "Detection Config" {
            # "Your code here.\n(You can make a copy of, or modify, this frame)"
            n500 = Unbundle By Name(w914) -> ("detection para"=w910:T3[], "active ccd"=w915:i32)
            n501 = Replace Array Subset(array=w910, new element="beam detection para", index=w915) -> (w911:T3[])
            n502 = Bundle By Name(cluster=w914, "detection para"=w911) -> (w913:T36)
            n503 = call <vilib>:"Add State(s) to Queue__jki_lib_state_machine.vi"("State(s) in (\"\")"=w918) -> ("States Out"=w917:string)  [unwired: 14 in]
          }
          frame "Motor Config" {
            # "Your code here.\n(You can make a copy of, or modify, this frame)"
            n504 = Unbundle By Name("associated motors") -> ("Motor CCD 1"=w940:u16, "Motor CCD 2"=w941:u16, "Motor CCD 3"=w942:u16, "Motor CCD 4"=w935:u16, "Motor CCD 5"=w934:u16, "Motor CCD 6"=w933:u16, "Motor CCD 7"=w932:u16, "Motor CCD 8"=w931:u16, "Motor CCD 9"=w930:u16, "Motor CCD 10"=w929:u16, "Motor CCD 11"=w928:u16, "Motor CCD 12"=w927:u16)
            n505 = local read "motor refs"() -> (w938:refnum<vi>[])
            n506 = property on="ActiveMotor" class="Ring (strict)"() -> ("Value"=w921:u16)  [unwired: 2 in, 2 out]
            n507 = property on="ActiveMotor" class="Ring (strict)"() -> ("Strings []"=w923:string[])  [unwired: 2 in, 2 out]
            n508 = Build Array(w940, w941, w942, w935, w934, w933, w932, w931, w930, w929, w928, w927) -> (w926:u16[])
            n509 = Increment(x=w926) -> (x+1=w925:u16[])
            n510 = Index Array(array=w923, index=w921) -> (element=w922:string)
            n511 = for {
              tunnel: w925 -> [w957] mode=indexing
              tunnel: w938 -> [w952]
              tunnel: [w948] -> w924 mode=indexing
              tunnel: [w947] -> w920 mode=indexing
              tunnel: [w946] -> w919 mode=indexing
              n512 = Multiply(x=w957, y=u16 3) -> (x*y=w953:u16)
              n513 = Subtract(x=w953, y=u16 3) -> (x-y=w947:u16)
              n514 = Subtract(x=w953, y=u16 2) -> (x-y=w946:u16)
              n515 = Index Array(array=w952, index=w947) -> (element=w951:refnum<vi>)
              n516 = Index Array(array=w952, index=w946) -> (element=w950:refnum<vi>)
              n517 = Bundle By Name(cluster="active Axis ref", "Ref X"=w951, "Ref Y"=w950) -> (w948:cluster{"Ref X":refnum<vi>, "Ref Y":refnum<vi>})
            }
            "Array" <- w920
            "Array 2" <- w919
            n518 = property on="ActiveMotorName::99" class="Str"("Val(Sgnl)"=w922) -> ()  [unwired: 2 in, 2 out]
            n519 = call <vilib>:"Add State(s) to Queue__jki_lib_state_machine.vi"("State(s) in (\"\")"=w945) -> ("States Out"=w944:string)  [unwired: 14 in]
            n520 = Bundle By Name(cluster=w937, "active axis refs 2"=w924) -> (w936:T36)
          }
          frame "Move Config" {
            # "Your code here.\n(You can make a copy of, or modify, this frame)"
            n521 = Unbundle By Name(w959) -> ("move properties"=w963:T2[], "active ccd"=w962:i32)
            n522 = Replace Array Subset(array=w963, new element="move config", index=w962) -> (w960:T2[])
            n523 = Bundle By Name(cluster=w959, "move properties"=w960) -> (w958:T36)
            n524 = call <vilib>:"Add State(s) to Queue__jki_lib_state_machine.vi"("State(s) in (\"\")"=w966) -> ("States Out"=w965:string)  [unwired: 14 in]
          }
          frame "----------Centroid & Move----------" {
            # "Template Separator\n(You can make a copy of, or modify, this frame)"
            n525 = call <vilib>:"Add State(s) to Queue__jki_lib_state_machine.vi"("State(s) in (\"\")"=w970) -> ("States Out"=w969:string)  [unwired: 14 in]
          }
          frame "detected" {
            n526 = Unbundle By Name(w973) -> ("Offset X"=w1015:dbl[][], "Offset Y"=w1014:dbl[][], "Size"=w1013:dbl[][], "Mean Size"=w1012:dbl[][], "Time"=w1009:timestamp[][], "Motor X"=w987:dbl[][], "active axis refs 2"=w986:T12, "Motor Y"=w985:dbl[][])
            n527 = Spreadsheet String To Array(format string="%s", spreadsheet string=w991, array type (2D Dbl)=string[] []) -> (array=w980:string[])  [unwired: 1 in]
            n528 = call-poly <userlib>:"Filter 1D Array__ogtk.vi"("items to filter"=w980, "array"=w981) -> ("filtered item indices"=w978:i32[])  [unwired: 4 in, 1 out]
            n529 = for {
              tunnel: w981 -> [w1032] mode=indexing
              tunnel: w980 -> [w1031]
              tunnel: [w1029] -> w982 mode=indexing
              n530 = for {
                tunnel: w1032 -> [w1035]
                tunnel: [w1034] -> w1030 mode=indexing
                tunnel: w1031 -> [w1033] mode=indexing
                n531 = Equal?(x=w1035, y=w1033) -> (x = y?=w1034:bool)
              }
              n532 = Or Array Elements(Boolean array=w1030) -> (logical OR=w1029:bool)
            }
            n533 = for {
              N: 12 -> [_]
              tunnel: w978 -> [w1028]
              tunnel: [w1025] -> w977 mode=indexing
              i -> [w1027]
              n534 = Equal?(x=w1028, y=w1027) -> (x = y?=w1026:bool[])
              n535 = Or Array Elements(Boolean array=w1026) -> (logical OR=w1025:bool)
            }
            "Array 3" <- w977
            n536 = call <vilib>:"Build State String with Arguments__jki_lib_state_machine.vi"("Arguments (\"\")"=w991, "State"="stats") -> ("State with Arguments"=w990:string)  [unwired: 4 in]
            n537 = Unbundle By Name(w973) -> ("Mean Centroid X"=w1020:dbl[][], "Mean Centroid Y"=w1019:dbl[][], "Centroid X"=w1022:dbl[][], "Centroid Y"=w1021:dbl[][])
            n538 = call <vilib>:"Add State(s) to Queue__jki_lib_state_machine.vi"("State(s) in (\"\")"=w989, "State(s) at Back (\"\")"=w990) -> ("States Out"=w988:string)  [unwired: 13 in]
            n539 = for {
              tunnel: w1022 -> [w1085]
              tunnel: w1021 -> [w1084]
              tunnel: w1020 -> [w1083]
              tunnel: w1019 -> [w1082]
              tunnel: [w1081] -> w1006 mode=indexing
              tunnel: [w1080] -> w1017 mode=indexing
              tunnel: w1016 -> [w1053] mode=indexing
              tunnel: w1015 -> [w1079]
              tunnel: w1014 -> [w1078]
              tunnel: [w1077] -> w994 mode=indexing
              tunnel: [w1076] -> w1007 mode=indexing
              tunnel: w1013 -> [w1075]
              tunnel: w1012 -> [w1074]
              tunnel: [w1073] -> w1011 mode=indexing
              tunnel: w1009 -> [w1072]
              tunnel: [w1071] -> w1008 mode=indexing
              tunnel: w987 -> [w1045]
              tunnel: w986 -> [w1044]
              tunnel: w985 -> [w1043]
              tunnel: [w1042] -> w984 mode=indexing
              tunnel: [w1041] -> w983 mode=indexing
              tunnel: w982 -> [w1040]
              i -> [w1039]
              n540 = Unbundle By Name(w1053) -> ("Target.X::12"=w1056:refnum<vi>, "Target.Y::12"=w1055:refnum<vi>)
              n541 = Index Array(array=w1045, index (row)=w1039) -> (element=w1048:dbl[])  [unwired: 1 in]
              n542 = Index Array(array=w1044, index=w1039) -> (element=w1047:cluster{"Ref X":refnum<vi>, "Ref Y":refnum<vi>})
              n543 = Index Array(array=w1043, index (row)=w1039) -> (element=w1052:dbl[])  [unwired: 1 in]
              n544 = Index Array(array=w1083, index (row)=w1039) -> (element=w1067:dbl[])  [unwired: 1 in]
              n545 = Index Array(array=w1082, index (row)=w1039) -> (element=w1068:dbl[])  [unwired: 1 in]
              n546 = Index Array(array=w1085, index (row)=w1039) -> (element=w1070:dbl[])  [unwired: 1 in]
              n547 = Index Array(array=w1084, index (row)=w1039) -> (element=w1069:dbl[])  [unwired: 1 in]
              n548 = Index Array(array=w1079, index (row)=w1039) -> (element=w1064:dbl[])  [unwired: 1 in]
              n549 = Index Array(array=w1078, index (row)=w1039) -> (element=w1063:dbl[])  [unwired: 1 in]
              n550 = Index Array(array=w1075, index (row)=w1039) -> (element=w1061:dbl[])  [unwired: 1 in]
              n551 = Index Array(array=w1074, index (row)=w1039) -> (element=w1060:dbl[])  [unwired: 1 in]
              n552 = Index Array(array=w1072, index (row)=w1039) -> (element=w1057:timestamp[])  [unwired: 1 in]
              n553 = Index Array(array=w1040, index=w1039) -> (element=w1038:bool)
              n554 = Unbundle By Name(w1047) -> ("Ref X"=w1046:refnum<vi>, "Ref Y"=w1050:refnum<vi>)
              n555 = property class="DigNum (strict)"(reference=w1056) -> ("Value"=w1037:dbl)  [unwired: 1 in, 2 out]
              n556 = property class="DigNum (strict)"(reference=w1055) -> ("Value"=w1054:dbl)  [unwired: 1 in, 2 out]
              n557 = call <vilib>:"Std Deviation and Variance.vi"("X"=w1070) -> ("mean"=w1036:dbl)  [unwired: 1 in, 2 out]
              n558 = call <vilib>:"Std Deviation and Variance.vi"("X"=w1069) -> ("mean"=w1066:dbl)  [unwired: 1 in, 2 out]
              n559 = call <vilib>:"Std Deviation and Variance.vi"("X"=w1061) -> ("mean"=w1059:dbl)  [unwired: 1 in, 2 out]
              n560 = Get Date/Time In Seconds() -> (seconds since 1Jan1904=w1058:timestamp)
              n561 = property class="DigNum (strict)"(reference=w1046) -> ("Value"=w1049:dbl)  [unwired: 1 in, 2 out]
              n562 = property class="DigNum (strict)"(reference=w1050) -> ("Value"=w1051:dbl)  [unwired: 1 in, 2 out]
              n563 = Subtract(x=w1037, y=w1036) -> (x-y=w1065:dbl)
              n564 = Subtract(x=w1054, y=w1066) -> (x-y=w1062:dbl)
              n565 = case shown="True" w1038 {
                tunnel: [w1103 w1117] -> w1081
                tunnel: [w1102 w1116] -> w1080
                tunnel: [w1101 w1115] -> w1077
                tunnel: [w1100 w1114] -> w1076
                tunnel: [w1099 w1113] -> w1073
                tunnel: [w1098 w1112] -> w1071
                tunnel: w1068 -> [w1097 w1111]
                tunnel: w1067 -> [w1096 w1110]
                tunnel: w1036 -> [w1095 _]
                tunnel: w1066 -> [w1094 _]
                tunnel: w1065 -> [w1093 _]
                tunnel: w1064 -> [w1092 w1109]
                tunnel: w1063 -> [w1091 w1108]
                tunnel: w1062 -> [w1090 _]
                tunnel: w1060 -> [w1089 w1107]
                tunnel: w1059 -> [w1088 _]
                tunnel: w1058 -> [w1087 w1106]
                tunnel: w1057 -> [w1086 w1105]
                frame True {
                  n566 = Build Array (concatenate)(w1096, w1095) -> (w1103:dbl[])
                  n567 = Build Array (concatenate)(w1097, w1094) -> (w1102:dbl[])
                  n568 = Build Array (concatenate)(w1092, w1093) -> (w1101:dbl[])
                  n569 = Build Array (concatenate)(w1091, w1090) -> (w1100:dbl[])
                  n570 = Build Array (concatenate)(w1089, w1088) -> (w1099:dbl[])
                  n571 = Build Array (concatenate)(w1086, w1087) -> (w1098:timestamp[])
                }
                frame False {
                  w1104 = 0.0
                  n572 = Build Array (concatenate)(w1110, w1104) -> (w1117:dbl[])
                  n573 = Build Array (concatenate)(w1111, w1104) -> (w1116:dbl[])
                  n574 = Build Array (concatenate)(w1109, w1104) -> (w1115:dbl[])
                  n575 = Build Array (concatenate)(w1108, w1104) -> (w1114:dbl[])
                  n576 = Build Array (concatenate)(w1107, w1104) -> (w1113:dbl[])
                  n577 = Build Array (concatenate)(w1105, w1106) -> (w1112:timestamp[])
                }
              }
              n578 = Build Array (concatenate)(w1052, w1051) -> (w1041:dbl[])
              n579 = Build Array (concatenate)(w1048, w1049) -> (w1042:dbl[])
            }
            n580 = local write "Numeric"(0.0 ("Numeric")) -> ()
            n581 = Array Size(array=w994) -> (size(s)=w1005:i32[])
            n582 = Index Array(array=w1005, index=1) -> (element=w1003:i32)
            "History index" <- w1003
            n583 = call <vilib>:"Add State(s) to Queue__jki_lib_state_machine.vi"("State(s) in (\"\")"=w988, "State(s) at Back (\"\")"="Check Move\ntdms" ("State(s) at Back (\"\")")) -> ("States Out"=w997:string)  [unwired: 13 in]
            n584 = Unbundle By Name(w973) -> ("img to avg"=w972:i32)
            n585 = Decrement(x=w972) -> (x-1=w971:i32)
            n586 = Initialize Array(0.0 ("element"), 12 ("dimension size"), w971) -> (w974:dbl[][])
            n587 = Greater?(x=w1003, y="History Size") -> (0:w1001:bool)
            n588 = Bundle By Name(cluster=w973, "Centroid X"=w974, "Centroid Y"=w974, "Mean Centroid X"=w1006, "Mean Centroid Y"=w1017, "Offset X"=w994, "Offset Y"=w1007, "Mean Size"=w1011, "Size"=w974, "Time"=w1008, "Motor X"=w984, "Motor Y"=w983) -> (w1018:T36)
            n589 = Select(t="history" ("State(s) at Back (\"\")"), s=w1001, f="") -> (s? t:f=w998:string)
            n590 = call <vilib>:"Add State(s) to Queue__jki_lib_state_machine.vi"("State(s) in (\"\")"=w997, "State(s) at Back (\"\")"=w998) -> ("States Out"=w996:string)  [unwired: 13 in]
          }
          frame "Check Move" {
            (unwired) "Device Ini" ("State(s) in Front (\"\")")
            # "Your code here.\n(You can make a copy of, or modify, this frame)"
            n591 = Unbundle By Name(w1122) -> ("move properties"=w1125:T2[], "Mean Size"=w1148:dbl[][], "move properties"=w1151:T2[], "Offset X"=w1150:dbl[][], "Offset Y"=w1149:dbl[][], "active cams"=w1129:string[])
            n592 = for {
              tunnel: w1151 -> [w1216]
              tunnel: w1150 -> [w1215]
              tunnel: w1149 -> [w1214]
              tunnel: w1148 -> [w1217]
              tunnel: [w1233] -> w1147 mode=indexing
              tunnel: [w1229] -> w1146 mode=indexing
              tunnel: w1129 -> [w1219] mode=indexing
              tunnel: [w1251] -> w1145 mode=indexing
              tunnel: [w1250] -> w1144 mode=indexing
              tunnel: w1125 -> [w1209]
              tunnel: [w1227] -> w1123 mode=indexing
              tunnel: [w1222] -> w1119 mode=indexing
              tunnel: "Speedmode @" -> [w1221]
              tunnel: w1118 -> [w1220]
              n593 = call-poly <userlib>:"Filter 1D Array__ogtk.vi"("items to filter"=w1219, "array"=w1220) -> ("filtered item indices"=w1218:i32[])  [unwired: 4 in, 1 out]
              n594 = Index Array(array=w1218) -> (element=w1208:i32)  [unwired: 1 in]
              n595 = Index Array(array=w1217, index (row)=w1208) -> (element=w1213:dbl[])  [unwired: 1 in]
              n596 = Index Array(array=w1216, index=w1208) -> (element=w1212:T2)
              n597 = Index Array(array=w1215, index (row)=w1208) -> (element=w1211:dbl[])  [unwired: 1 in]
              n598 = Index Array(array=w1209, index=w1208) -> (element=w1207:T2)
              n599 = Index Array(array=w1214, index (row)=w1208) -> (element=w1210:dbl[])  [unwired: 1 in]
              n600 = Unbundle By Name(w1212) -> ("Tolerance [%]"=w1244:dbl)
              n601 = Reverse 1D Array(array=w1211) -> (reversed array=w1249:dbl[])
              n602 = Reverse 1D Array(array=w1210) -> (reversed array=w1248:dbl[])
              n603 = Reverse 1D Array(array=w1213) -> (reversed array=w1243:dbl[])
              n604 = Unbundle By Name(w1207) -> ("enable feedback"=w1232:bool)
              n605 = Index Array(array=w1249) -> (element=w1247:dbl)  [unwired: 1 in]
              n606 = Index Array(array=w1248) -> (element=w1246:dbl)  [unwired: 1 in]
              n607 = Index Array(array=w1243) -> (element=w1242:dbl)  [unwired: 1 in]
              n608 = Absolute Value(x=w1247) -> (abs(x)=w1228:dbl)
              n609 = Absolute Value(x=w1246) -> (abs(x)=w1225:dbl)
              n610 = Square Root(x=w1242) -> (sqrt(x)=w1241:dbl)
              n611 = Divide(x=w1244, y=100.0) -> (x/y=w1240:dbl)
              n612 = Multiply(x=w1241, y=w1240) -> (x*y=w1224:dbl)
              n613 = Not Equal To 0?(x=w1225) -> (x != 0?=w1230:bool)
              n614 = Not Equal To 0?(x=w1228) -> (x != 0?=w1235:bool)
              n615 = Greater Or Equal?(x=w1228, y=w1224) -> (x >= y?=w1234:bool)
              n616 = Greater Or Equal?(x=w1225, y=w1224) -> (x >= y?=w1231:bool)
              n617 = Divide(x=w1228, y=w1224) -> (x/y=w1226:dbl)
              n618 = Divide(x=w1225, y=w1224) -> (x/y=w1223:dbl)
              n619 = Compound Arithmetic op=AND(w1232, w1235, w1234) -> (w1233:bool)
              n620 = Compound Arithmetic op=AND(w1232, w1231, w1230) -> (w1229:bool)
              n621 = Boolean To (0,1)(Boolean=w1229) -> (0, 1=w1236:i16)
              n622 = Greater?(x=w1226, y=w1221) -> (0:w1227:bool)
              n623 = Greater?(x=w1223, y=w1221) -> (0:w1222:bool)
              n624 = Multiply(x=w1236, y=w1225) -> (x*y=w1237:dbl)
              n625 = Boolean To (0,1)(Boolean=w1233) -> (0, 1=w1239:i16)
              n626 = Multiply(x=w1239, y=w1228) -> (x*y=w1238:dbl)
              n627 = Bundle(w1237, "GUIdevice 8"=w1219) -> (w1250:cluster{dbl, "GUIdevice 8":string})  [unwired: 1 in]
              n628 = Bundle(w1238, "GUIdevice 8"=w1219) -> (w1251:cluster{dbl, "GUIdevice 8":string})  [unwired: 1 in]
            }
            "required X" <- w1147
            "required Y" <- w1146
            "speedmode X" <- w1123
            "speedmode Y" <- w1119
            n629 = case shown="True" "Align" {
              tunnel: w1145 -> [w1159 w1164]
              tunnel: w1144 -> [w1158 w1161]
              tunnel: [w1157 w1163] -> w1141
              tunnel: [w1156 w1160] -> w1135
              frame False {
                n630 = Sort 1D Array(array=w1158) -> (sorted array=w1155:cluster{dbl, "GUIdevice 8":string}[])
                n631 = Sort 1D Array(array=w1159) -> (sorted array=w1154:cluster{dbl, "GUIdevice 8":string}[])
                n632 = Reverse 1D Array(array=w1155) -> (reversed array=w1156:cluster{dbl, "GUIdevice 8":string}[])
                n633 = Reverse 1D Array(array=w1154) -> (reversed array=w1157:cluster{dbl, "GUIdevice 8":string}[])
              }
              frame True {
                w1162 = cluster{dbl, "GUIdevice 8":string}[] [] ("Array")
                n634 = for {
                  shift-right: [w1174] -> w1163
                  shift-left: w1162 -> [w1176]
                  tunnel: w1164 -> [w1175] mode=indexing
                  n635 = Unbundle(w1175) -> (w1178:dbl)  [unwired: 1 out]
                  n636 = Not Equal To 0?(x=w1178) -> (x != 0?=w1177:bool)
                  n637 = case shown="True" w1177 {
                    tunnel: w1176 -> [w1179 w1182]
                    tunnel: w1175 -> [_ w1181]
                    tunnel: [w1179 w1180] -> w1174
                    frame False {
                    }
                    frame True {
                      n638 = Build Array (concatenate)(w1182, w1181) -> (w1180:cluster{dbl, "GUIdevice 8":string}[])
                    }
                  }
                }
                n639 = for {
                  shift-right: [w1165] -> w1160
                  shift-left: w1162 -> [w1167]
                  tunnel: w1161 -> [w1166] mode=indexing
                  n640 = Unbundle(w1166) -> (w1169:dbl)  [unwired: 1 out]
                  n641 = Not Equal To 0?(x=w1169) -> (x != 0?=w1168:bool)
                  n642 = case shown="True" w1168 {
                    tunnel: w1167 -> [w1170 w1173]
                    tunnel: w1166 -> [_ w1172]
                    tunnel: [w1170 w1171] -> w1165
                    frame False {
                    }
                    frame True {
                      n643 = Build Array (concatenate)(w1173, w1172) -> (w1171:cluster{dbl, "GUIdevice 8":string}[])
                    }
                  }
                }
              }
            }
            n644 = call <vilib>:"Add State(s) to Queue__jki_lib_state_machine.vi"("State(s) in (\"\")"=w1128) -> ("States Out"=w1127:string)  [unwired: 14 in]
            n645 = Bundle By Name(cluster=w1122, "speedmode X"=w1123, "speedmode Y"=w1119) -> (w1121:T36)
            n646 = Empty Array?(array=w1141) -> (empty?=w1138:bool)
            n647 = Empty Array?(array=w1135) -> (empty?=w1133:bool)
            n648 = Index Array(array=w1141) -> (element=w1131:cluster{dbl, "GUIdevice 8":string})  [unwired: 1 in]
            n649 = Index Array(array=w1135) -> (element=w1130:cluster{dbl, "GUIdevice 8":string})  [unwired: 1 in]
            n650 = Unbundle(w1131) -> (w1140:dbl)  [unwired: 1 out]
            n651 = Unbundle(w1130) -> (w1136:dbl)  [unwired: 1 out]
            n652 = Equal To 0?(x=w1140) -> (x = 0?=w1139:bool)
            n653 = Equal To 0?(x=w1136) -> (x = 0?=w1134:bool)
            n654 = property on="autodetect" class="Bool (strict)"("Value"=FALSE ("autodetect")) -> ()  [unwired: 2 in, 2 out]
            n655 = Unbundle By Name(w1121) -> ("Feedback global"=w1142:bool)
            n656 = Or(x=w1139, y=w1138) -> (x .or. y?=w1137:bool)
            n657 = Or(x=w1134, y=w1133) -> (x .or. y?=w1132:bool)
            n658 = case shown="True" w1142 {
              tunnel: w1137 -> [_ w1190]
              tunnel: w1141 -> [_ w1189]
              tunnel: w1132 -> [_ w1187]
              tunnel: w1135 -> [_ w1186]
              tunnel: w1127 -> [w1183 w1185]
              tunnel: [w1183 w1184] -> w1143
              frame False {
              }
              frame True {
                n659 = case shown="False" w1190 {
                  tunnel: w1189 -> [w1205 _]
                  tunnel: w1185 -> [w1201 w1206]
                  tunnel: [w1199 w1206] -> w1188
                  frame False {
                    n660 = Index Array(array=w1205) -> (element=w1204:cluster{dbl, "GUIdevice 8":string})  [unwired: 1 in]
                    n661 = Unbundle By Name(w1204) -> ("GUIdevice 8"=w1203:string)
                    n662 = call <vilib>:"Build State String with Arguments__jki_lib_state_machine.vi"("Arguments (\"\")"=w1203, "State"="Move X") -> ("State with Arguments"=w1200:string)  [unwired: 4 in]
                    n663 = call <vilib>:"Add State(s) to Queue__jki_lib_state_machine.vi"("State(s) in (\"\")"=w1201, "State(s) at Back (\"\")"=w1200) -> ("States Out"=w1199:string)  [unwired: 13 in]
                  }
                  frame True {
                  }
                }
                n664 = case shown="False" w1187 {
                  tunnel: w1186 -> [w1197 _]
                  tunnel: w1188 -> [w1193 w1198]
                  tunnel: [w1191 w1198] -> w1184
                  frame False {
                    n665 = Index Array(array=w1197) -> (element=w1196:cluster{dbl, "GUIdevice 8":string})  [unwired: 1 in]
                    n666 = Unbundle By Name(w1196) -> ("GUIdevice 8"=w1195:string)
                    n667 = call <vilib>:"Build State String with Arguments__jki_lib_state_machine.vi"("Arguments (\"\")"=w1195, "State"="Move Y") -> ("State with Arguments"=w1192:string)  [unwired: 4 in]
                    n668 = call <vilib>:"Add State(s) to Queue__jki_lib_state_machine.vi"("State(s) in (\"\")"=w1193, "State(s) at Back (\"\")"=w1192) -> ("States Out"=w1191:string)  [unwired: 13 in]
                  }
                  frame True {
                  }
                }
              }
            }
            n669 = call <vilib>:"Add State(s) to Queue__jki_lib_state_machine.vi"("State(s) in (\"\")"=w1127, "State(s) at Back (\"\")"=w1143) -> ("States Out"=w1153:string)  [unwired: 13 in]
          }
          frame "Move X" {
            # "Your code here.\n(You can make a copy of, or modify, this frame)"
            n670 = Unbundle By Name(w1275) -> ("Offset X"=w1252:dbl[][])
            n671 = call-poly <userlib>:"Filter 1D Array__ogtk.vi"("items to filter"=w1260, "array"=w1279) -> ("filtered item indices"=w1264:i32[])  [unwired: 4 in, 1 out]
            n672 = Unbundle By Name(w1275) -> ("speedmode X"=w1259:bool[], "active axis refs 2"=w1278:T12, "move properties"=w1263:T2[])
            n673 = for {
              tunnel: w1264 -> [w1284] mode=indexing
              tunnel: w1263 -> [w1288]
              shift-right: [w1283] -> w1261
              shift-left: i32[] [] ("filtered item indices") -> [w1286]
              n674 = Index Array(array=w1288, index=w1284) -> (element=w1287:T2)
              n675 = Unbundle By Name(w1287) -> ("enable feedback"=w1285:bool)
              n676 = case shown="True" w1285 {
                tunnel: w1286 -> [w1289 w1292]
                tunnel: w1284 -> [_ w1291]
                tunnel: [w1289 w1290] -> w1283
                frame False {
                }
                frame True {
                  n677 = Build Array (concatenate)(w1292, w1291) -> (w1290:i32[])
                }
              }
            }
            n678 = Index Array(array=w1261) -> (element=w1258:i32)  [unwired: 1 in]
            n679 = Index Array(array=w1252, index (row)=w1258) -> (element=w1274:dbl[])  [unwired: 1 in]
            n680 = Reverse 1D Array(array=w1274) -> (reversed array=w1273:dbl[])
            n681 = Index Array(array=w1278, index=w1258) -> (element=w1277:cluster{"Ref X":refnum<vi>, "Ref Y":refnum<vi>})
            n682 = Index Array(array=w1273) -> (element=w1271:dbl)  [unwired: 1 in]
            n683 = Index Array(array=w1263, index=w1258) -> (element=w1276:T2)
            n684 = Unbundle By Name(w1277) -> ("Ref X"=w1268:refnum<vi>, "Ref Y"=w1267:refnum<vi>)
            n685 = Index Array(array=w1259, index=w1258) -> (element=w1257:bool)
            n686 = Unbundle By Name(w1276) -> ("Invert Direction X"=w1269:bool, "Invert Axis"=w1272:bool, "Stepsize"=w1255:dbl, "enable feedback"=w1266:bool)
            n687 = Greater Or Equal To 0?(x=w1271) -> (x >= 0?=w1270:bool)
            n688 = call <vilib>:"Add State(s) to Queue__jki_lib_state_machine.vi"("State(s) in Front (\"\")"="Wait" ("State(s) in Front (\"\")"), "State(s) in (\"\")"=w1282) -> ("States Out"=w1281:string)  [unwired: 13 in]
            n689 = property on="Speedmode @" class="DigNum (strict)"() -> ("Value"=w1254:dbl)  [unwired: 2 in, 2 out]
            n690 = Multiply(x=w1254, y=w1255) -> (x*y=w1256:dbl)
            n691 = Select(t=w1256, s=w1257, f=w1255) -> (s? t:f=w1253:dbl)
            n692 = case shown="True" w1266 {
              tunnel: w1272 -> [_ w1298]
              tunnel: w1270 -> [_ w1297]
              tunnel: w1253 -> [_ w1296]
              tunnel: w1269 -> [_ w1295]
              tunnel: w1268 -> [_ w1294]
              tunnel: w1267 -> [_ w1293]
              frame False {
              }
              frame True {
                n693 = case shown="False" w1297 {
                  tunnel: w1295 -> [w1306 w1328]
                  tunnel: w1296 -> [w1304 w1326]
                  tunnel: w1298 -> [w1303 w1325]
                  tunnel: w1298 -> [w1302 w1324]
                  tunnel: w1294 -> [w1300 w1322]
                  tunnel: w1293 -> [w1299 w1321]
                  frame True {
                    n694 = case shown="False" w1303 {
                      tunnel: [w1317 w1319] -> w1305
                      tunnel: w1300 -> [w1318 _]
                      tunnel: w1299 -> [_ w1320]
                      frame False {
                        n695 = property class="DigNum (strict)"(reference=w1318) -> ("Value"=w1317:dbl)  [unwired: 1 in, 2 out]
                      }
                      frame True {
                        n696 = property class="DigNum (strict)"(reference=w1320) -> ("Value"=w1319:dbl)  [unwired: 1 in, 2 out]
                      }
                    }
                    n697 = case shown="False" w1306 {
                      tunnel: w1305 -> [w1313 w1316]
                      tunnel: w1304 -> [w1312 w1315]
                      tunnel: [w1311 w1314] -> w1301
                      frame False {
                        n698 = Add(x=w1313, y=w1312) -> (x+y=w1311:dbl)
                      }
                      frame True {
                        n699 = Subtract(x=w1316, y=w1315) -> (x-y=w1314:dbl)
                      }
                    }
                    n700 = case shown="False" w1302 {
                      tunnel: w1301 -> [w1307 w1309]
                      tunnel: w1300 -> [w1308 _]
                      tunnel: w1299 -> [_ w1310]
                      frame False {
                        n701 = property class="DigNum (strict)"(reference=w1308, "Val(Sgnl)"=w1307) -> ()  [unwired: 1 in, 2 out]
                      }
                      frame True {
                        n702 = property class="DigNum (strict)"(reference=w1310, "Val(Sgnl)"=w1309) -> ()  [unwired: 1 in, 2 out]
                      }
                    }
                  }
                  frame False {
                    n703 = case shown="False" w1325 {
                      tunnel: [w1339 w1341] -> w1327
                      tunnel: w1322 -> [w1340 _]
                      tunnel: w1321 -> [_ w1342]
                      frame False {
                        n704 = property class="DigNum (strict)"(reference=w1340) -> ("Value"=w1339:dbl)  [unwired: 1 in, 2 out]
                      }
                      frame True {
                        n705 = property class="DigNum (strict)"(reference=w1342) -> ("Value"=w1341:dbl)  [unwired: 1 in, 2 out]
                      }
                    }
                    n706 = case shown="False" w1328 {
                      tunnel: w1327 -> [w1335 w1338]
                      tunnel: w1326 -> [w1334 w1337]
                      tunnel: [w1333 w1336] -> w1323
                      frame False {
                        n707 = Subtract(x=w1335, y=w1334) -> (x-y=w1333:dbl)
                      }
                      frame True {
                        n708 = Add(x=w1338, y=w1337) -> (x+y=w1336:dbl)
                      }
                    }
                    n709 = case shown="False" w1324 {
                      tunnel: w1323 -> [w1329 w1331]
                      tunnel: w1322 -> [w1330 _]
                      tunnel: w1321 -> [_ w1332]
                      frame False {
                        n710 = property class="DigNum (strict)"(reference=w1330, "Val(Sgnl)"=w1329) -> ()  [unwired: 1 in, 2 out]
                      }
                      frame True {
                        n711 = property class="DigNum (strict)"(reference=w1332, "Val(Sgnl)"=w1331) -> ()  [unwired: 1 in, 2 out]
                      }
                    }
                  }
                }
              }
            }
            "Arguments X" <- w1260
            "Moving X" <- w1260
          }
          frame "Move Y" {
            # "Your code here.\n(You can make a copy of, or modify, this frame)"
            n712 = Unbundle By Name(w1366) -> ("Offset Y"=w1365:dbl[][])
            n713 = call-poly <userlib>:"Filter 1D Array__ogtk.vi"("items to filter"=w1350, "array"=w1370) -> ("filtered item indices"=w1355:i32[])  [unwired: 4 in, 1 out]
            n714 = Unbundle By Name(w1366) -> ("speedmode Y"=w1349:bool[], "active axis refs 2"=w1369:T12, "move properties"=w1353:T2[])
            n715 = for {
              tunnel: w1355 -> [w1375] mode=indexing
              tunnel: w1353 -> [w1379]
              shift-right: [w1374] -> w1354
              shift-left: i32[] [] ("filtered item indices") -> [w1377]
              n716 = Index Array(array=w1379, index=w1375) -> (element=w1378:T2)
              n717 = Unbundle By Name(w1378) -> ("enable feedback"=w1376:bool)
              n718 = case shown="True" w1376 {
                tunnel: w1377 -> [w1380 w1383]
                tunnel: w1375 -> [_ w1382]
                tunnel: [w1380 w1381] -> w1374
                frame False {
                }
                frame True {
                  n719 = Build Array (concatenate)(w1383, w1382) -> (w1381:i32[])
                }
              }
            }
            n720 = Index Array(array=w1354) -> (element=w1348:i32)  [unwired: 1 in]
            n721 = Index Array(array=w1365, index (row)=w1348) -> (element=w1364:dbl[])  [unwired: 1 in]
            n722 = Reverse 1D Array(array=w1364) -> (reversed array=w1363:dbl[])
            n723 = Index Array(array=w1369, index=w1348) -> (element=w1368:cluster{"Ref X":refnum<vi>, "Ref Y":refnum<vi>})
            n724 = Index Array(array=w1363) -> (element=w1361:dbl)  [unwired: 1 in]
            n725 = Index Array(array=w1353, index=w1348) -> (element=w1367:T2)
            n726 = Index Array(array=w1349, index=w1348) -> (element=w1347:bool)
            n727 = Unbundle By Name(w1368) -> ("Ref Y"=w1358:refnum<vi>, "Ref X"=w1357:refnum<vi>)
            n728 = Unbundle By Name(w1367) -> ("Invert Direction Y"=w1359:bool, "Invert Axis"=w1362:bool, "Stepsize"=w1345:dbl, "enable feedback"=w1356:bool)
            n729 = Greater Or Equal To 0?(x=w1361) -> (x >= 0?=w1360:bool)
            n730 = call <vilib>:"Add State(s) to Queue__jki_lib_state_machine.vi"("State(s) in Front (\"\")"="Wait" ("State(s) in Front (\"\")"), "State(s) in (\"\")"=w1373) -> ("States Out"=w1372:string)  [unwired: 13 in]
            n731 = property on="Speedmode @" class="DigNum (strict)"() -> ("Value"=w1344:dbl)  [unwired: 2 in, 2 out]
            n732 = Multiply(x=w1344, y=w1345) -> (x*y=w1343:dbl)
            n733 = Select(t=w1343, s=w1347, f=w1345) -> (s? t:f=w1346:dbl)
            n734 = case shown="True" w1356 {
              tunnel: w1362 -> [_ w1389]
              tunnel: w1360 -> [_ w1388]
              tunnel: w1346 -> [_ w1387]
              tunnel: w1359 -> [_ w1386]
              tunnel: w1358 -> [_ w1385]
              tunnel: w1357 -> [_ w1384]
              frame False {
              }
              frame True {
                n735 = case shown="True" w1388 {
                  tunnel: w1386 -> [w1397 w1419]
                  tunnel: w1387 -> [w1395 w1417]
                  tunnel: w1389 -> [w1394 w1416]
                  tunnel: w1389 -> [w1393 w1415]
                  tunnel: w1385 -> [w1391 w1413]
                  tunnel: w1384 -> [w1390 w1412]
                  frame True {
                    n736 = case shown="False" w1394 {
                      tunnel: [w1408 w1410] -> w1396
                      tunnel: w1391 -> [w1409 _]
                      tunnel: w1390 -> [_ w1411]
                      frame False {
                        n737 = property class="DigNum (strict)"(reference=w1409) -> ("Value"=w1408:dbl)  [unwired: 1 in, 2 out]
                      }
                      frame True {
                        n738 = property class="DigNum (strict)"(reference=w1411) -> ("Value"=w1410:dbl)  [unwired: 1 in, 2 out]
                      }
                    }
                    n739 = case shown="False" w1397 {
                      tunnel: w1396 -> [w1404 w1407]
                      tunnel: w1395 -> [w1403 w1406]
                      tunnel: [w1402 w1405] -> w1392
                      frame False {
                        n740 = Add(x=w1404, y=w1403) -> (x+y=w1402:dbl)
                      }
                      frame True {
                        n741 = Subtract(x=w1407, y=w1406) -> (x-y=w1405:dbl)
                      }
                    }
                    n742 = case shown="False" w1393 {
                      tunnel: w1392 -> [w1398 w1400]
                      tunnel: w1391 -> [w1399 _]
                      tunnel: w1390 -> [_ w1401]
                      frame False {
                        n743 = property class="DigNum (strict)"(reference=w1399, "Val(Sgnl)"=w1398) -> ()  [unwired: 1 in, 2 out]
                      }
                      frame True {
                        n744 = property class="DigNum (strict)"(reference=w1401, "Val(Sgnl)"=w1400) -> ()  [unwired: 1 in, 2 out]
                      }
                    }
                  }
                  frame False {
                    n745 = case shown="False" w1416 {
                      tunnel: [w1430 w1432] -> w1418
                      tunnel: w1413 -> [w1431 _]
                      tunnel: w1412 -> [_ w1433]
                      frame False {
                        n746 = property class="DigNum (strict)"(reference=w1431) -> ("Value"=w1430:dbl)  [unwired: 1 in, 2 out]
                      }
                      frame True {
                        n747 = property class="DigNum (strict)"(reference=w1433) -> ("Value"=w1432:dbl)  [unwired: 1 in, 2 out]
                      }
                    }
                    n748 = case shown="False" w1419 {
                      tunnel: w1418 -> [w1426 w1429]
                      tunnel: w1417 -> [w1425 w1428]
                      tunnel: [w1424 w1427] -> w1414
                      frame False {
                        n749 = Subtract(x=w1426, y=w1425) -> (x-y=w1424:dbl)
                      }
                      frame True {
                        n750 = Add(x=w1429, y=w1428) -> (x+y=w1427:dbl)
                      }
                    }
                    n751 = case shown="False" w1415 {
                      tunnel: w1414 -> [w1420 w1422]
                      tunnel: w1413 -> [w1421 _]
                      tunnel: w1412 -> [_ w1423]
                      frame False {
                        n752 = property class="DigNum (strict)"(reference=w1421, "Val(Sgnl)"=w1420) -> ()  [unwired: 1 in, 2 out]
                      }
                      frame True {
                        n753 = property class="DigNum (strict)"(reference=w1423, "Val(Sgnl)"=w1422) -> ()  [unwired: 1 in, 2 out]
                      }
                    }
                  }
                }
              }
            }
            "Arguments Y" <- w1350
            "Moving Y" <- w1350
          }
          frame "Wait" {
            # "Your code here.\n(You can make a copy of, or modify, this frame)"
            n754 = flat-sequence {
              frame #0 {
                n755 = Wait (ms)(milliseconds to wait=u32 300) -> ()  [unwired: 1 out]
              }
              frame #1 {
                n756 = property on="Moving Y" class="Str"("Value"="") -> ()  [unwired: 2 in, 2 out]
                n757 = property on="Moving X" class="Str"("Value"="") -> ()  [unwired: 2 in, 2 out]
              }
            }
            n758 = call <vilib>:"Add State(s) to Queue__jki_lib_state_machine.vi"("State(s) in (\"\")"=w1439) -> ("States Out"=w1438:string)  [unwired: 14 in]
            n759 = local read "Mean Centroid X"() -> (w1434:dbl[][])
            n760 = Bundle By Name(cluster=w1436, "Mean Centroid X"=w1434, "Mean Centroid Y"=w1434) -> (w1435:T36)
          }
          frame "stats" {
            # "Your code here.\n(You can make a copy of, or modify, this frame)"
            n761 = Unbundle By Name(w1448) -> ("Offset X"=w1447:dbl[][], "Offset Y"=w1446:dbl[][], "Time"=w1445:timestamp[][], "Motor X"=w1444:dbl[][], "Motor Y"=w1443:dbl[][])
            n762 = for {
              tunnel: w1446 -> [w1486]
              tunnel: w1445 -> [w1487]
              tunnel: w1447 -> [w1488]
              tunnel: [w1491] -> w1474 mode=indexing
              tunnel: w1444 -> [w1485]
              tunnel: w1443 -> [w1484]
              tunnel: w1449 -> [_] mode=indexing
              i -> [w1478]
              n763 = Index Array(array=w1486, index (row)=w1478) -> (element=w1482:dbl[])  [unwired: 1 in]
              n764 = Index Array(array=w1485, index (row)=w1478) -> (element=w1480:dbl[])  [unwired: 1 in]
              n765 = Index Array(array=w1484, index (row)=w1478) -> (element=w1479:dbl[])  [unwired: 1 in]
              n766 = Index Array(array=w1488, index (row)=w1478) -> (element=w1483:dbl[])  [unwired: 1 in]
              n767 = Index Array(array=w1487, index (row)=w1478) -> (element=w1481:timestamp[])  [unwired: 1 in]
              n768 = Bundle("Time"=w1481, "Motor X"=w1480) -> (w1490:cluster{"Time":timestamp[], "Motor X":dbl[]})  [unwired: 1 in]
              n769 = Bundle("Time"=w1481, "Motor Y"=w1479) -> (w1489:cluster{"Time":timestamp[], "Motor Y":dbl[]})  [unwired: 1 in]
              n770 = Bundle("Time"=w1481, "Offset X"=w1483) -> (w1492:cluster{"Time":timestamp[], "Offset X":dbl[]})  [unwired: 1 in]
              n771 = Bundle("Time"=w1481, "Offset Y"=w1482) -> (w1493:cluster{"Time":timestamp[], "Offset Y":dbl[]})  [unwired: 1 in]
              n772 = Build Array(w1493, w1492, w1490, w1489) -> (w1491:cluster{"Time":timestamp[], "Motor Y":dbl[]}[])
            }
            n773 = call <vilib>:"Add State(s) to Queue__jki_lib_state_machine.vi"("State(s) in (\"\")"=w1477) -> ("States Out"=w1476:string)  [unwired: 14 in]
            n774 = Index Array(array=w1474, index (row) #1=0 ("index (row)"), index (row) #2=1 ("index (row)"), index (row) #3=2 ("index (row)"), index (row) #4=3 ("index (row)"), index (row) #5=4 ("index (row)"), index (row) #6=5 ("index (row)"), index (row) #7=6 ("index (row)"), index (row) #8=7 ("index (row)"), index (row) #9=8 ("index (row)"), index (row) #10=9 ("index (row)"), index (row) #11=10 ("index (row)"), index (row) #12=11 ("index (row)")) -> (element #1=→"CCD 1":cluster{"Time":timestamp[], "Motor Y":dbl[]}[], element #2=→"CCD 2":cluster{"Time":timestamp[], "Motor Y":dbl[]}[], element #3=→"CCD 3":cluster{"Time":timestamp[], "Motor Y":dbl[]}[], element #4=→"CCD 4":cluster{"Time":timestamp[], "Motor Y":dbl[]}[], element #5=→"CCD 5":cluster{"Time":timestamp[], "Motor Y":dbl[]}[], element #6=→"CCD 6":cluster{"Time":timestamp[], "Motor Y":dbl[]}[], element #7=→"CCD 7":cluster{"Time":timestamp[], "Motor Y":dbl[]}[], element #8=→"CCD 8":cluster{"Time":timestamp[], "Motor Y":dbl[]}[], element #9=→"CCD 9":cluster{"Time":timestamp[], "Motor Y":dbl[]}[], element #10=→"CCD 10":cluster{"Time":timestamp[], "Motor Y":dbl[]}[], element #11=→"CCD 11":cluster{"Time":timestamp[], "Motor Y":dbl[]}[], element #12=→"CCD 12":cluster{"Time":timestamp[], "Motor Y":dbl[]}[])  [unwired: 12 in]
          }
          frame "---------------Statistics--------------" {
            # "Template Separator\n(You can make a copy of, or modify, this frame)"
            n775 = call <vilib>:"Add State(s) to Queue__jki_lib_state_machine.vi"("State(s) in (\"\")"=w1497) -> ("States Out"=w1496:string)  [unwired: 14 in]
          }
          frame "Save Stats" {
            # "Your code here.\n(You can make a copy of, or modify, this frame)"
            n776 = property on="CCD 1" class="XYGraph (strict)"() -> ("Value"=w1507:cluster{timestamp[], dbl[]}[])  [unwired: 2 in, 2 out]
            n777 = property on="CCD 2" class="XYGraph (strict)"() -> ("Value"=w1506:cluster{timestamp[], dbl[]}[])  [unwired: 2 in, 2 out]
            n778 = property on="CCD 3" class="XYGraph (strict)"() -> ("Value"=w1505:cluster{timestamp[], dbl[]}[])  [unwired: 2 in, 2 out]
            n779 = property on="CCD 4" class="XYGraph (strict)"() -> ("Value"=w1504:cluster{timestamp[], dbl[]}[])  [unwired: 2 in, 2 out]
            n780 = property on="CCD 5" class="XYGraph (strict)"() -> ("Value"=w1503:cluster{timestamp[], dbl[]}[])  [unwired: 2 in, 2 out]
            n781 = property on="CCD 6" class="XYGraph (strict)"() -> ("Value"=w1502:cluster{timestamp[], dbl[]}[])  [unwired: 2 in, 2 out]
            n782 = property on="CCD 7" class="XYGraph (strict)"() -> ("Value"=w1501:cluster{timestamp[], dbl[]}[])  [unwired: 2 in, 2 out]
            n783 = property on="CCD 8" class="XYGraph (strict)"() -> ("Value"=w1500:cluster{timestamp[], dbl[]}[])  [unwired: 2 in, 2 out]
            n784 = Build Array(w1507, w1506, w1505, w1504, w1503, w1502, w1501, w1500) -> (w1499:cluster{timestamp[], dbl[]}[][])
            n785 = for {
              tunnel: w1499 -> [w1515] mode=indexing
              tunnel: w1498 -> [w1514] mode=indexing
              n786 = Empty String/Path?(string/path=w1514) -> (empty?=w1513:bool)
              n787 = case shown="False" w1513 {
                tunnel: w1515 -> [w1521 _]
                tunnel: w1514 -> [w1519 _]
                frame False {
                  n788 = Index Array(array=w1521, index #1=0 ("index"), index #2=1 ("index"), index #3=2 ("index"), index #4=3 ("index")) -> (element #1=w1556:cluster{timestamp[], dbl[]}, element #2=w1550:cluster{timestamp[], dbl[]}, element #3=w1549:cluster{timestamp[], dbl[]}, element #4=w1548:cluster{timestamp[], dbl[]})  [unwired: 1 in, 1 out]
                  n789 = Concatenate Strings(w1519, ".dat" ("string")) -> (w1517:string)
                  n790 = Unbundle(w1556) -> (w1555:timestamp[], w1533:dbl[])
                  n791 = Unbundle(w1550) -> (w1524:dbl[])  [unwired: 1 out]
                  n792 = Unbundle(w1549) -> (w1523:dbl[])  [unwired: 1 out]
                  n793 = Unbundle(w1548) -> (w1522:dbl[])  [unwired: 1 out]
                  n794 = Build Path(base path="save path", name or relative path=w1517) -> (appended path=w1516:path)
                  n795 = for {
                    tunnel: w1555 -> [w1558] mode=indexing
                    tunnel: [w1557] -> w1531 mode=indexing
                    n796 = Format Date/Time String(time format string (%c)="%Y%m%d%H%M%S", seconds (now)=w1558) -> (date/time string=w1557:string)  [unwired: 1 in]
                  }
                  n797 = Array Size(array=w1533) -> (size(s)=w1534:i32)
                  n798 = Number To Fractional String(number=w1533) -> (F-format string=w1530:string[])  [unwired: 3 in]
                  n799 = Number To Fractional String(number=w1524) -> (F-format string=w1527:string[])  [unwired: 3 in]
                  n800 = Number To Fractional String(number=w1523) -> (F-format string=w1526:string[])  [unwired: 3 in]
                  n801 = Number To Fractional String(number=w1522) -> (F-format string=w1525:string[])  [unwired: 3 in]
                  n802 = Initialize Array("", w1534, 5 ("dimension size")) -> (w1532:string[][])
                  n803 = Insert Into Array(array=w1532, index (col)=0 ("disabled index (col)"), new element=w1531) -> (w1542:string[][])  [unwired: 1 in]
                  n804 = Insert Into Array(array=w1542, index (col)=1 ("disabled index (col)"), new element=w1530) -> (w1541:string[][])  [unwired: 1 in]
                  n805 = Insert Into Array(array=w1541, index (col)=2 ("disabled index (col)"), new element=w1527) -> (w1545:string[][])  [unwired: 1 in]
                  n806 = Insert Into Array(array=w1545, index (col)=3 ("disabled index (col)"), new element=w1526) -> (w1546:string[][])  [unwired: 1 in]
                  n807 = Insert Into Array(array=w1546, index (col)=4 ("disabled index (col)"), new element=w1525) -> (w1547:string[][])  [unwired: 1 in]
                  n808 = Insert Into Array(array=w1547, index (row)=0, new element=string[] ["time", "Centroid X", "Centroid Y", "Motor Axis 1", "Motor Axis 2"] ("new element/subarray 2")) -> (w1529:string[][])  [unwired: 1 in]
                  n809 = call-poly <vilib>:"Write To Spreadsheet File.vi"("2D data"=w1529, "file path (dialog if empty)"=w1516) -> ()  [unwired: 6 in, 1 out]
                }
                frame True {
                }
              }
            }
            n810 = call <vilib>:"Add State(s) to Queue__jki_lib_state_machine.vi"("State(s) in (\"\")"=w1512) -> ("States Out"=w1511:string)  [unwired: 14 in]
            n811 = property on="Save Stats" class="Bool (strict)"("Value"=FALSE ("Save Stats")) -> ()  [unwired: 2 in, 2 out]
          }
          frame "tdms" {
            w1583 = 21600.0 ("new tdms")
            # "Your code here.\n(You can make a copy of, or modify, this frame)"
            n812 = Unbundle By Name(w1572) -> ("Data Value Reference out"=w1597:refnum<k34>, "Offset X"=w1599:dbl[][], "Offset Y"=w1594:dbl[][], "active axis refs 2"=w1596:T12)
            n813 = for {
              tunnel: w1599 -> [w1643]
              tunnel: w1594 -> [w1642]
              tunnel: w1598 -> [w1606] mode=indexing
              tunnel: w1597 -> [w1607]
              tunnel: w1596 -> [w1628]
              tunnel: w1595 -> [w1612]
              tunnel: [w1610] -> w1593
              i -> [w1629]
              n814 = Index Array(array=w1643, index (row)=w1629) -> (element=w1641:dbl[])  [unwired: 1 in]
              n815 = Index Array(array=w1642, index (row)=w1629) -> (element=w1640:dbl[])  [unwired: 1 in]
              n816 = Index Array(array=w1628, index=w1629) -> (element=w1627:cluster{"Ref X":refnum<vi>, "Ref Y":refnum<vi>})
              n817 = Reverse 1D Array(array=w1640) -> (reversed array=w1638:dbl[])
              n818 = Reverse 1D Array(array=w1641) -> (reversed array=w1639:dbl[])
              n819 = Unbundle By Name(w1627) -> ("Ref X"=w1626:refnum<vi>, "Ref Y"=w1625:refnum<vi>)
              n820 = Index Array(array=w1639) -> (element=w1637:dbl)  [unwired: 1 in]
              n821 = Index Array(array=w1638) -> (element=w1636:dbl)  [unwired: 1 in]
              n822 = property class="DigNum (strict)"(reference=w1626, error in=w1612) -> (error out=w1611:errorcluster, "Value"=w1620:dbl)  [unwired: 1 out]
              n823 = Build Array(w1637) -> (w1609:dbl[])
              n824 = Build Array(w1636) -> (w1631:dbl[])
              n825 = Get Date/Time In Seconds() -> (seconds since 1Jan1904=w1608:timestamp)
              n826 = Build Array(w1608) -> (w1604:timestamp[])
              n827 = property class="DigNum (strict)"(reference=w1625, error in=w1611) -> (error out=w1602:errorcluster, "Value"=w1614:dbl)  [unwired: 1 out]
              n828 = Build Array(w1620) -> (w1619:dbl[])
              n829 = TDMS Write(0:w1607, 5:w1606, 7:"time", 9:w1604, 11:w1602) -> (4:w1603:refnum<k34>, 15:w1601:errorcluster)  [unwired: 1 in, 2 out]
              n830 = Build Array(w1614) -> (w1613:dbl[])
              n831 = TDMS Write(0:w1603, 5:w1606, 7:"centroid X", 9:w1609, 11:w1601) -> (4:w1634:refnum<k34>, 6:w1633:string, 15:w1632:errorcluster)  [unwired: 1 in, 1 out]
              n832 = TDMS Write(0:w1634, 5:w1633, 7:"centroid Y", 9:w1631, 11:w1632) -> (4:w1623:refnum<k34>, 6:w1622:string, 15:w1624:errorcluster)  [unwired: 1 in, 1 out]
              n833 = TDMS Write(0:w1623, 5:w1622, 7:"Motor Axis 1", 9:w1619, 11:w1624) -> (4:w1618:refnum<k34>, 6:w1617:string, 15:w1615:errorcluster)  [unwired: 1 in, 1 out]
              n834 = TDMS Write(0:w1618, 5:w1617, 7:"Motor Axis 2", 9:w1613, 11:w1615) -> (15:w1610:errorcluster)  [unwired: 1 in, 3 out]
            }
            n835 = Unbundle By Name(w1572) -> ("img to avg"=w1570:i32)
            n836 = property on="millisecond timer value" class="DigNum (strict)"() -> ("Value"=w1573:u32)  [unwired: 2 in, 2 out]
            n837 = local read "millisecond timer 2"() -> (w1589:u32)
            n838 = Tick Count (ms)() -> (millisecond timer value=w1574:u32)
            n839 = call <userlib>:"Tick Count (ms)__ogtk.vi"("error in (no error)"=w1593) -> ("error out"=w1590:errorcluster, "millisecond timer value"=w1592:u32)  [unwired: 9 in]
            n840 = Subtract(x=w1574, y=w1573) -> (x-y=w1588:u32)
            n841 = Subtract(x=w1574, y=w1573) -> (x-y=w1575:u32)
            n842 = Subtract(x=w1592, y=w1589) -> (x-y=→"Waveform Chart":u32)
            n843 = Multiply(x=5.0 ("new tdms"), y=w1570) -> (x*y=w1568:dbl)
            n844 = Divide(x=w1588, y=u32 1000) -> (x/y=w1586:dbl)
            n845 = Divide(x=w1575, y=u32 1000) -> (x/y=w1577:dbl)
            n846 = Quotient & Remainder(x=w1586, y=w1583) -> (x-y*floor(x/y)=w1585:dbl)  [unwired: 1 out]
            n847 = Quotient & Remainder(x=w1577, y=w1568) -> (x-y*floor(x/y)=w1569:dbl)  [unwired: 1 out]
            "x-y*floor(x/y)" <- w1569
            n848 = Subtract(x=w1568, y=2.0) -> (x-y=w1566:dbl)
            n849 = Greater?(x=w1569, y=w1566) -> (0:w1565:bool)
            n850 = Subtract(x=w1583, y=20.0) -> (x-y=w1581:dbl)
            n851 = Greater?(x=w1585, y=w1581) -> (0:w1584:bool)
            n852 = Select(t="Device Ini", s=w1565, f="") -> (s? t:f=w1562:string)
            n853 = Select(t="newtdms", s=w1584, f="") -> (s? t:f=w1578:string)
            n854 = call <vilib>:"Add State(s) to Queue__jki_lib_state_machine.vi"("State(s) in (\"\")"=w1600, "State(s) at Back (\"\")"=w1578) -> ("States Out"=w1561:string)  [unwired: 13 in]
            n855 = call <vilib>:"Add State(s) to Queue__jki_lib_state_machine.vi"("State(s) in Front (\"\")"=w1562, "State(s) in (\"\")"=w1561) -> ("States Out"=w1560:string)  [unwired: 13 in]
          }
          frame "Reset History" {
            # "Your code here.\n(You can make a copy of, or modify, this frame)"
            n856 = for {
              N: 1 -> [_]
              shift-right: [w1653] -> w1645
              shift-left: timestamp[][] [] ("Time") -> [w1655]
              n857 = for {
                N: 12 -> [_]
                tunnel: w1655 -> [w1658] mode=indexing
                tunnel: [w1656] -> w1653 mode=indexing
                n858 = Get Date/Time In Seconds() -> (seconds since 1Jan1904=w1657:timestamp)
                n859 = Build Array (concatenate)(w1658, w1657) -> (w1656:timestamp[])
              }
            }
            n860 = local read "Offset X"() -> (w1644:dbl[][])
            n861 = Bundle By Name(cluster=w1649, "Offset X"=w1644, "Offset Y"=w1644, "Time"=w1645, "Motor X"=w1644) -> (w1648:T36)
            n862 = call <vilib>:"Add State(s) to Queue__jki_lib_state_machine.vi"("State(s) in (\"\")"=w1652) -> ("States Out"=w1651:string)  [unwired: 14 in]
          }
          frame "New Category: 2" {
            # "Your code here.\n(You can make a copy of, or modify, this frame)"
            n863 = call <vilib>:"Add State(s) to Queue__jki_lib_state_machine.vi"("State(s) in (\"\")"=w1662) -> ("States Out"=w1661:string)  [unwired: 14 in]
          }
          frame "ImgToAvg" {
            # "Your code here.\n(You can make a copy of, or modify, this frame)"
            n864 = Decimal String To Number(string=w1666) -> (number=w1663:i32)  [unwired: 2 in, 1 out]
            n865 = Bundle By Name(cluster=w1665, "img to avg"=w1663) -> (w1664:T36)
            n866 = call <vilib>:"Add State(s) to Queue__jki_lib_state_machine.vi"("State(s) in (\"\")"=w1669) -> ("States Out"=w1668:string)  [unwired: 14 in]
          }
          frame "newtdms" {
            # "Your code here.\n(You can make a copy of, or modify, this frame)"
            n867 = Unbundle By Name(w1680) -> ("Data Value Reference out"=w1679:refnum<k34>)
            n868 = TDMS Close(8:w1678, 11:w1679) -> (0:w1671:errorcluster)  [unwired: 1 out]
            n869 = call <vilib>:"Clear Errors.vi"("error in (no error)"=w1671) -> ("error out"=w1670:errorcluster)  [unwired: 6 in]
            n870 = Get Date/Time In Seconds() -> (seconds since 1Jan1904=w1691:timestamp)
            n871 = Format Date/Time String(time format string (%c)="%Y%m%d%H%M", seconds (now)=w1691) -> (date/time string=w1682:string)  [unwired: 1 in]
            n872 = Concatenate Strings(w1682, "Beampointing_Pico.tdms" ("string")) -> (w1688:string)
            n873 = String To Path(string=w1688) -> (path=w1689:path)
            n874 = Build Path(base path=w1672, name or relative path=w1689) -> (appended path=w1683:path)
            n875 = TDMS Open(6:FALSE ("disable buffering (T)"), 7:enum16{"1.0", "2.0"}."2.0" ("file format version (2.0)"), 8:w1670, 10:T17."create or replace" ("operation"), 11:w1683) -> (0:w1674:errorcluster, 3:w1677:refnum<k34>)  [unwired: 2 in]
            n876 = call "TDMSbuffersize.vi"("error in (no error)"=w1674, "group names"=w1676, "Data Value Reference in"=w1677) -> ("error out"=w1673:errorcluster, "Data Value Reference out"=w1675:refnum<k34>)  [unwired: 7 in]
            n877 = call <vilib>:"Add State(s) to Queue__jki_lib_state_machine.vi"("State(s) in (\"\")"=w1693) -> ("States Out"=w1692:string)  [unwired: 14 in]
            n878 = Bundle By Name(cluster=w1680, "Data Value Reference out"=w1675) -> (w1681:T36)
          }
          frame "Center" {
            # "Your code here.\n(You can make a copy of, or modify, this frame)"
            n879 = property on="Center" class="Bool (strict)"("Value"=FALSE ("Center")) -> ()  [unwired: 2 in, 2 out]
            n880 = control-ref of="image::1"() -> (w1708:refnum<vi>)
            n881 = control-ref of="image::2"() -> (w1707:refnum<vi>)
            n882 = control-ref of="image::3"() -> (w1706:refnum<vi>)
            n883 = control-ref of="image::4"() -> (w1705:refnum<vi>)
            n884 = control-ref of="image::5"() -> (w1704:refnum<vi>)
            n885 = control-ref of="image::6"() -> (w1703:refnum<vi>)
            n886 = control-ref of="image::7"() -> (w1702:refnum<vi>)
            n887 = control-ref of="image::8"() -> (w1701:refnum<vi>)
            n888 = control-ref of="image::9"() -> (w1700:refnum<vi>)
            n889 = control-ref of="image::10"() -> (w1699:refnum<vi>)
            n890 = control-ref of="image::11"() -> (w1698:refnum<vi>)
            n891 = control-ref of="image::12"() -> (w1697:refnum<vi>)
            n892 = for {
              tunnel: w1694 -> [w1721] mode=indexing
              tunnel: [w1716] -> w1709 mode=indexing
              n893 = Unbundle By Name(w1721) -> ("Target.X::12"=w1720:refnum<vi>, "Target.Y::12"=w1719:refnum<vi>)
              n894 = property class="DigNum (strict)"(reference=w1720) -> ("Value"=w1718:dbl)  [unwired: 1 in, 2 out]
              n895 = property class="DigNum (strict)"(reference=w1719) -> ("Value"=w1717:dbl)  [unwired: 1 in, 2 out]
              n896 = Bundle("Value"=w1718, "Value"=w1717) -> (w1716:cluster{"Value":dbl, "Value":dbl})  [unwired: 1 in]
            }
            n897 = call <vilib>:"Add State(s) to Queue__jki_lib_state_machine.vi"("State(s) in (\"\")"=w1713) -> ("States Out"=w1712:string)  [unwired: 14 in]
            n898 = Build Array(w1708, w1707, w1706, w1705, w1704, w1703, w1702, w1701, w1700, w1699, w1698, w1697) -> (w1696:refnum<vi>[])
            n899 = for {
              tunnel: w1696 -> [w1715] mode=indexing
              tunnel: w1709 -> [w1714] mode=indexing
              n900 = property class="ImageControl"(reference=w1715, "Image Center Position"=w1714) -> ()  [unwired: 1 in, 2 out]
            }
          }
          frame "history" {
            # "Your code here.\n(You can make a copy of, or modify, this frame)"
            n901 = Unbundle By Name(w1731) -> ("Offset X"=w1737:dbl[][], "Offset Y"=w1736:dbl[][], "Mean Centroid X"=w1735:dbl[][], "Mean Centroid Y"=w1734:dbl[][], "Motor X"=w1733:dbl[][], "Motor Y"=w1732:dbl[][], "Time"=w1723:timestamp[][])
            n902 = for {
              tunnel: w1737 -> [w1755] mode=indexing
              tunnel: w1736 -> [w1753] mode=indexing
              tunnel: w1735 -> [w1752] mode=indexing
              tunnel: w1734 -> [w1751] mode=indexing
              tunnel: w1733 -> [w1750] mode=indexing
              tunnel: w1732 -> [w1749] mode=indexing
              tunnel: [w1754] -> w1729 mode=indexing
              tunnel: [w1748] -> w1728 mode=indexing
              tunnel: [w1744] -> w1727 mode=indexing
              tunnel: [w1747] -> w1726 mode=indexing
              tunnel: [w1746] -> w1725 mode=indexing
              tunnel: [w1745] -> w1724 mode=indexing
              tunnel: w1723 -> [w1743] mode=indexing
              tunnel: [w1741] -> w1722 mode=indexing
              w1742 = 0
              n903 = Delete From Array(array=w1750, index=w1742) -> (array with subset deleted=w1746:dbl[])  [unwired: 1 in, 1 out]
              n904 = Delete From Array(array=w1749, index=w1742) -> (array with subset deleted=w1745:dbl[])  [unwired: 1 in, 1 out]
              n905 = Delete From Array(array=w1743, index=w1742) -> (array with subset deleted=w1741:timestamp[])  [unwired: 1 in, 1 out]
              n906 = Delete From Array(array=w1752, index=w1742) -> (array with subset deleted=w1744:dbl[])  [unwired: 1 in, 1 out]
              n907 = Delete From Array(array=w1751, index=w1742) -> (array with subset deleted=w1747:dbl[])  [unwired: 1 in, 1 out]
              n908 = Delete From Array(array=w1753, index=w1742) -> (array with subset deleted=w1748:dbl[])  [unwired: 1 in, 1 out]
              n909 = Delete From Array(array=w1755, index=w1742) -> (array with subset deleted=w1754:dbl[])  [unwired: 1 in, 1 out]
            }
            n910 = call <vilib>:"Add State(s) to Queue__jki_lib_state_machine.vi"("State(s) in (\"\")"=w1740) -> ("States Out"=w1739:string)  [unwired: 14 in]
            n911 = Bundle By Name(cluster=w1731, "Offset X"=w1729, "Offset Y"=w1728, "Mean Centroid X"=w1727, "Mean Centroid Y"=w1726, "Motor X"=w1725, "Motor Y"=w1724, "Time"=w1722) -> (w1730:T36)
          }
        }
        n912 = property on="Box" class="Arr (strict)"() -> ("Value"=w261:T6)  [unwired: 2 in, 2 out]
        n913 = for {
          tunnel: w263 -> [w288]
          tunnel: w262 -> [w289]
          tunnel: w254 -> [w281] mode=indexing
          tunnel: w261 -> [w282] mode=indexing
          n914 = call-poly <userlib>:"Filter 1D Array__ogtk.vi"("items to filter"=w281, "array"=w289) -> ("filtered item indices"=w290:i32[])  [unwired: 4 in, 1 out]
          n915 = Index Array(array=w290) -> (element=w284:i32)  [unwired: 1 in]
          n916 = Index Array(array=w288, index=w284) -> (element=w287:T30)
          n917 = Unbundle By Name(w287) -> ("Target.X::12"=w292:refnum<vi>, "Target.Y::12"=w291:refnum<vi>)
          n918 = property class="DigNum (strict)"(reference=w292) -> ("Value"=w286:dbl)  [unwired: 1 in, 2 out]
          n919 = property class="DigNum (strict)"(reference=w291) -> ("Value"=w285:dbl)  [unwired: 1 in, 2 out]
          n920 = call "draw crosshair imaq.vi"("Color"=u32 16774656, "Target.Y"=w285, "size"=cluster{"xhair size":dbl, "xhair size 2":dbl} {"xhair size"=25.0, "xhair size 2"=25.0}, "Target.X"=w286, "Bounding Rectangle"=T15 {"Left"=0, "Top"=0, "Right"=0, "Bottom"=0}, "image in"=w281) -> ("error out"=→"error out":errorcluster, "image out"=w280:T9)  [unwired: 4 in]
          n921 = call "draw box imaq.vi"("Color"=u32 1244928, "Rectangle"=w282, "image in"=w280) -> ()  [unwired: 8 in, 1 out]
        }
        n922 = property on="ActiveMotor" class="Ring (strict)"() -> ("Strings []"=w256:string[])  [unwired: 2 in, 2 out]
        n923 = Index Array(array=w256, index="ActiveMotor") -> (element=w257:string)
        n924 = Not Equal?(x="ActiveMotorName::99", y=w257) -> (x != y?=w258:bool)
        n925 = case shown="True" w258 {
          tunnel: w256 -> [_ w277]
          tunnel: "ActiveMotorName::99" -> [_ w276]
          frame False {
          }
          frame True {
            n926 = Search 1D Array(1D array=w277, element=w276) -> (index of element=w275:i32)  [unwired: 1 in]
            n927 = property on="ActiveMotor" class="Ring (strict)"("Value"=w275) -> ()  [unwired: 2 in, 2 out]
          }
        }
      }
      n928 = control-ref of="This Application"() -> (w243:refnum<vi>)
      n929 = control-ref of="This VI"() -> (w247:refnum<vi>)
      n930 = Current VI's Menubar() -> (w246:refnum<k9>)
      n931 = call "GUI_Master_subvi_reentrant_queues.vi"("This Application"=w243, "error in (no error)"=w244, "tcp data event"=w242, "Caller menu reference"=w246, "Caller VI ref"=w247) -> ("error out"=→"error IO 2":errorcluster)  [unwired: 6 in]
      n932 = Unbundle By Name(w132) -> ("Data Value Reference out"=w131:refnum<k34>)
      n933 = for {
        tunnel: w161 -> [w251] mode=indexing
        tunnel: w160 -> [w250]
        tunnel: [w249] -> w130
        n934 = call "IMAQ Dispose"("Image"=w251, "error in (no error)"=w250) -> ("error out"=w249:errorcluster)  [unwired: 4 in]
      }
      n935 = TDMS Close(8:w130, 11:w131) -> (0:→"error out 2":errorcluster)  [unwired: 1 out]
    }
  }
